vi "Omniax_mDrive_XYZR_MM_BR_RES_2_NC_GR_pxi_Acc2.vi"() -> ()   [LabVIEW 2009]
uses:
  <vilib>/Instr/_visa.llb/VISA Configure Serial Port (Instr).vi
panel:
  in  "Clear ZY":bool
  out "atan Y/Z":dbl
  out "ZY Graph":cluster{"Y":dbl[], "Y":dbl[]}[](graph)
  out "R Ready":bool
  out "Z Ready":bool
  out "Y Ready":bool
  out "X Ready":bool
  out "ZR Graph":cluster{"Y":dbl[], "Y":dbl[]}[](graph)
  out "XY Graph":cluster{"Y":dbl[], "Y":dbl[]}[](graph)
  out "X Scan Duration":dbl
  out "Y Scan Duration":dbl
  out "Z Scan Duration":dbl
  out "R Scan Duration":dbl
  out "R Backlash steps/sec":i32
  out "R Backlash":i32
  out "R Holding Current %":i32
  out "R Run Current %":i32
  out "R offset deg":dbl
  out "R deg/rev":dbl
  out "R steps/rev":u32
  out "R velocity PV step/sec":i32
  out "R MINPOS":i32=-94296
  out "R MAXPOS":i32=-34296
  out "R COM PORT":refnum<visa-resource-name>="COM5"
  in  "R Scan set":bool
  in  "R Scan Velocity SP deg/sec":dbl
  in  "R Scan Length SP deg":dbl
  in  "R Move Set":bool
  out "Reset R Motor Steps":i32
  in  "Reset R Position deg":dbl
  out "R Velocity MVdeg/sec":dbl
  in  "R Velocity SP deg/sec":dbl
  in  "R Position SP deg":dbl
  out "R Position MV deg":dbl
  out "R Scan velocity MV deg/sec":dbl format="%#_6f"
  out "R Scan length MV deg":dbl
  in  "R Scan Length SP steps":i32 min=-6144000 max=0 step=100
  in  "R Scan OK":bool
  in  "R Velocity SP step/sec":i32 min=1 max=20000
  in  "R Scan Velocity SP steps/sec":i32=1 min=1 max=102400 step=1
  in  "R Go":bool
  in  "R Step SP":i32=-20000 min=-6144000 max=0 step=500
  out "R Position deg PV":dbl
  out "R Step PV":i32 max=2000
  out "R Backlash corr":bool
  out "R in Motion":bool
  out "R Scan":bool
  out "R in Range":bool
  out "Z COM PORT":refnum<visa-resource-name>="COM5"
  out "Z Backlash steps/sec":i32
  out "Z Backlash":i32
  out "Z Holding Current %":i32
  out "Z Run Current %":i32
  out "Z offset mm":dbl
  out "Z mm/rev":dbl
  out "Z steps/rev":u32
  out "Z  velocity PV step/sec":i32
  out "Z MINPOS":i32=-94296
  out "Z MAXPOS":i32=-34296
  in  "Z Scan set":bool
  in  "Z Scan Velocity SP mm/sec":dbl
  in  "Z Scan Length SP mm":dbl
  in  "Z Move Set":bool
  out "Reset Z Motor Steps":i32
  in  "Reset Z Position mm":dbl
  out "Z Velocity MV mm/sec":dbl
  in  "Z Velocity SP mm/sec":dbl
  in  "Z Position SP mm":dbl
  out "Z Position MV mm":dbl
  out "Z Scan velocity MV mm/sec":dbl format="%#_6f"
  out "Z Scan length MV mm":dbl
  in  "Z Scan Length SP steps":i32 min=-11520000 max=90880000 step=100
  in  "Z Scan OK":bool
  in  "Z Velocity SP step/sec":i32 min=1 max=204800
  in  "Z Scan Velocity SP steps/sec":i32=1 min=1 max=102400 step=1
  in  "Z Go":bool
  in  "Z Step SP":i32=-20000 min=0 max=102400000 step=500
  out "Z Position mm PV":dbl
  out "Z Step PV":i32 max=2000
  out "Z Backlash corr":bool
  out "Z in Motion":bool
  out "Z Scan":bool
  out "Z in Range":bool
  out "Reset X Motor Steps":i32
  in  "Reset X Position mm":dbl
  out "X Backlash corr":bool
  out "X  in Motion":bool
  out "X Scan":bool
  out "X  in Range":bool
  out "X Step PV":i32 max=2000
  out "X Position mm PV":dbl
  out "X velocity PV step/sec":i32
  in  "X Scan set":bool
  in  "X Scan Velocity SP mm/sec":dbl
  in  "X Scan Length SP mm":dbl
  in  "X Move Set":bool
  out "X Velocity MV mm/sec":dbl
  in  "X Velocity SP mm/sec":dbl
  in  "X Position SP mm":dbl
  out "X Position MV mm":dbl
  out "X Scan velocity MV mm/sec":dbl format="%#_6f"
  out "X Scan length MV mm":dbl
  in  "X Scan Length SP steps":i32 min=-2304000 max=2304000 step=100
  in  "X Scan OK":bool
  in  "X Velocity SP step/sec":i32 min=1 max=128000
  in  "X Scan Velocity SP steps/sec":i32=1 min=1 max=102400 step=1
  in  "X Go":bool
  in  "X Step SP":i32=-20000 min=-2304000 max=2304000 step=500
  out "X Backlash steps/sec":i32
  out "X Backlash":i32
  out "X Holding Current %":i32
  out "X Run Current %":i32
  out "X offset mm":dbl
  out "X mm/rev":dbl
  out "X steps/rev":u32
  out "X MAXPOS":i32=-34296
  out "X MINPOS":i32=-94296
  out "X COM PORT":refnum<visa-resource-name>="COM5"
  out "Y Backlash corr":bool
  in  "Y Scan set":bool
  in  "Y Scan Velocity SP mm/sec":dbl
  in  "Y Scan Length SP mm":dbl
  in  "Y Move Set":bool
  out "Y Backlash steps/sec":i32
  out "Y Backlash":i32
  out "Y in Motion":bool
  in  "Reset":bool
  out "Reset Y Motor Steps":i32
  in  "Reset Y Position mm":dbl
  out "Y Velocity MV mm/sec":dbl
  in  "Y Velocity SP mm/sec":dbl
  in  "Y Position SP mm":dbl
  out "Y Position MV mm":dbl
  out "Y Holding Current %":i32
  out "Y Run Current %":i32
  out "Y Scan velocity MV mm/sec":dbl format="%#_6f"
  out "Y Scan length MV mm":dbl
  in  "Scan Cancel":bool
  out "Y Position mm PV":dbl
  out "Y offset mm":dbl
  out "Y mm/rev":dbl
  out "Y steps/rev":u32
  out "Y velocity PV step/sec":i32
  in  "Y Scan Length SP steps":i32 min=-1792000 max=2816000 step=100
  out "Y Scan":bool
  in  "Y Scan OK":bool
  in  "Scan Go":bool
  in  "Y Velocity SP step/sec":i32 min=1 max=128000
  in  "Y Scan Velocity SP steps/sec":i32=1 min=1 max=102400 step=1
  in  "Stop":bool
  out "Y in Range":bool
  out "Y Step PV":i32 max=2000
  in  "Y Go":bool
  in  "Y Step SP":i32=-20000 min=-2304000 max=2304000 step=500
  out "Y MINPOS":i32=-94296
  out "Y MAXPOS":i32=-34296
  out "Y COM PORT":refnum<visa-resource-name>="COM5"
  # "L"
  # "M"
  # "B"
  # "S"
  # "R"
  # "MX"
  # "MY"
  # "MZ"
  # "MR"
  # "MX"
  # "MY"
  # "MZ"
  # "MR"
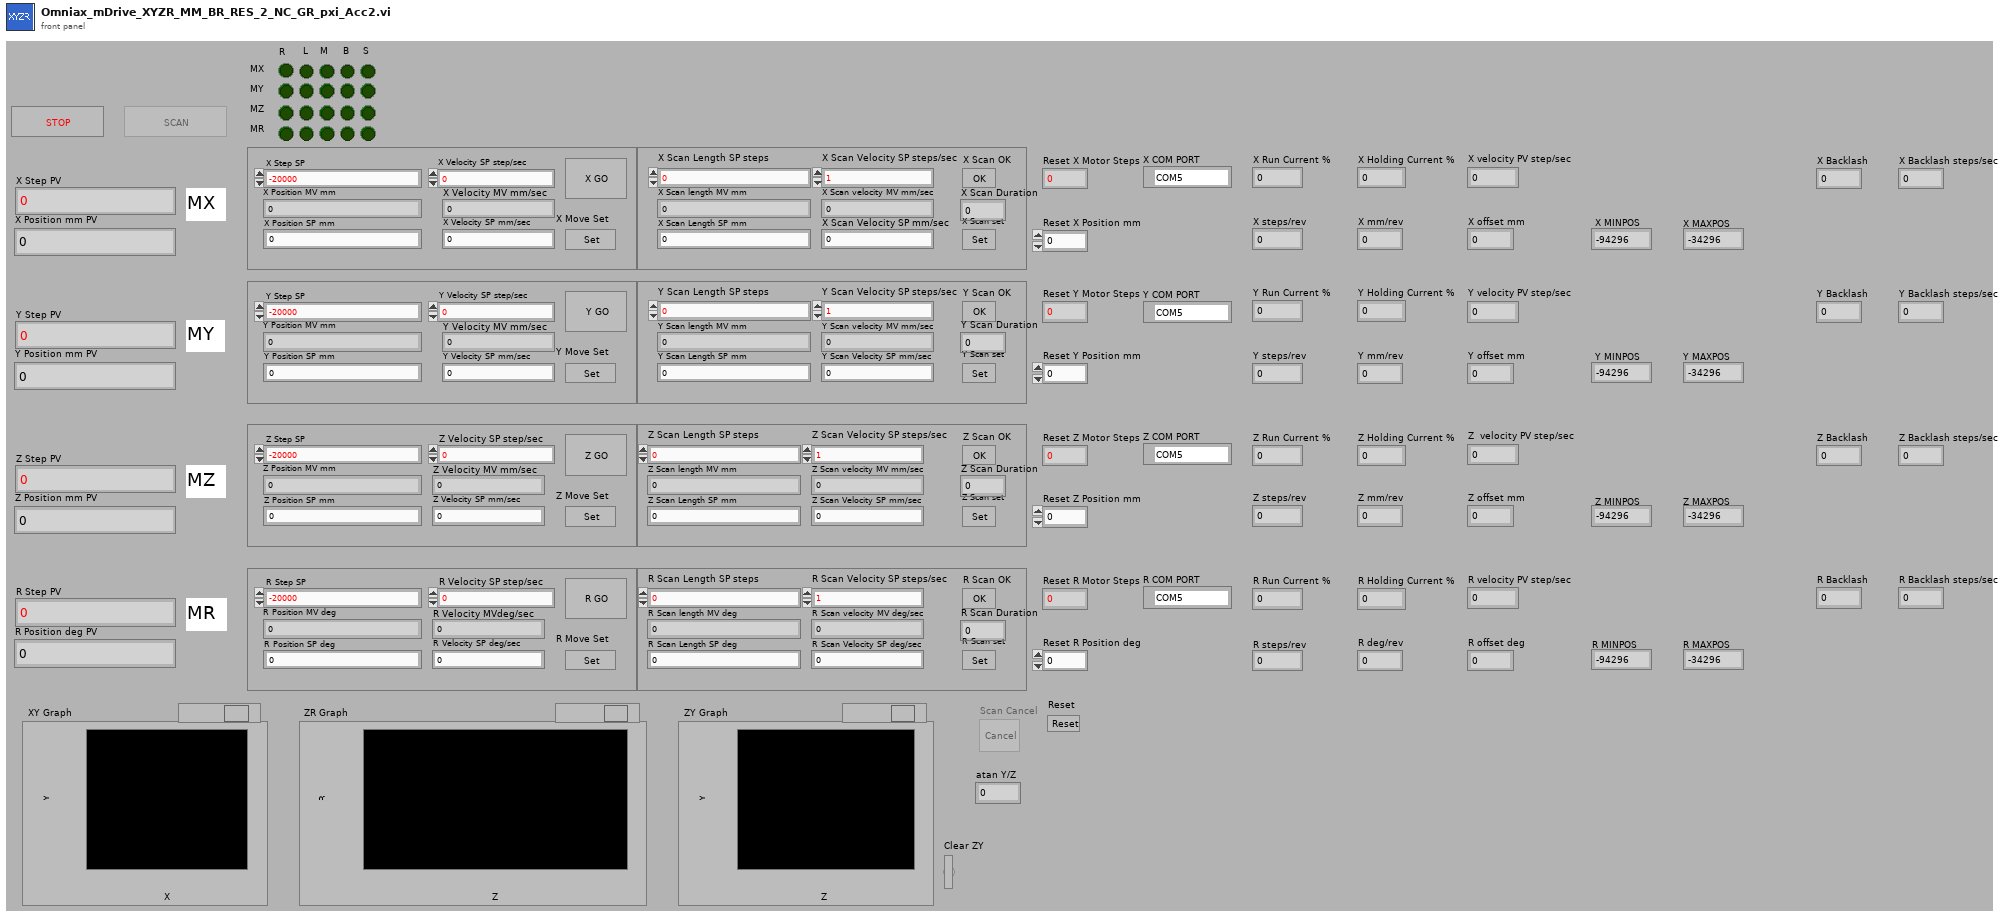
[diagram p1: front panel]
types:
  T1 = enum16{"Stop", "Reset", "Run Current", "Holding Current", "Accel Rate", "Decel Rate", "Move to Relative Position", "Move to Absolute Position", "Echo Mode", "Print Parameter", "Send String", "Microstep Resolution", "Set Current Position", "Max Velocity"}
  T2 = enum8{"Enabled", "Disabled", "Disabled and Grayed Out"}
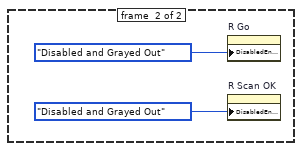
[diagram p2: hidden frame]
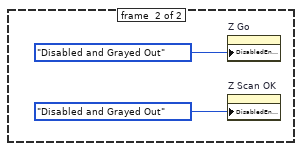
[diagram p5: hidden frame]
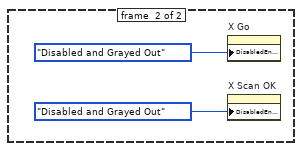
[diagram p8: hidden frame]
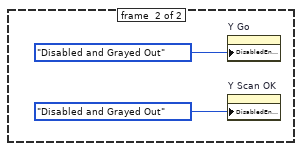
[diagram p11: hidden frame]
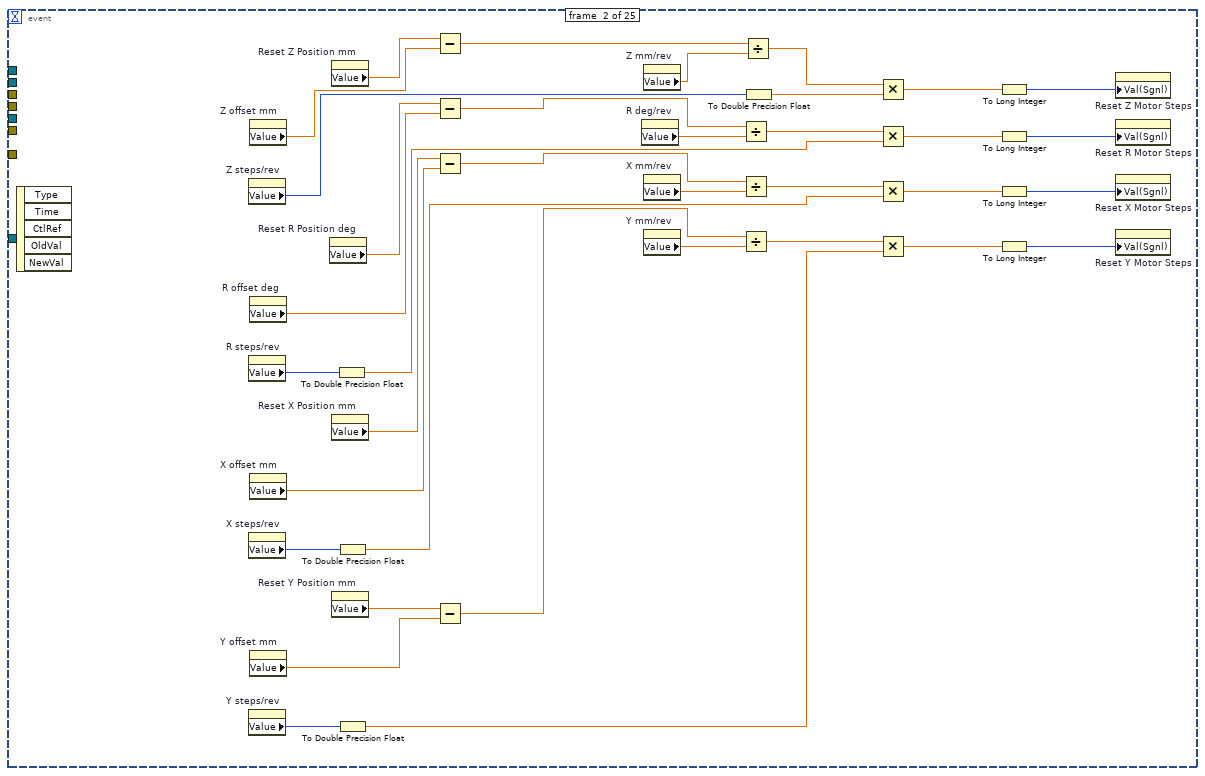
[diagram p14: hidden frame]
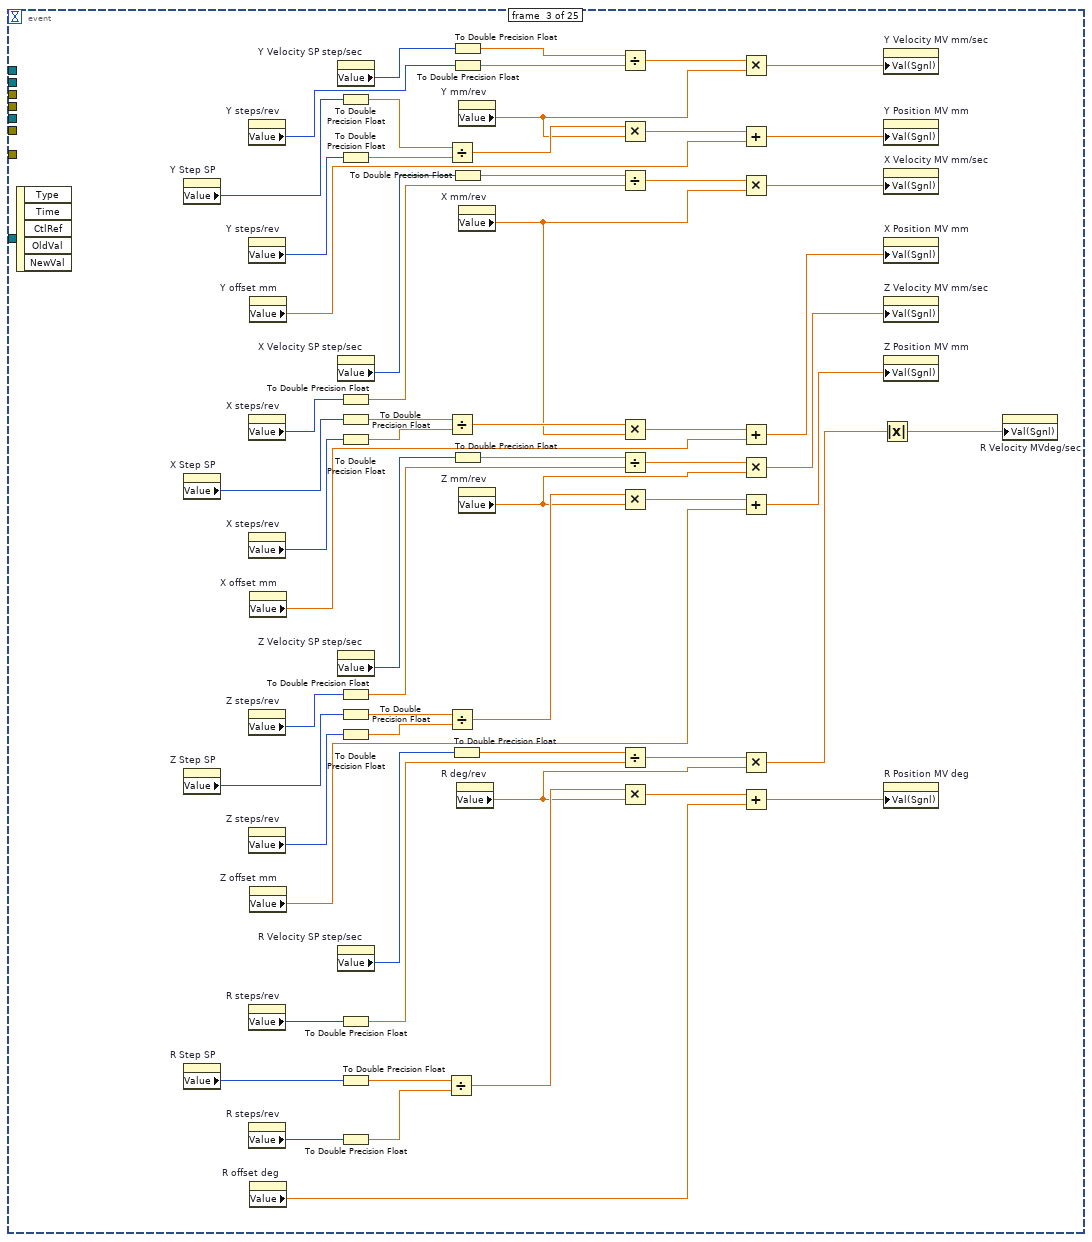
[diagram p15: hidden frame]
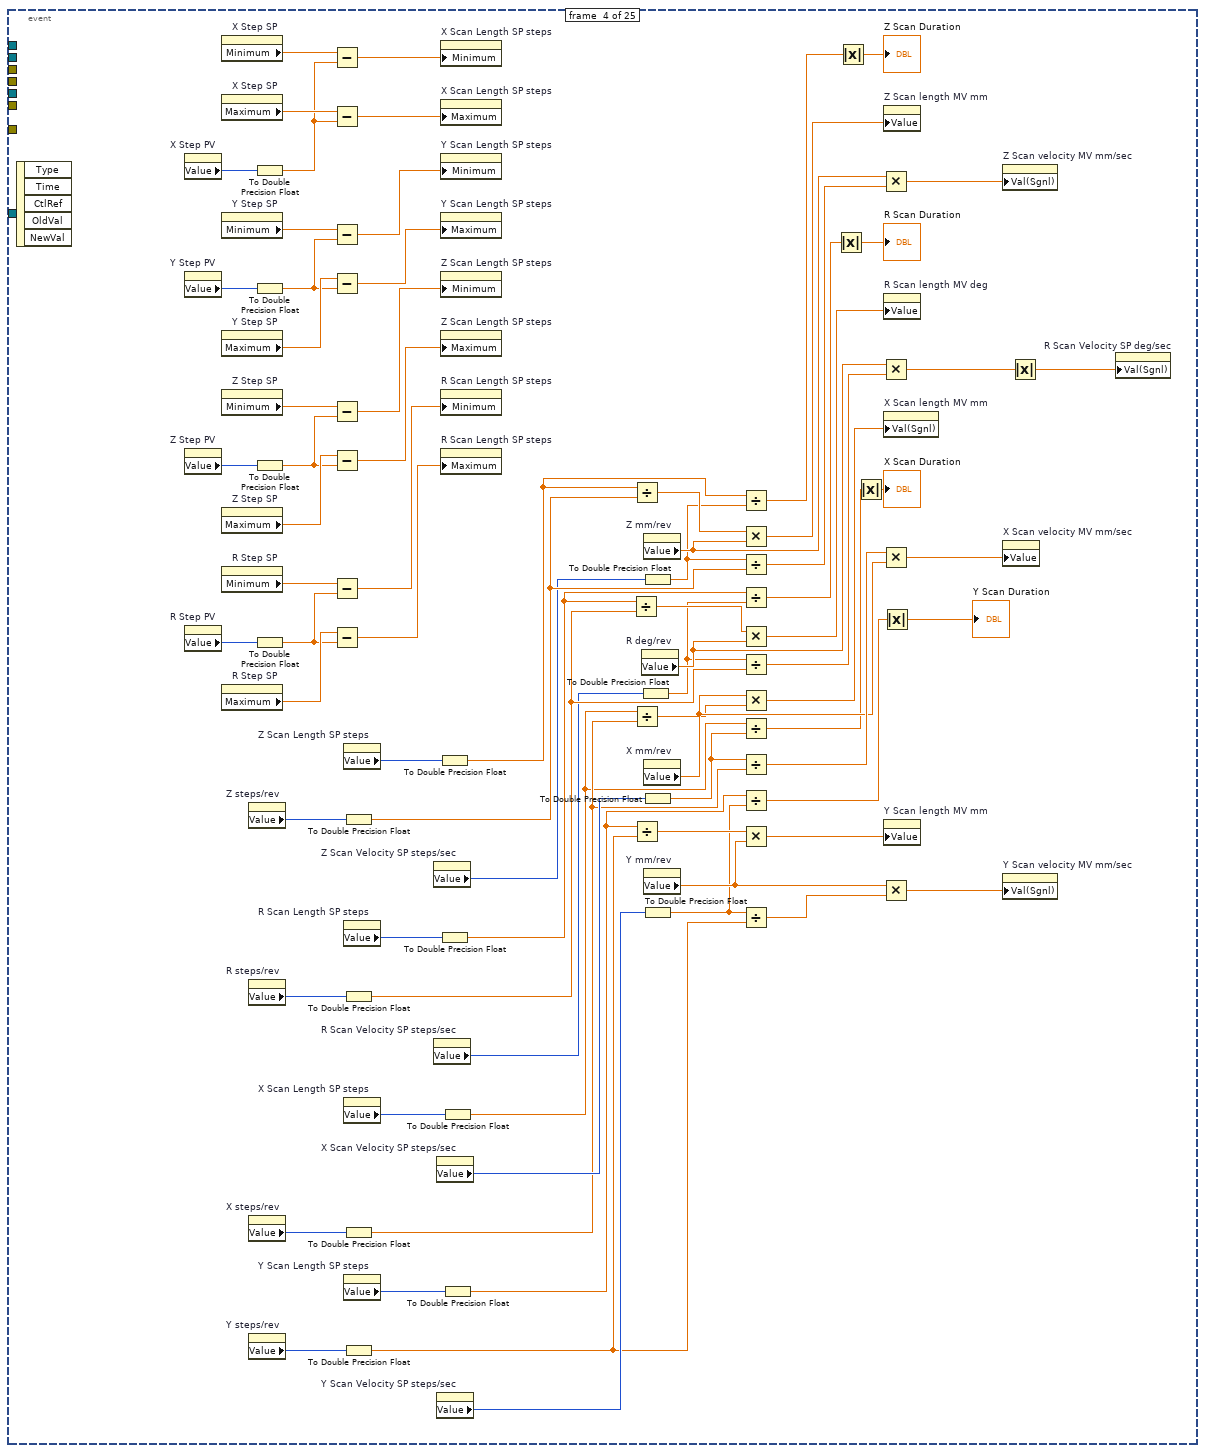
[diagram p16: hidden frame]
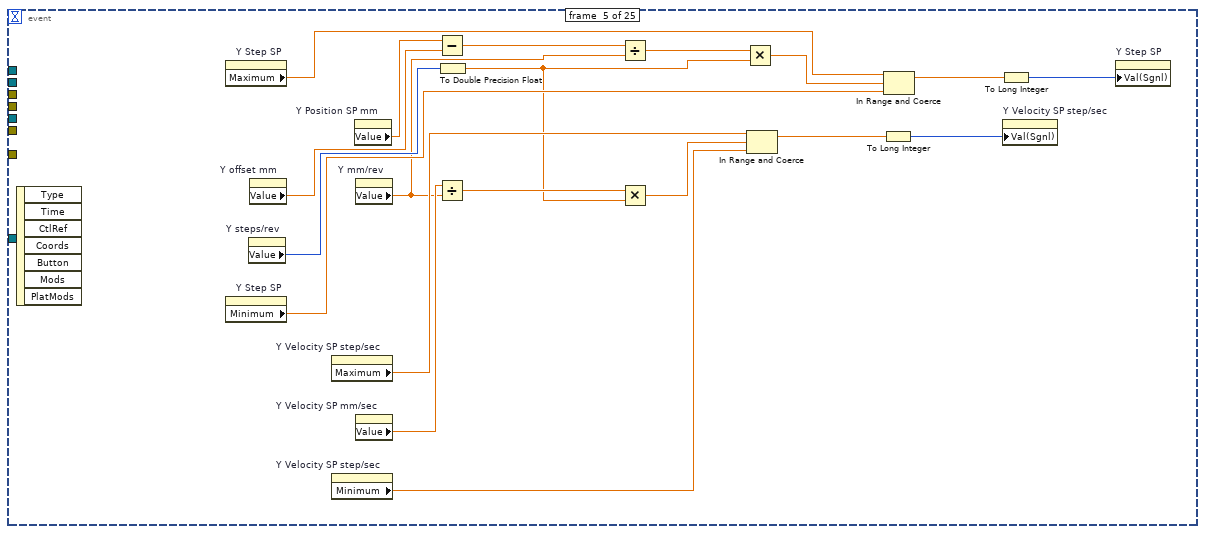
[diagram p17: hidden frame]
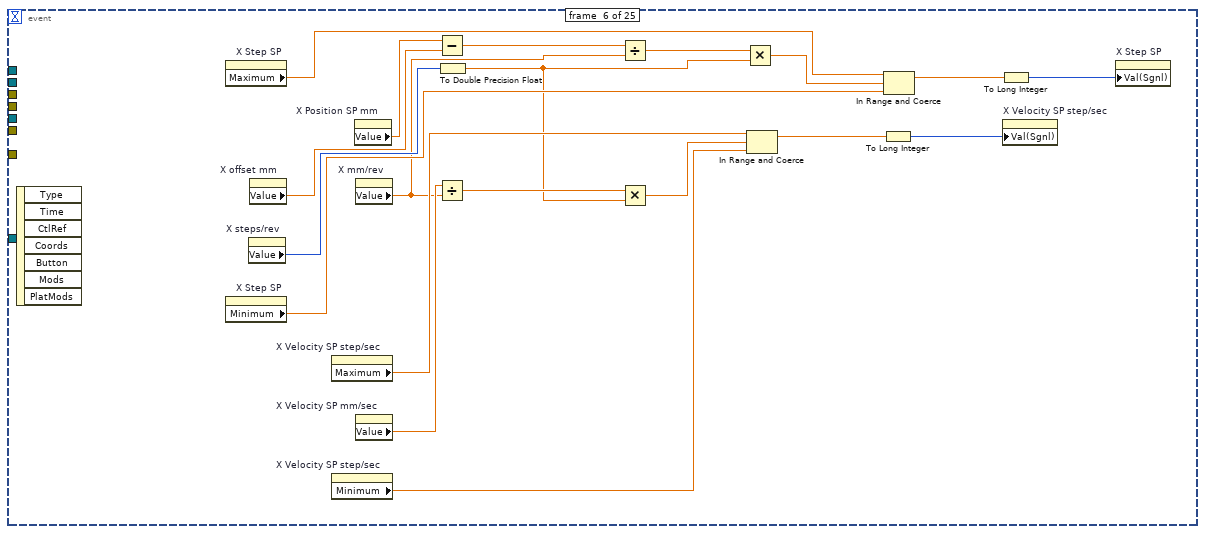
[diagram p18: hidden frame]
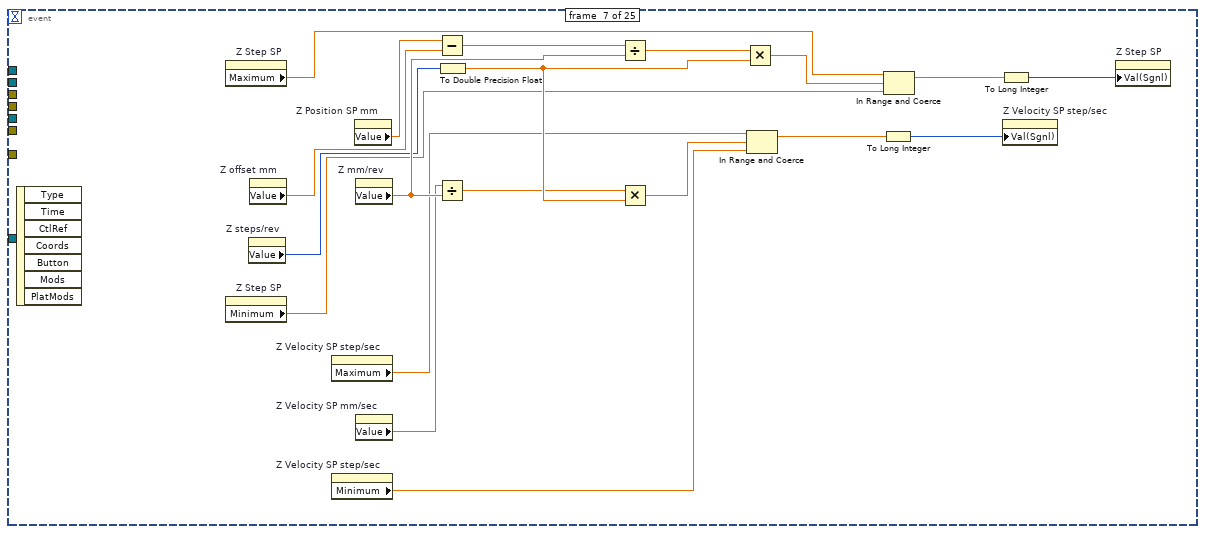
[diagram p19: hidden frame]
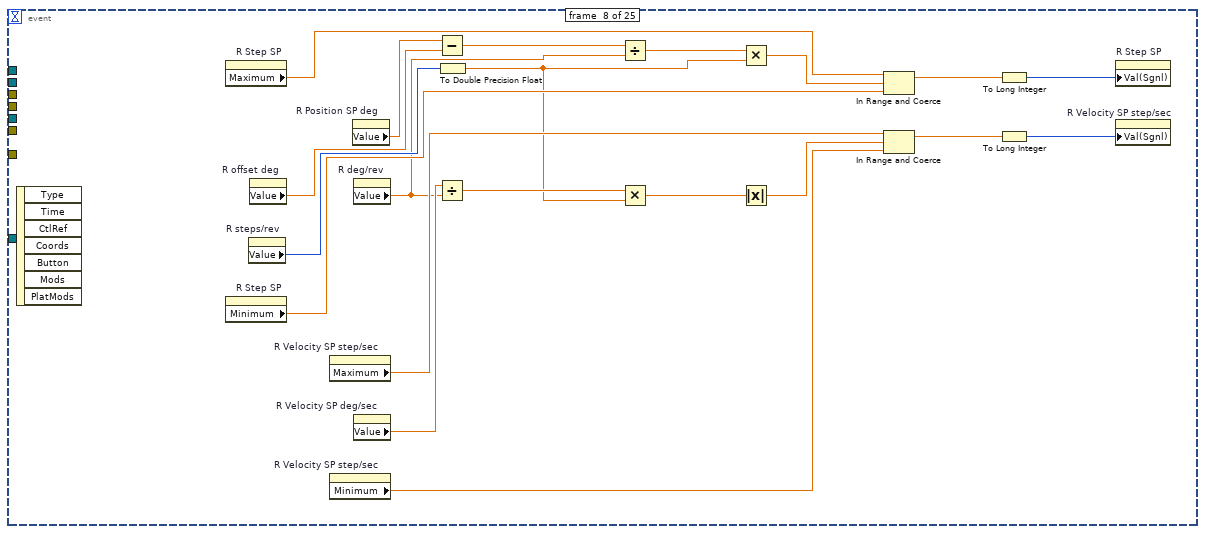
[diagram p20: hidden frame]
diagram:
  n1 = flat-sequence {
    frame #0 {
      w83 = 0.2 ("MM/rev")
      w86 = u32 51200 ("step/rev")
      w81 = 128000 ("Value (Signaling)")
      n2 = To Double Precision Float(number=w81) -> (double precision float=w87:dbl)
      n3 = To Double Precision Float(number=w86) -> (double precision float=w85:dbl)
      n4 = property on="Y Velocity SP step/sec" class="DigNum (strict)"("Minimum"=1.0 ("Data Entry Limits:Minimum")) -> ()  [unwired: 2 in, 2 out]
      n5 = property on="Y Velocity SP step/sec" class="DigNum (strict)"("Val(Sgnl)"=w81) -> ()  [unwired: 2 in, 2 out]
      n6 = Divide(x=w87, y=w85) -> (x/y=w82:dbl)
      n7 = property on="Y Velocity SP step/sec" class="DigNum (strict)"("Maximum"=w87) -> ()  [unwired: 2 in, 2 out]
      n8 = Multiply(x=w82, y=w83) -> (x*y=w84:dbl)
      n9 = property on="Y Velocity SP mm/sec" class="DigNum (strict)"("Val(Sgnl)"=w84) -> ()  [unwired: 2 in, 2 out]
      "Y offset mm" <- 0.0 ("offset")
      "Y steps/rev" <- w86
      "Y mm/rev" <- w83
    }
  }
  n10 = flat-sequence {
    tunnel: [w91] -> w6
    tunnel: [w90] -> w5
    tunnel: [w99] -> w24
    tunnel: [w101] -> w22
    tunnel: w6 -> [w100]
    tunnel: w5 -> [w102]
    tunnel: w24 -> [w106]
    tunnel: [w107] -> w23
    tunnel: w22 -> [w105]
    tunnel: [w108] -> w21
    tunnel: [w119] -> w45
    tunnel: [w121] -> w44
    tunnel: w23 -> [w120]
    tunnel: w21 -> [w115]
    tunnel: w45 -> [w128]
    tunnel: [w127] -> w43
    tunnel: w44 -> [w125]
    tunnel: [w126] -> w42
    tunnel: [w138] -> w41
    tunnel: [w139] -> w40
    tunnel: w43 -> [w137]
    tunnel: w42 -> [w136]
    tunnel: w41 -> [w149]
    tunnel: w40 -> [w148]
    tunnel: [w151] -> w39
    tunnel: [w150] -> w38
    tunnel: [w145] -> w37
    tunnel: [w158] -> w31
    tunnel: [w159] -> w32
    tunnel: w39 -> [w159]
    tunnel: w38 -> [w158]
    tunnel: w37 -> [w156]
    frame #0 {
      w98 = refnum<visa-resource-name> "COM7" ("COM PORT")
      w96 = u16 0 items=["None", "XON/XOFF", "RTS/CTS", "XON/XOFF & RTS/CTS", "DTR/DSR", "XON/XOFF & DTR/DSR"] ("flow control (0:none)")
      w95 = u16 10 items=["1.0"=10, "1.5"=15, "2.0"=20] ("stop bits (10: 1 bit)")
      # "Stop bits"
      n11 = call-poly "VISA Configure Serial Port"("VISA resource name"=w98, "timeout (10sec)"=u32 10000, "baud rate (9600)"=u32 9600, "data bits (8)"=u16 8, "parity (0:none)"=enum16{"None", "Odd", "Even", "Mark", "Space"}."None", "stop bits (10: 1 bit)"=w95, "flow control (0:none)"=w96) -> ("VISA resource name out"=w91:refnum<visa-resource-name>, "error out"=w90:errorcluster)  [unwired: 7 in]
      "R COM PORT" <- w98
    }
    frame #1 {
      n12 = call "mDrive Send Command.vi"("error in (no error)"=w102, "Extra"="EM=2", "Command"=T1."Send String", "VISA resource name"=w100) -> ("error out"=w101:errorcluster, "VISA resource name out"=w99:refnum<visa-resource-name>)  [unwired: 3 in, 1 out]
    }
    frame #2 {
      # "pr=1000000"
      n13 = Number To Decimal String(number=100000) -> (decimal integer string=w110:string)  [unwired: 1 in]
      n14 = call "mDrive Send Command.vi"("error in (no error)"=w105, "Extra"=w110, "Command"=T1."Accel Rate", "VISA resource name"=w106) -> ("error out"=w109:errorcluster, "VISA resource name out"=w114:refnum<visa-resource-name>)  [unwired: 3 in, 1 out]
      n15 = call "mDrive Send Command.vi"("error in (no error)"=w109, "Extra"=w110, "Command"=T1."Decel Rate", "VISA resource name"=w114) -> ("error out"=w108:errorcluster, "VISA resource name out"=w107:refnum<visa-resource-name>)  [unwired: 3 in, 1 out]
    }
    frame #3 {
      # "Run Current %"
      n16 = property on="R Run Current %" class="DigNum (strict)"() -> ("Value"=w117:i32)  [unwired: 2 in, 2 out]
      n17 = Number To Decimal String(number=w117) -> (decimal integer string=w118:string)  [unwired: 1 in]
      n18 = call "mDrive Send Command.vi"("error in (no error)"=w115, "Extra"=w118, "Command"=T1."Run Current", "VISA resource name"=w120) -> ("error out"=w121:errorcluster, "VISA resource name out"=w119:refnum<visa-resource-name>)  [unwired: 3 in, 1 out]
    }
    frame #4 {
      # "Holding Current %"
      n19 = property on="R Holding Current %" class="DigNum (strict)"() -> ("Value"=w123:i32)  [unwired: 2 in, 2 out]
      n20 = Number To Decimal String(number=w123) -> (decimal integer string=w124:string)  [unwired: 1 in]
      n21 = call "mDrive Send Command.vi"("error in (no error)"=w125, "Extra"=w124, "Command"=T1."Holding Current", "VISA resource name"=w128) -> ("error out"=w126:errorcluster, "VISA resource name out"=w127:refnum<visa-resource-name>)  [unwired: 3 in, 1 out]
    }
    frame #5 {
      # "Print Velocity Max"
      # "Velocity Max"
      n22 = property on="R Velocity SP step/sec" class="DigNum (strict)"() -> ("Value"=w135:i32)  [unwired: 2 in, 2 out]
      n23 = Number To Decimal String(number=w135) -> (decimal integer string=w134:string)  [unwired: 1 in]
      n24 = call "mDrive Send Command.vi"("error in (no error)"=w136, "Extra"=w134, "Command"=T1."Max Velocity", "VISA resource name"=w137) -> ("error out"=w132:errorcluster, "VISA resource name out"=w142:refnum<visa-resource-name>)  [unwired: 3 in, 1 out]
      n25 = call "mDrive Send Command.vi"("error in (no error)"=w132, "Extra"="VM", "Command"=T1."Print Parameter", "VISA resource name"=w142) -> ("error out"=w139:errorcluster, "read buffer"=w140:string, "VISA resource name out"=w138:refnum<visa-resource-name>)  [unwired: 3 in]
      n26 = Decimal String To Number(string=w140, offset=0) -> (number=w133:i32)  [unwired: 1 in, 1 out]
      n27 = property on="R velocity PV step/sec" class="DigNum (strict)"("Val(Sgnl)"=w133) -> ()  [unwired: 2 in, 2 out]
    }
    frame #6 {
      # "PRINT POSITION"
      n28 = call "mDrive Send Command.vi"("error in (no error)"=w148, "Extra"="P", "Command"=T1."Print Parameter", "VISA resource name"=w149) -> ("error out"=w150:errorcluster, "read buffer"=w147:string, "VISA resource name out"=w151:refnum<visa-resource-name>)  [unwired: 3 in]
      n29 = Decimal String To Number(string=w147, offset=0) -> (number=w145:i32)  [unwired: 1 in, 1 out]
    }
    frame #7 {
      n30 = property on="R Step SP" class="DigNum (strict)"("Val(Sgnl)"=w156) -> ()  [unwired: 2 in, 2 out]
      n31 = property on="R Step SP" class="DigNum (strict)"() -> ("Maximum"=w155:dbl)  [unwired: 2 in, 2 out]
      n32 = To Long Integer(number=w155) -> (32bit integer=w152:i32)
      "R MAXPOS" <- w152
      n33 = property on="R Step SP" class="DigNum (strict)"() -> ("Minimum"=w154:dbl)  [unwired: 2 in, 2 out]
      n34 = To Long Integer(number=w154) -> (32bit integer=w153:i32)
      "R MINPOS" <- w153
      n35 = In Range and Coerce(upper limit=w152, x=w156, lower limit=w153) -> (In Range?=w157:bool)  [unwired: 1 out]
      n36 = property on="R in Range" class="Bool (strict)"("Val(Sgnl)"=w157) -> ()  [unwired: 2 in, 2 out]
    }
  }
  n37 = flat-sequence {
    tunnel: [w160] -> w10
    tunnel: [w161] -> w9
    tunnel: [w171] -> w16
    tunnel: [w170] -> w14
    tunnel: w10 -> [w172]
    tunnel: w9 -> [w169]
    tunnel: w16 -> [w182]
    tunnel: [w177] -> w15
    tunnel: w14 -> [w181]
    tunnel: [w181] -> w13
    tunnel: [w186] -> w54
    tunnel: [w188] -> w53
    tunnel: w15 -> [w187]
    tunnel: w13 -> [w189]
    tunnel: w54 -> [w196]
    tunnel: [w195] -> w52
    tunnel: w53 -> [w193]
    tunnel: [w194] -> w51
    tunnel: [w206] -> w50
    tunnel: [w207] -> w49
    tunnel: w52 -> [w205]
    tunnel: w51 -> [w204]
    tunnel: w50 -> [w217]
    tunnel: w49 -> [w216]
    tunnel: [w219] -> w48
    tunnel: [w218] -> w47
    tunnel: [w213] -> w46
    tunnel: [w226] -> w35
    tunnel: [w227] -> w36
    tunnel: w48 -> [w227]
    tunnel: w47 -> [w226]
    tunnel: w46 -> [w224]
    frame #0 {
      w168 = refnum<visa-resource-name> "COM6" ("COM PORT")
      w166 = u16 0 items=["None", "XON/XOFF", "RTS/CTS", "XON/XOFF & RTS/CTS", "DTR/DSR", "XON/XOFF & DTR/DSR"] ("flow control (0:none)")
      w165 = u16 10 items=["1.0"=10, "1.5"=15, "2.0"=20] ("stop bits (10: 1 bit)")
      # "Stop bits"
      n38 = call-poly "VISA Configure Serial Port"("VISA resource name"=w168, "timeout (10sec)"=u32 10000, "baud rate (9600)"=u32 9600, "data bits (8)"=u16 8, "parity (0:none)"=enum16{"None", "Odd", "Even", "Mark", "Space"}."None", "stop bits (10: 1 bit)"=w165, "flow control (0:none)"=w166) -> ("VISA resource name out"=w160:refnum<visa-resource-name>, "error out"=w161:errorcluster)  [unwired: 7 in]
      "Z COM PORT" <- w168
    }
    frame #1 {
      n39 = call "mDrive Send Command.vi"("error in (no error)"=w169, "Extra"="EM=2", "Command"=T1."Send String", "VISA resource name"=w172) -> ("error out"=w170:errorcluster, "VISA resource name out"=w171:refnum<visa-resource-name>)  [unwired: 3 in, 1 out]
    }
    frame #2 {
      n40 = Number To Decimal String(number=1000000) -> (decimal integer string=w175:string)  [unwired: 1 in]
      n41 = call "mDrive Send Command.vi"("Extra"=w175, "Command"=T1."Accel Rate", "VISA resource name"=w182) -> ("VISA resource name out"=w180:refnum<visa-resource-name>)  [unwired: 4 in, 2 out]
      n42 = call "mDrive Send Command.vi"("Extra"=w175, "Command"=T1."Decel Rate", "VISA resource name"=w180) -> ("VISA resource name out"=w177:refnum<visa-resource-name>)  [unwired: 4 in, 2 out]
    }
    frame #3 {
      # "Run Current %"
      n43 = property on="Z Run Current %" class="DigNum (strict)"() -> ("Value"=w184:i32)  [unwired: 2 in, 2 out]
      n44 = Number To Decimal String(number=w184) -> (decimal integer string=w185:string)  [unwired: 1 in]
      n45 = call "mDrive Send Command.vi"("error in (no error)"=w189, "Extra"=w185, "Command"=T1."Run Current", "VISA resource name"=w187) -> ("error out"=w188:errorcluster, "VISA resource name out"=w186:refnum<visa-resource-name>)  [unwired: 3 in, 1 out]
    }
    frame #4 {
      # "Holding Current %"
      n46 = property on="Z Run Current %" class="DigNum (strict)"() -> ("Value"=w191:i32)  [unwired: 2 in, 2 out]
      n47 = Number To Decimal String(number=w191) -> (decimal integer string=w192:string)  [unwired: 1 in]
      n48 = call "mDrive Send Command.vi"("error in (no error)"=w193, "Extra"=w192, "Command"=T1."Holding Current", "VISA resource name"=w196) -> ("error out"=w194:errorcluster, "VISA resource name out"=w195:refnum<visa-resource-name>)  [unwired: 3 in, 1 out]
    }
    frame #5 {
      # "Velocity Max"
      n49 = property on="Z Velocity SP step/sec" class="DigNum (strict)"() -> ("Value"=w203:i32)  [unwired: 2 in, 2 out]
      n50 = Number To Decimal String(number=w203) -> (decimal integer string=w202:string)  [unwired: 1 in]
      n51 = call "mDrive Send Command.vi"("error in (no error)"=w204, "Extra"=w202, "Command"=T1."Max Velocity", "VISA resource name"=w205) -> ("error out"=w200:errorcluster, "VISA resource name out"=w210:refnum<visa-resource-name>)  [unwired: 3 in, 1 out]
      n52 = call "mDrive Send Command.vi"("error in (no error)"=w200, "Extra"="VM", "Command"=T1."Print Parameter", "VISA resource name"=w210) -> ("error out"=w207:errorcluster, "read buffer"=w208:string, "VISA resource name out"=w206:refnum<visa-resource-name>)  [unwired: 3 in]
      n53 = Decimal String To Number(string=w208, offset=0) -> (number=w201:i32)  [unwired: 1 in, 1 out]
      n54 = property on="Z  velocity PV step/sec" class="DigNum (strict)"("Val(Sgnl)"=w201) -> ()  [unwired: 2 in, 2 out]
    }
    frame #6 {
      # "PRINT POSITION"
      n55 = call "mDrive Send Command.vi"("error in (no error)"=w216, "Extra"="P", "Command"=T1."Print Parameter", "VISA resource name"=w217) -> ("error out"=w218:errorcluster, "read buffer"=w215:string, "VISA resource name out"=w219:refnum<visa-resource-name>)  [unwired: 3 in]
      n56 = Decimal String To Number(string=w215, offset=0) -> (number=w213:i32)  [unwired: 1 in, 1 out]
    }
    frame #7 {
      n57 = property on="Z Step SP" class="DigNum (strict)"("Val(Sgnl)"=w224) -> ()  [unwired: 2 in, 2 out]
      n58 = property on="Z Step SP" class="DigNum (strict)"() -> ("Maximum"=w221:dbl)  [unwired: 2 in, 2 out]
      n59 = property on="Z Step SP" class="DigNum (strict)"() -> ("Minimum"=w223:dbl)  [unwired: 2 in, 2 out]
      n60 = To Long Integer(number=w221) -> (32bit integer=w222:i32)
      "Z MAXPOS" <- w222
      n61 = To Long Integer(number=w223) -> (32bit integer=w220:i32)
      "Z MINPOS" <- w220
      n62 = In Range and Coerce(upper limit=w222, x=w224, lower limit=w220) -> (In Range?=w225:bool)  [unwired: 1 out]
      n63 = property on="Z in Range" class="Bool (strict)"("Val(Sgnl)"=w225) -> ()  [unwired: 2 in, 2 out]
    }
  }
  n64 = flat-sequence {
    tunnel: [w229] -> w4
    tunnel: [w228] -> w3
    tunnel: [w239] -> w20
    tunnel: [w237] -> w18
    tunnel: w4 -> [w240]
    tunnel: w3 -> [w238]
    tunnel: w20 -> [w246]
    tunnel: [w247] -> w19
    tunnel: w18 -> [w243]
    tunnel: [w245] -> w17
    tunnel: [w256] -> w74
    tunnel: [w258] -> w72
    tunnel: w19 -> [w257]
    tunnel: w17 -> [w259]
    tunnel: w74 -> [w266]
    tunnel: [w265] -> w73
    tunnel: w72 -> [w263]
    tunnel: [w264] -> w71
    tunnel: [w276] -> w76
    tunnel: [w277] -> w75
    tunnel: w73 -> [w275]
    tunnel: w71 -> [w274]
    tunnel: w76 -> [w287]
    tunnel: w75 -> [w286]
    tunnel: [w289] -> w60
    tunnel: [w288] -> w59
    tunnel: [w283] -> w58
    tunnel: [w294] -> w79
    tunnel: [w295] -> w80
    tunnel: w60 -> [w295]
    tunnel: w59 -> [w294]
    tunnel: w58 -> [w290]
    frame #0 {
      w236 = refnum<visa-resource-name> "COM5" ("COM PORT")
      w234 = u16 0 items=["None", "XON/XOFF", "RTS/CTS", "XON/XOFF & RTS/CTS", "DTR/DSR", "XON/XOFF & DTR/DSR"] ("flow control (0:none)")
      w233 = u16 10 items=["1.0"=10, "1.5"=15, "2.0"=20] ("stop bits (10: 1 bit)")
      # "Stop bits"
      n65 = call-poly "VISA Configure Serial Port"("VISA resource name"=w236, "timeout (10sec)"=u32 10000, "baud rate (9600)"=u32 9600, "data bits (8)"=u16 8, "parity (0:none)"=enum16{"None", "Odd", "Even", "Mark", "Space"}."None", "stop bits (10: 1 bit)"=w233, "flow control (0:none)"=w234) -> ("VISA resource name out"=w229:refnum<visa-resource-name>, "error out"=w228:errorcluster)  [unwired: 7 in]
      "Y COM PORT" <- w236
    }
    frame #1 {
      n66 = call "mDrive Send Command.vi"("error in (no error)"=w238, "Extra"="EM=2", "Command"=T1."Send String", "VISA resource name"=w240) -> ("error out"=w237:errorcluster, "VISA resource name out"=w239:refnum<visa-resource-name>)  [unwired: 3 in, 1 out]
    }
    frame #2 {
      n67 = Number To Decimal String(number=1000000) -> (decimal integer string=w248:string)  [unwired: 1 in]
      n68 = call "mDrive Send Command.vi"("error in (no error)"=w243, "Extra"=w248, "Command"=T1."Accel Rate", "VISA resource name"=w246) -> ("error out"=w244:errorcluster, "VISA resource name out"=w252:refnum<visa-resource-name>)  [unwired: 3 in, 1 out]
      n69 = call "mDrive Send Command.vi"("error in (no error)"=w244, "Extra"=w248, "Command"=T1."Decel Rate", "VISA resource name"=w252) -> ("error out"=w245:errorcluster, "VISA resource name out"=w247:refnum<visa-resource-name>)  [unwired: 3 in, 1 out]
    }
    frame #3 {
      # "Run Current %"
      n70 = property on="Y Run Current %" class="DigNum (strict)"() -> ("Value"=w254:i32)  [unwired: 2 in, 2 out]
      n71 = Number To Decimal String(number=w254) -> (decimal integer string=w255:string)  [unwired: 1 in]
      n72 = call "mDrive Send Command.vi"("error in (no error)"=w259, "Extra"=w255, "Command"=T1."Run Current", "VISA resource name"=w257) -> ("error out"=w258:errorcluster, "VISA resource name out"=w256:refnum<visa-resource-name>)  [unwired: 3 in, 1 out]
    }
    frame #4 {
      # "Holding Current %"
      n73 = property on="Y Holding Current %" class="DigNum (strict)"() -> ("Value"=w261:i32)  [unwired: 2 in, 2 out]
      n74 = Number To Decimal String(number=w261) -> (decimal integer string=w262:string)  [unwired: 1 in]
      n75 = call "mDrive Send Command.vi"("error in (no error)"=w263, "Extra"=w262, "Command"=T1."Holding Current", "VISA resource name"=w266) -> ("error out"=w264:errorcluster, "VISA resource name out"=w265:refnum<visa-resource-name>)  [unwired: 3 in, 1 out]
    }
    frame #5 {
      # "Velocity Max"
      n76 = property on="Y Velocity SP step/sec" class="DigNum (strict)"() -> ("Value"=w273:i32)  [unwired: 2 in, 2 out]
      n77 = Number To Decimal String(number=w273) -> (decimal integer string=w272:string)  [unwired: 1 in]
      n78 = call "mDrive Send Command.vi"("error in (no error)"=w274, "Extra"=w272, "Command"=T1."Max Velocity", "VISA resource name"=w275) -> ("error out"=w270:errorcluster, "VISA resource name out"=w280:refnum<visa-resource-name>)  [unwired: 3 in, 1 out]
      n79 = call "mDrive Send Command.vi"("error in (no error)"=w270, "Extra"="VM", "Command"=T1."Print Parameter", "VISA resource name"=w280) -> ("error out"=w277:errorcluster, "read buffer"=w278:string, "VISA resource name out"=w276:refnum<visa-resource-name>)  [unwired: 3 in]
      n80 = Decimal String To Number(string=w278, offset=0) -> (number=w271:i32)  [unwired: 1 in, 1 out]
      n81 = property on="Y scan velocity MV step/sec" class="DigNum (strict)"("Val(Sgnl)"=w271) -> ()  [unwired: 2 in, 2 out]
    }
    frame #6 {
      # "PRINT POSITION"
      n82 = call "mDrive Send Command.vi"("error in (no error)"=w286, "Extra"="P", "Command"=T1."Print Parameter", "VISA resource name"=w287) -> ("error out"=w288:errorcluster, "read buffer"=w285:string, "VISA resource name out"=w289:refnum<visa-resource-name>)  [unwired: 3 in]
      n83 = Decimal String To Number(string=w285, offset=0) -> (number=w283:i32)  [unwired: 1 in, 1 out]
    }
    frame #7 {
      w292 = -2304000 ("lower limit")
      w293 = 2304000 ("upper limit")
      n84 = property on="Y Step SP" class="DigNum (strict)"("Val(Sgnl)"=w290) -> ()  [unwired: 2 in, 2 out]
      n85 = property on="Y Step SP" class="DigNum (strict)"("Minimum"=w292) -> ()  [unwired: 2 in, 2 out]
      n86 = property on="Y Step SP" class="DigNum (strict)"("Maximum"=w293) -> ()  [unwired: 2 in, 2 out]
      n87 = In Range and Coerce(upper limit=w293, x=w290, lower limit=w292) -> (In Range?=w291:bool)  [unwired: 1 out]
      n88 = property on="Y in Range" class="Bool (strict)"("Val(Sgnl)"=w291) -> ()  [unwired: 2 in, 2 out]
      "Y MINPOS" <- w292
      "Y MAXPOS" <- w293
    }
  }
  n89 = flat-sequence {
    frame #0 {
      w301 = -3.0 ("R deg/rev")
      w299 = u32 51200 ("step/rev")
      w303 = 20000 ("Value (Signaling)")
      n90 = To Double Precision Float(number=w303) -> (double precision float=w305:dbl)
      n91 = To Double Precision Float(number=w299) -> (double precision float=w300:dbl)
      n92 = property on="R Velocity SP step/sec" class="DigNum (strict)"("Val(Sgnl)"=w303) -> ()  [unwired: 2 in, 2 out]
      n93 = property on="R Velocity SP step/sec" class="DigNum (strict)"("Minimum"=1.0 ("Data Entry Limits:Minimum")) -> ()  [unwired: 2 in, 2 out]
      n94 = Divide(x=w305, y=w300) -> (x/y=w304:dbl)
      n95 = property on="R Velocity SP step/sec" class="DigNum (strict)"("Maximum"=w305) -> ()  [unwired: 2 in, 2 out]
      n96 = Multiply(x=w304, y=w301) -> (x*y=w302:dbl)
      n97 = Absolute Value(x=w302) -> (abs(x)=w296:dbl)
      n98 = property on="R Velocity SP deg/sec" class="DigNum (strict)"("Val(Sgnl)"=w296) -> ()  [unwired: 2 in, 2 out]
      "R offset deg" <- 0.0 ("R offset deg")
      "R deg/rev" <- w301
      "R steps/rev" <- w299
    }
  }
  n99 = flat-sequence {
    frame #0 {
      w307 = 0.2 ("Z mm/rev")
      w306 = u32 51200 ("step/rev")
      w308 = 204800 ("Value (Signaling)")
      n100 = To Double Precision Float(number=w308) -> (double precision float=w312:dbl)
      n101 = To Double Precision Float(number=w306) -> (double precision float=w311:dbl)
      n102 = property on="Z Velocity SP step/sec" class="DigNum (strict)"("Val(Sgnl)"=w308) -> ()  [unwired: 2 in, 2 out]
      n103 = property on="Z Velocity SP step/sec" class="DigNum (strict)"("Minimum"=1.0 ("Data Entry Limits:Minimum")) -> ()  [unwired: 2 in, 2 out]
      n104 = Divide(x=w312, y=w311) -> (x/y=w309:dbl)
      n105 = property on="Z Velocity SP step/sec" class="DigNum (strict)"("Maximum"=w312) -> ()  [unwired: 2 in, 2 out]
      n106 = Multiply(x=w309, y=w307) -> (x*y=w310:dbl)
      n107 = property on="Z Velocity SP mm/sec" class="DigNum (strict)"("Val(Sgnl)"=w310) -> ()  [unwired: 2 in, 2 out]
      "Z offset mm" <- 0.0 ("Z offset mm")
      "Z mm/rev" <- w307
      "Z steps/rev" <- w306
    }
  }
  n108 = flat-sequence {
    frame #0 {
      n109 = property on="R Backlash corr" class="Bool (strict)"("Val(Sgnl)"=FALSE ("Value (Signaling)")) -> ()  [unwired: 2 in, 2 out]
      n110 = property on="Y Backlash corr" class="Bool (strict)"("Val(Sgnl)"=FALSE ("Value (Signaling)")) -> ()  [unwired: 2 in, 2 out]
      n111 = property on="Z Backlash corr" class="Bool (strict)"("Val(Sgnl)"=FALSE ("Value (Signaling)")) -> ()  [unwired: 2 in, 2 out]
      n112 = property on="X Backlash corr" class="Bool (strict)"("Val(Sgnl)"=FALSE ("Value (Signaling)")) -> ()  [unwired: 2 in, 2 out]
      "Z Backlash steps/sec" <- 25600 ("Z Backlash steps/sec")
      "Z Backlash" <- -12800 ("Z Backlash")
      "X Backlash steps/sec" <- 25600 ("Value (Signaling)")
      "X Backlash" <- 5120 ("Backlash2")
      "Y Backlash" <- 5120 ("Backlash2")
      "Y Backlash steps/sec" <- 25600 ("Value (Signaling)")
      "R Backlash steps/sec" <- 6400 ("R Backlash steps/sec")
      "R Backlash" <- -12800 ("R Backlash")
    }
  }
  n113 = flat-sequence {
    frame #0 {
      "Z Holding Current %" <- 20 ("Z Holding Current %")
      "Z Run Current %" <- 40 ("Z Run Current %")
      "X Run Current %" <- 40 ("Run Current %")
      "X Holding Current %" <- 20 ("Holding Current %")
      "Y Run Current %" <- 40 ("Run Current %")
      "Y Holding Current %" <- 20 ("Holding Current %")
      "R Holding Current %" <- 20 ("R Holding Current %")
      "R Run Current %" <- 100 ("R Run Current %")
    }
  }
  n114 = flat-sequence {
    frame #0 {
      n115 = property on="Z Scan" class="Bool (strict)"("Val(Sgnl)"=FALSE ("Value (Signaling)")) -> ()  [unwired: 2 in, 2 out]
      n116 = property on="R Velocity SP deg/sec" class="DigNum (strict)"("Val(Sgnl)"=0.1 ("Value (Signaling)")) -> ()  [unwired: 2 in, 2 out]
      n117 = property on="Z Scan Velocity SP mm/sec" class="DigNum (strict)"("Val(Sgnl)"=0.1 ("Value (Signaling)")) -> ()  [unwired: 2 in, 2 out]
      n118 = property on="X Scan" class="Bool (strict)"("Val(Sgnl)"=FALSE ("Value (Signaling)")) -> ()  [unwired: 2 in, 2 out]
      n119 = property on="R Scan" class="Bool (strict)"("Val(Sgnl)"=FALSE ("Value (Signaling)")) -> ()  [unwired: 2 in, 2 out]
      n120 = property on="Y Scan Velocity SP mm/sec" class="DigNum (strict)"("Val(Sgnl)"=0.1 ("Value (Signaling)")) -> ()  [unwired: 2 in, 2 out]
      n121 = property on="Y Scan" class="Bool (strict)"("Val(Sgnl)"=FALSE ("Value (Signaling)")) -> ()  [unwired: 2 in, 2 out]
      n122 = property on="X Scan Velocity SP mm/sec" class="DigNum (strict)"("Val(Sgnl)"=0.1 ("Value (Signaling)")) -> ()  [unwired: 2 in, 2 out]
      n123 = property on="Scan Go" class="Bool"("DisabledEnum"=T2."Disabled and Grayed Out" ("Disabled")) -> ()  [unwired: 2 in, 2 out]
      n124 = property on="Scan Cancel" class="Bool"("DisabledEnum"=T2."Disabled and Grayed Out" ("Disabled")) -> ()  [unwired: 2 in, 2 out]
    }
  }
  n125 = flat-sequence {
    frame #0 {
      w347 = 0.2 ("MM/rev")
      w350 = u32 51200 ("step/rev")
      w345 = 128000 ("Value (Signaling)")
      # "a=1000000"
      n126 = property on="X Velocity SP step/sec" class="DigNum (strict)"("Minimum"=1.0 ("Data Entry Limits:Minimum")) -> ()  [unwired: 2 in, 2 out]
      n127 = To Double Precision Float(number=w345) -> (double precision float=w351:dbl)
      n128 = To Double Precision Float(number=w350) -> (double precision float=w349:dbl)
      n129 = property on="X Velocity SP step/sec" class="DigNum (strict)"("Val(Sgnl)"=w345) -> ()  [unwired: 2 in, 2 out]
      n130 = Divide(x=w351, y=w349) -> (x/y=w346:dbl)
      n131 = property on="X Velocity SP step/sec" class="DigNum (strict)"("Maximum"=w351) -> ()  [unwired: 2 in, 2 out]
      n132 = Multiply(x=w346, y=w347) -> (x*y=w348:dbl)
      n133 = property on="X Velocity SP mm/sec" class="DigNum (strict)"("Val(Sgnl)"=w348) -> ()  [unwired: 2 in, 2 out]
      "X offset mm" <- 0.0 ("offset")
      "X steps/rev" <- w350
      "X mm/rev" <- w347
    }
  }
  n134 = flat-sequence {
    tunnel: [w355] -> w8
    tunnel: [w354] -> w7
    tunnel: [w365] -> w28
    tunnel: [w363] -> w26
    tunnel: w8 -> [w366]
    tunnel: w7 -> [w364]
    tunnel: w28 -> [w370]
    tunnel: [w369] -> w27
    tunnel: w26 -> [w371]
    tunnel: [w373] -> w25
    tunnel: [w382] -> w70
    tunnel: [w384] -> w69
    tunnel: w27 -> [w383]
    tunnel: w25 -> [w385]
    tunnel: w70 -> [w392]
    tunnel: [w391] -> w68
    tunnel: w69 -> [w389]
    tunnel: [w390] -> w67
    tunnel: [w402] -> w66
    tunnel: [w403] -> w65
    tunnel: w68 -> [w401]
    tunnel: w67 -> [w400]
    tunnel: w66 -> [w413]
    tunnel: w65 -> [w412]
    tunnel: [w415] -> w57
    tunnel: [w414] -> w56
    tunnel: [w409] -> w55
    tunnel: [w420] -> w63
    tunnel: [w421] -> w64
    tunnel: w57 -> [w421]
    tunnel: w56 -> [w420]
    tunnel: w55 -> [w416]
    frame #0 {
      w362 = refnum<visa-resource-name> "COM4" ("COM PORT")
      w360 = u16 0 items=["None", "XON/XOFF", "RTS/CTS", "XON/XOFF & RTS/CTS", "DTR/DSR", "XON/XOFF & DTR/DSR"] ("flow control (0:none)")
      w359 = u16 10 items=["1.0"=10, "1.5"=15, "2.0"=20] ("stop bits (10: 1 bit)")
      # "Stop bits"
      n135 = call-poly "VISA Configure Serial Port"("VISA resource name"=w362, "timeout (10sec)"=u32 10000, "baud rate (9600)"=u32 9600, "data bits (8)"=u16 8, "parity (0:none)"=enum16{"None", "Odd", "Even", "Mark", "Space"}."None", "stop bits (10: 1 bit)"=w359, "flow control (0:none)"=w360) -> ("VISA resource name out"=w355:refnum<visa-resource-name>, "error out"=w354:errorcluster)  [unwired: 7 in]
      "X COM PORT" <- w362
    }
    frame #1 {
      n136 = call "mDrive Send Command.vi"("error in (no error)"=w364, "Extra"="EM=2", "Command"=T1."Send String", "VISA resource name"=w366) -> ("error out"=w363:errorcluster, "VISA resource name out"=w365:refnum<visa-resource-name>)  [unwired: 3 in, 1 out]
    }
    frame #2 {
      n137 = Number To Decimal String(number=1000000) -> (decimal integer string=w374:string)  [unwired: 1 in]
      n138 = call "mDrive Send Command.vi"("error in (no error)"=w371, "Extra"=w374, "Command"=T1."Accel Rate", "VISA resource name"=w370) -> ("error out"=w372:errorcluster, "VISA resource name out"=w378:refnum<visa-resource-name>)  [unwired: 3 in, 1 out]
      n139 = call "mDrive Send Command.vi"("error in (no error)"=w372, "Extra"=w374, "Command"=T1."Decel Rate", "VISA resource name"=w378) -> ("error out"=w373:errorcluster, "VISA resource name out"=w369:refnum<visa-resource-name>)  [unwired: 3 in, 1 out]
    }
    frame #3 {
      # "Run Current %"
      n140 = property on="X Run Current %" class="DigNum (strict)"() -> ("Value"=w380:i32)  [unwired: 2 in, 2 out]
      n141 = Number To Decimal String(number=w380) -> (decimal integer string=w381:string)  [unwired: 1 in]
      n142 = call "mDrive Send Command.vi"("error in (no error)"=w385, "Extra"=w381, "Command"=T1."Run Current", "VISA resource name"=w383) -> ("error out"=w384:errorcluster, "VISA resource name out"=w382:refnum<visa-resource-name>)  [unwired: 3 in, 1 out]
    }
    frame #4 {
      # "Holding Current %"
      n143 = property on="X Holding Current %" class="DigNum (strict)"() -> ("Value"=w387:i32)  [unwired: 2 in, 2 out]
      n144 = Number To Decimal String(number=w387) -> (decimal integer string=w388:string)  [unwired: 1 in]
      n145 = call "mDrive Send Command.vi"("error in (no error)"=w389, "Extra"=w388, "Command"=T1."Holding Current", "VISA resource name"=w392) -> ("error out"=w390:errorcluster, "VISA resource name out"=w391:refnum<visa-resource-name>)  [unwired: 3 in, 1 out]
    }
    frame #5 {
      # "Velocity Max"
      n146 = property on="X Velocity SP step/sec" class="DigNum (strict)"() -> ("Value"=w399:i32)  [unwired: 2 in, 2 out]
      n147 = Number To Decimal String(number=w399) -> (decimal integer string=w398:string)  [unwired: 1 in]
      n148 = call "mDrive Send Command.vi"("error in (no error)"=w400, "Extra"=w398, "Command"=T1."Max Velocity", "VISA resource name"=w401) -> ("error out"=w396:errorcluster, "VISA resource name out"=w406:refnum<visa-resource-name>)  [unwired: 3 in, 1 out]
      n149 = call "mDrive Send Command.vi"("error in (no error)"=w396, "Extra"="VM", "Command"=T1."Print Parameter", "VISA resource name"=w406) -> ("error out"=w403:errorcluster, "read buffer"=w404:string, "VISA resource name out"=w402:refnum<visa-resource-name>)  [unwired: 3 in]
      n150 = Decimal String To Number(string=w404, offset=0) -> (number=w397:i32)  [unwired: 1 in, 1 out]
      n151 = property on="X velocity PV step/sec" class="DigNum (strict)"("Val(Sgnl)"=w397) -> ()  [unwired: 2 in, 2 out]
    }
    frame #6 {
      # "PRINT POSITION"
      n152 = call "mDrive Send Command.vi"("error in (no error)"=w412, "Extra"="P", "Command"=T1."Print Parameter", "VISA resource name"=w413) -> ("error out"=w414:errorcluster, "read buffer"=w411:string, "VISA resource name out"=w415:refnum<visa-resource-name>)  [unwired: 3 in]
      n153 = Decimal String To Number(string=w411, offset=0) -> (number=w409:i32)  [unwired: 1 in, 1 out]
    }
    frame #7 {
      w418 = -2304000 ("lower limit")
      w419 = 2304000 ("upper limit")
      n154 = property on="X Step SP" class="DigNum (strict)"("Val(Sgnl)"=w416) -> ()  [unwired: 2 in, 2 out]
      n155 = property on="X Step SP" class="DigNum (strict)"("Maximum"=w419) -> ()  [unwired: 2 in, 2 out]
      n156 = In Range and Coerce(upper limit=w419, x=w416, lower limit=w418) -> (In Range?=w417:bool)  [unwired: 1 out]
      n157 = property on="X Step SP" class="DigNum (strict)"("Minimum"=w418) -> ()  [unwired: 2 in, 2 out]
      n158 = property on="X  in Range" class="Bool (strict)"("Val(Sgnl)"=w417) -> ()  [unwired: 2 in, 2 out]
      "X MINPOS" <- w418
      "X MAXPOS" <- w419
    }
  }
  n159 = property on="Z Step SP" class="DigNum (strict)"("Minimum"=0 ("lower limit")) -> ()  [unwired: 2 in, 2 out]
  n160 = property on="Z Step SP" class="DigNum (strict)"("Maximum"=102400000 ("upper limit")) -> ()  [unwired: 2 in, 2 out]
  n161 = property on="R Step SP" class="DigNum (strict)"("Minimum"=-6144000 ("lower limit")) -> ()  [unwired: 2 in, 2 out]
  n162 = property on="R Step SP" class="DigNum (strict)"("Maximum"=0 ("upper limit")) -> ()  [unwired: 2 in, 2 out]
  n163 = while {
    tunnel: w80 -> [w435]
    tunnel: w79 -> [w438]
    tunnel: [w439] -> w77
    tunnel: [w437] -> w78
    tunnel: w64 -> [w433]
    tunnel: w63 -> [w432]
    tunnel: [w431] -> w62
    tunnel: [w430] -> w61
    tunnel: w36 -> [w429]
    tunnel: w35 -> [w428]
    tunnel: [w427] -> w34
    tunnel: [w426] -> w33
    tunnel: w32 -> [w425]
    tunnel: w31 -> [w424]
    tunnel: [w423] -> w30
    tunnel: [w422] -> w29
    stop <- w434 stop-if-true
    n164 = event shown="[3] \"Y Scan Length SP steps\", \"Y Scan Velocity SP steps/sec \", \"X Scan Velocity SP steps/sec \", \"X Scan Length SP steps\", \"Z Scan Velocity SP steps/sec\", \"Z Scan Length SP steps\", \"R Scan Velocity SP steps/sec\", \"R Scan Length SP steps\": Value Change" {
      selector: _ -> [_ _ _ _ _ _ _ _ _ _ _ _ _ _ _ _ _ _ _ _ _ _ _ _ _]
      dyn-events: _ -> [_ _ _ _ _ _ _ _ _ _ _ _ _ _ _ _ _ _ _ _ _ _ _ _ _]
      timeout: 100 -> [_ _ _ _ _ _ _ _ _ _ _ _ _ _ _ _ _ _ _ _ _ _ _ _ _]
      tunnel: w438 -> [w517 _ _ _ _ _ _ _ _ _ _ _ w1358 _ _ _ _ w1607 _ _ w1703 w1719 w1763 w1840 w2084]
      tunnel: [w516 _ _ _ _ _ _ _ _ _ _ _ w1364 _ _ _ _ w1605 _ _ w1703 w1717 w1765 w1829 w2082] -> w439
      tunnel: w435 -> [w455 _ _ _ _ _ _ _ _ _ _ _ w1359 _ _ _ _ w1606 _ _ w1704 w1720 w1764 w1842 w2085]
      tunnel: [w515 _ _ _ _ _ _ _ _ _ _ _ w1365 _ _ _ _ w1602 _ _ w1704 w1718 w1766 w1830 w2083] -> w437
      tunnel: [_ _ _ _ _ _ _ _ _ _ _ _ _ _ _ _ _ _ _ _ TRUE _ _ _ _] -> w434
      tunnel: w433 -> [w454 _ _ _ _ _ _ _ _ _ _ _ _ _ _ w1516 w1571 _ _ _ _ w1714 w1756 w1846 w2081]
      tunnel: w432 -> [w492 _ _ _ _ _ _ _ _ _ _ _ _ _ _ w1515 w1570 _ _ _ _ w1713 w1755 w1844 w2080]
      tunnel: [w491 _ _ _ _ _ _ _ _ _ _ _ _ _ _ w1514 w1569 _ _ _ _ w1716 w1754 w1822 w2079] -> w431
      tunnel: [w490 _ _ _ _ _ _ _ _ _ _ _ _ _ _ w1513 w1568 _ _ _ _ w1715 w1753 w1820 w2078] -> w430
      tunnel: w429 -> [w464 _ _ _ _ _ _ _ _ _ _ _ _ w1410 _ _ _ _ w1637 _ _ w1712 w1750 w1838 w2077]
      tunnel: w428 -> [w467 _ _ _ _ _ _ _ _ _ _ _ _ w1409 _ _ _ _ w1636 _ _ w1711 w1749 w1836 w2076]
      tunnel: [w466 _ _ _ _ _ _ _ _ _ _ _ _ w1407 _ _ _ _ w1634 _ _ w1710 w1748 w1828 w2073] -> w427
      tunnel: [w465 _ _ _ _ _ _ _ _ _ _ _ _ w1408 _ _ _ _ w1635 _ _ w1709 w1747 w1827 w2072] -> w426
      tunnel: w425 -> [w463 _ _ _ _ _ _ _ _ _ _ _ _ _ w1463 _ _ _ _ w1671 _ w1708 w1744 w1833 w2075]
      tunnel: w424 -> [w462 _ _ _ _ _ _ _ _ _ _ _ _ _ w1462 _ _ _ _ w1670 _ w1707 w1743 w1831 w2074]
      tunnel: [w461 _ _ _ _ _ _ _ _ _ _ _ _ _ w1460 _ _ _ _ w1669 _ w1706 w1742 w1825 w2071] -> w423
      tunnel: [w460 _ _ _ _ _ _ _ _ _ _ _ _ _ w1461 _ _ _ _ w1668 _ w1705 w1741 w1824 w2070] -> w422
      event #0 {
        n165 = event-data() -> ()  [unwired: 1 in, 2 out]
        n166 = flat-sequence {
          tunnel: [w813] -> w503
          tunnel: [w790] -> w502
          tunnel: [w802] -> w501
          tunnel: [w781] -> w500
          tunnel: w454 -> [w780]
          tunnel: w492 -> [w779]
          tunnel: w503 -> [w819]
          tunnel: [w819] -> w499
          tunnel: w502 -> [w818]
          tunnel: [w818] -> w498
          tunnel: w501 -> [w817]
          tunnel: [w817] -> w497
          tunnel: w500 -> [w814]
          tunnel: [w814] -> w496
          tunnel: w499 -> [w826]
          tunnel: [w827] -> w495
          tunnel: w498 -> [w829]
          tunnel: [w828] -> w494
          tunnel: w497 -> [w825]
          tunnel: [w824] -> w493
          tunnel: w496 -> [w824]
          tunnel: w495 -> [w839]
          tunnel: w494 -> [w840]
          tunnel: w493 -> [w842]
          tunnel: [w838] -> w490
          tunnel: [w837] -> w491
          frame #0 {
            w785 = 0.05 ("Delay Time (s)")
            n167 = property on="X Step SP" class="DigNum (strict)"() -> ("Maximum"=w804:dbl)  [unwired: 2 in, 2 out]
            n168 = property on="X Step SP" class="DigNum (strict)"() -> ("Minimum"=w806:dbl)  [unwired: 2 in, 2 out]
            n169 = property on="X steps/rev" class="DigNum (strict)"() -> ("Value"=w800:u32)  [unwired: 2 in, 2 out]
            n170 = property on="X offset mm" class="DigNum (strict)"() -> ("Value"=w796:dbl)  [unwired: 2 in, 2 out]
            n171 = To Long Integer(number=w804) -> (32bit integer=w803:i32)
            n172 = To Long Integer(number=w806) -> (32bit integer=w805:i32)
            n173 = To Double Precision Float(number=w800) -> (double precision float=w801:dbl)
            n174 = call "mDrive Send Command.vi"("error in (no error)"=w779, "Extra"="P", "Command"=T1."Print Parameter", "VISA resource name"=w780) -> ("error out"=w808:errorcluster, "read buffer"=w812:string, "VISA resource name out"=w810:refnum<visa-resource-name>)  [unwired: 3 in]
            n175 = call "Time Delay12"("error in (no error)"=w808, "Delay Time (s)"=w785) -> ("error out"=w807:errorcluster)  [unwired: 9 in]
            n176 = Decimal String To Number(string=w812, offset=0) -> (number=w792:i32)  [unwired: 1 in, 1 out]
            n177 = To Long Integer(number=w792) -> (32bit integer=w794:i32)
            n178 = property on="X Step PV" class="DigNum (strict)"("Val(Sgnl)"=w794) -> ()  [unwired: 2 in, 2 out]
            n179 = call "mDrive Send Command.vi"("error in (no error)"=w807, "Extra"="MV", "Command"=T1."Print Parameter", "VISA resource name"=w810) -> ("error out"=w809:errorcluster, "read buffer"=w778:string, "VISA resource name out"=w813:refnum<visa-resource-name>)  [unwired: 3 in]
            n180 = call "Time Delay11"("error in (no error)"=w809, "Delay Time (s)"=w785) -> ("error out"=w790:errorcluster)  [unwired: 9 in]
            n181 = In Range and Coerce(upper limit=w803, x=w794, lower limit=w805) -> (In Range?=w802:bool)  [unwired: 1 out]
            n182 = To Double Precision Float(number=w794) -> (double precision float=w795:dbl)
            n183 = Decimal String To Number(string=w778, offset=0 ("offset (0)")) -> (number=w784:i32)  [unwired: 1 in, 1 out]
            n184 = Divide(x=w795, y=w801) -> (x/y=w799:dbl)
            n185 = Number To Boolean Array(number=w784) -> (Boolean array=w783:bool[])
            n186 = property on="X  in Range" class="Bool (strict)"("Val(Sgnl)"=w802) -> ()  [unwired: 2 in, 2 out]
            n187 = Not Equal?(x=w778, y="") -> (x != y?=w776:bool)
            n188 = property on="X mm/rev" class="DigNum (strict)"() -> ("Value"=w798:dbl)  [unwired: 2 in, 2 out]
            n189 = Index Array(array=w783, index=0) -> (element=w781:bool)
            n190 = property on="X Ready" class="Bool (strict)"("Val(Sgnl)"=w776) -> ()  [unwired: 2 in, 2 out]
            n191 = Multiply(x=w799, y=w798) -> (x*y=w797:dbl)
            n192 = property on="X  in Motion" class="Bool (strict)"("Val(Sgnl)"=w781) -> ()  [unwired: 2 in, 2 out]
            n193 = Add(x=w797, y=w796) -> (x+y=w793:dbl)
            n194 = property on="X Position mm PV" class="DigNum (strict)"("Val(Sgnl)"=w793) -> ()  [unwired: 2 in, 2 out]
          }
          frame #1 {
            n195 = property on="X Scan" class="Bool (strict)"() -> ("Value"=w815:bool)  [unwired: 2 in, 2 out]
            n196 = Or(x=w814, y=w815) -> (x .or. y?=w816:bool)
            n197 = case shown="True" w816 {
              frame #0 {
                n198 = property on="X Go" class="Bool"("DisabledEnum"=T2."Enabled" ("Disabled")) -> ()  [unwired: 2 in, 2 out]
                n199 = property on="X Scan OK" class="Bool"("DisabledEnum"=T2."Enabled" ("Disabled")) -> ()  [unwired: 2 in, 2 out]
              }
              frame #1 {
                n200 = property on="X Go" class="Bool"("DisabledEnum"=T2."Disabled and Grayed Out" ("Disabled")) -> ()  [unwired: 2 in, 2 out]
                n201 = property on="X Scan OK" class="Bool"("DisabledEnum"=T2."Disabled and Grayed Out" ("Disabled")) -> ()  [unwired: 2 in, 2 out]
              }
            }
          }
          frame #2 {
            n202 = case shown="False" w825 {
              tunnel: w826 -> [w832 w836]
              tunnel: [w833 w836] -> w827
              tunnel: [w834 w835] -> w828
              tunnel: w829 -> [w831 w835]
              frame #0 {
                n203 = call "mDrive Send Command.vi"("error in (no error)"=w831, "Command"=T1."Stop", "VISA resource name"=w832) -> ("error out"=w834:errorcluster, "VISA resource name out"=w833:refnum<visa-resource-name>)  [unwired: 4 in, 1 out]
              }
              frame #1 {
              }
            }
          }
          frame #3 {
            n204 = property on="X Backlash corr" class="Bool (strict)"() -> ("Value"=w843:bool)  [unwired: 2 in, 2 out]
            n205 = Implies(1:w842, 2:w843) -> (0:w841:bool)
            n206 = case shown="False" w841 {
              tunnel: w840 -> [w850 w903]
              tunnel: w839 -> [w849 w904]
              tunnel: [w848 w903] -> w838
              tunnel: [w847 w904] -> w837
              frame #0 {
                # "Backlash"
                n207 = flat-sequence {
                  tunnel: [w865] -> w862
                  tunnel: [w867] -> w861
                  tunnel: [w866] -> w860
                  tunnel: w850 -> [w864]
                  tunnel: w849 -> [w863]
                  tunnel: w862 -> [w875]
                  tunnel: [w875] -> w859
                  tunnel: w861 -> [w874]
                  tunnel: w860 -> [w873]
                  tunnel: [w872] -> w858
                  tunnel: [w871] -> w857
                  tunnel: [w870] -> w846
                  tunnel: w859 -> [w885]
                  tunnel: w858 -> [w884]
                  tunnel: w857 -> [w882]
                  tunnel: [w883] -> w856
                  tunnel: [w882] -> w855
                  tunnel: [w881] -> w852
                  tunnel: [w880] -> w851
                  tunnel: w846 -> [w880]
                  tunnel: w856 -> [w896]
                  tunnel: w855 -> [w889]
                  tunnel: [w896] -> w854
                  tunnel: [w895] -> w853
                  tunnel: w852 -> [w895]
                  tunnel: w851 -> [w891]
                  tunnel: [w890] -> w844
                  tunnel: w854 -> [w900]
                  tunnel: w853 -> [w899]
                  tunnel: [w898] -> w848
                  tunnel: [w897] -> w845
                  tunnel: w844 -> [w897]
                  tunnel: [w902] -> w847
                  tunnel: w845 -> [w902]
                  frame #0 {
                    n208 = property on="X Backlash steps/sec" class="DigNum (strict)"() -> ("Value"=w865:i32)  [unwired: 2 in, 2 out]
                    n209 = Number To Decimal String(number=w865) -> (decimal integer string=w868:string)  [unwired: 1 in]
                    n210 = call "mDrive Send Command.vi"("error in (no error)"=w864, "Extra"=w868, "Command"=T1."Max Velocity", "VISA resource name"=w863) -> ("error out"=w866:errorcluster, "VISA resource name out"=w867:refnum<visa-resource-name>)  [unwired: 3 in, 1 out]
                  }
                  frame #1 {
                    n211 = property on="X Backlash" class="DigNum (strict)"() -> ("Value"=w870:i32)  [unwired: 2 in, 2 out]
                    n212 = Number To Decimal String(number=w870) -> (decimal integer string=w876:string)  [unwired: 1 in]
                    n213 = call "mDrive Send Command.vi"("error in (no error)"=w873, "Extra"=w876, "Command"=T1."Move to Relative Position", "VISA resource name"=w874) -> ("error out"=w872:errorcluster, "VISA resource name out"=w871:refnum<visa-resource-name>)  [unwired: 3 in, 1 out]
                  }
                  frame #2 {
                    n214 = To Double Precision Float(number=w880) -> (double precision float=w878:dbl)
                    n215 = To Double Precision Float(number=w885) -> (double precision float=w887:dbl)
                    n216 = Absolute Value(x=w878) -> (abs(x)=w879:dbl)
                    n217 = Divide(x=w879, y=w887) -> (x/y=w888:dbl)
                    n218 = Add(x=w888, y=0.3) -> (x+y=w881:dbl)
                    n219 = call "Time Delay13"("error in (no error)"=w884, "Delay Time (s)"=w881) -> ("error out"=w883:errorcluster)  [unwired: 9 in]
                  }
                  frame #3 {
                    n220 = Negate(x=w891) -> (-x=w892:i32)
                    n221 = Number To Decimal String(number=w892) -> (decimal integer string=w893:string)  [unwired: 1 in]
                    n222 = call "mDrive Send Command.vi"("Extra"=w893, "Command"=T1."Move to Relative Position", "VISA resource name"=w889) -> ("VISA resource name out"=w890:refnum<visa-resource-name>)  [unwired: 4 in, 2 out]
                  }
                  frame #4 {
                    n223 = call "Time Delay14"("error in (no error)"=w900, "Delay Time (s)"=w899) -> ("error out"=w898:errorcluster)  [unwired: 9 in]
                  }
                  frame #5 {
                    n224 = property on="X Backlash corr" class="Bool (strict)"("Val(Sgnl)"=FALSE ("Value (Signaling)")) -> ()  [unwired: 2 in, 2 out]
                  }
                }
              }
              frame #1 {
              }
            }
          }
        }
        n225 = flat-sequence {
          tunnel: [w684] -> w489
          tunnel: [w661] -> w488
          tunnel: [w673] -> w487
          tunnel: [w652] -> w486
          tunnel: w464 -> [w651]
          tunnel: w467 -> [w650]
          tunnel: w489 -> [w690]
          tunnel: [w690] -> w485
          tunnel: w488 -> [w689]
          tunnel: [w689] -> w484
          tunnel: w487 -> [w688]
          tunnel: [w688] -> w483
          tunnel: w486 -> [w685]
          tunnel: [w685] -> w482
          tunnel: w485 -> [w697]
          tunnel: [w698] -> w481
          tunnel: w484 -> [w700]
          tunnel: [w699] -> w480
          tunnel: w483 -> [w696]
          tunnel: [w695] -> w479
          tunnel: w482 -> [w695]
          tunnel: w481 -> [w710]
          tunnel: w480 -> [w711]
          tunnel: w479 -> [w713]
          tunnel: [w709] -> w465
          tunnel: [w708] -> w466
          frame #0 {
            w656 = 0.05 ("Delay Time (s)")
            n226 = property on="Z Step SP" class="DigNum (strict)"() -> ("Maximum"=w675:dbl)  [unwired: 2 in, 2 out]
            n227 = property on="Z Step SP" class="DigNum (strict)"() -> ("Minimum"=w677:dbl)  [unwired: 2 in, 2 out]
            n228 = property on="Z steps/rev" class="DigNum (strict)"() -> ("Value"=w671:u32)  [unwired: 2 in, 2 out]
            n229 = property on="Z offset mm" class="DigNum (strict)"() -> ("Value"=w667:dbl)  [unwired: 2 in, 2 out]
            n230 = To Long Integer(number=w675) -> (32bit integer=w674:i32)
            n231 = To Long Integer(number=w677) -> (32bit integer=w676:i32)
            n232 = To Double Precision Float(number=w671) -> (double precision float=w672:dbl)
            n233 = call "mDrive Send Command.vi"("error in (no error)"=w650, "Extra"="P", "Command"=T1."Print Parameter", "VISA resource name"=w651) -> ("error out"=w679:errorcluster, "read buffer"=w683:string, "VISA resource name out"=w681:refnum<visa-resource-name>)  [unwired: 3 in]
            n234 = call "Time Delay17"("error in (no error)"=w679, "Delay Time (s)"=w656) -> ("error out"=w678:errorcluster)  [unwired: 9 in]
            n235 = Decimal String To Number(string=w683, offset=0) -> (number=w663:i32)  [unwired: 1 in, 1 out]
            n236 = To Long Integer(number=w663) -> (32bit integer=w665:i32)
            n237 = property on="Z Step PV" class="DigNum (strict)"("Val(Sgnl)"=w665) -> ()  [unwired: 2 in, 2 out]
            n238 = call "mDrive Send Command.vi"("error in (no error)"=w678, "Extra"="MV", "Command"=T1."Print Parameter", "VISA resource name"=w681) -> ("error out"=w680:errorcluster, "read buffer"=w647:string, "VISA resource name out"=w684:refnum<visa-resource-name>)  [unwired: 3 in]
            n239 = call "Time Delay16"("error in (no error)"=w680, "Delay Time (s)"=w656) -> ("error out"=w661:errorcluster)  [unwired: 9 in]
            n240 = In Range and Coerce(upper limit=w674, x=w665, lower limit=w676) -> (In Range?=w673:bool)  [unwired: 1 out]
            n241 = To Double Precision Float(number=w665) -> (double precision float=w666:dbl)
            n242 = Decimal String To Number(string=w647, offset=0 ("offset (0)")) -> (number=w655:i32)  [unwired: 1 in, 1 out]
            n243 = property on="Z in Range" class="Bool (strict)"("Val(Sgnl)"=w673) -> ()  [unwired: 2 in, 2 out]
            n244 = Divide(x=w666, y=w672) -> (x/y=w670:dbl)
            n245 = Number To Boolean Array(number=w655) -> (Boolean array=w654:bool[])
            n246 = Not Equal?(x=w647, y="") -> (x != y?=w648:bool)
            n247 = property on="Z Ready" class="Bool (strict)"("Val(Sgnl)"=w648) -> ()  [unwired: 2 in, 2 out]
            n248 = property on="Z mm/rev" class="DigNum (strict)"() -> ("Value"=w669:dbl)  [unwired: 2 in, 2 out]
            n249 = Index Array(array=w654, index=0) -> (element=w652:bool)
            n250 = Multiply(x=w670, y=w669) -> (x*y=w668:dbl)
            n251 = property on="Z in Motion" class="Bool (strict)"("Val(Sgnl)"=w652) -> ()  [unwired: 2 in, 2 out]
            n252 = Add(x=w668, y=w667) -> (x+y=w664:dbl)
            n253 = property on="Z Position mm PV" class="DigNum (strict)"("Val(Sgnl)"=w664) -> ()  [unwired: 2 in, 2 out]
          }
          frame #1 {
            n254 = property on="Z Scan" class="Bool (strict)"() -> ("Value"=w686:bool)  [unwired: 2 in, 2 out]
            n255 = Or(x=w685, y=w686) -> (x .or. y?=w687:bool)
            n256 = case shown="True" w687 {
              frame #0 {
                n257 = property on="Z Go" class="Bool"("DisabledEnum"=T2."Enabled" ("Disabled")) -> ()  [unwired: 2 in, 2 out]
                n258 = property on="Z Scan OK" class="Bool"("DisabledEnum"=T2."Enabled" ("Disabled")) -> ()  [unwired: 2 in, 2 out]
              }
              frame #1 {
                n259 = property on="Z Go" class="Bool"("DisabledEnum"=T2."Disabled and Grayed Out" ("Disabled")) -> ()  [unwired: 2 in, 2 out]
                n260 = property on="Z Scan OK" class="Bool"("DisabledEnum"=T2."Disabled and Grayed Out" ("Disabled")) -> ()  [unwired: 2 in, 2 out]
              }
            }
          }
          frame #2 {
            n261 = case shown="False" w696 {
              tunnel: w697 -> [w703 w707]
              tunnel: [w704 w707] -> w698
              tunnel: [w705 w706] -> w699
              tunnel: w700 -> [w702 w706]
              frame #0 {
                n262 = call "mDrive Send Command.vi"("error in (no error)"=w702, "Command"=T1."Stop", "VISA resource name"=w703) -> ("error out"=w705:errorcluster, "VISA resource name out"=w704:refnum<visa-resource-name>)  [unwired: 4 in, 1 out]
              }
              frame #1 {
              }
            }
          }
          frame #3 {
            n263 = property on="Z Backlash corr" class="Bool (strict)"() -> ("Value"=w714:bool)  [unwired: 2 in, 2 out]
            n264 = Implies(1:w713, 2:w714) -> (0:w712:bool)
            n265 = case shown="False" w712 {
              tunnel: w711 -> [w721 w774]
              tunnel: w710 -> [w720 w775]
              tunnel: [w719 w774] -> w709
              tunnel: [w718 w775] -> w708
              frame #0 {
                # "Backlash"
                n266 = flat-sequence {
                  tunnel: [w736] -> w733
                  tunnel: [w738] -> w732
                  tunnel: [w737] -> w731
                  tunnel: w721 -> [w735]
                  tunnel: w720 -> [w734]
                  tunnel: w733 -> [w746]
                  tunnel: [w746] -> w730
                  tunnel: w732 -> [w745]
                  tunnel: w731 -> [w744]
                  tunnel: [w743] -> w729
                  tunnel: [w742] -> w728
                  tunnel: [w741] -> w717
                  tunnel: w730 -> [w756]
                  tunnel: w729 -> [w755]
                  tunnel: w728 -> [w753]
                  tunnel: [w754] -> w727
                  tunnel: [w753] -> w726
                  tunnel: [w752] -> w723
                  tunnel: [w751] -> w722
                  tunnel: w717 -> [w751]
                  tunnel: w727 -> [w767]
                  tunnel: w726 -> [w760]
                  tunnel: [w767] -> w725
                  tunnel: [w766] -> w724
                  tunnel: w723 -> [w766]
                  tunnel: w722 -> [w762]
                  tunnel: [w761] -> w715
                  tunnel: w725 -> [w771]
                  tunnel: w724 -> [w770]
                  tunnel: [w769] -> w719
                  tunnel: [w768] -> w716
                  tunnel: w715 -> [w768]
                  tunnel: [w773] -> w718
                  tunnel: w716 -> [w773]
                  frame #0 {
                    n267 = property on="Z Backlash steps/sec" class="DigNum (strict)"() -> ("Value"=w736:i32)  [unwired: 2 in, 2 out]
                    n268 = Number To Decimal String(number=w736) -> (decimal integer string=w739:string)  [unwired: 1 in]
                    n269 = call "mDrive Send Command.vi"("error in (no error)"=w735, "Extra"=w739, "Command"=T1."Max Velocity", "VISA resource name"=w734) -> ("error out"=w737:errorcluster, "VISA resource name out"=w738:refnum<visa-resource-name>)  [unwired: 3 in, 1 out]
                  }
                  frame #1 {
                    n270 = property on="Z Backlash" class="DigNum (strict)"() -> ("Value"=w741:i32)  [unwired: 2 in, 2 out]
                    n271 = Number To Decimal String(number=w741) -> (decimal integer string=w747:string)  [unwired: 1 in]
                    n272 = call "mDrive Send Command.vi"("error in (no error)"=w744, "Extra"=w747, "Command"=T1."Move to Relative Position", "VISA resource name"=w745) -> ("error out"=w743:errorcluster, "VISA resource name out"=w742:refnum<visa-resource-name>)  [unwired: 3 in, 1 out]
                  }
                  frame #2 {
                    n273 = To Double Precision Float(number=w751) -> (double precision float=w749:dbl)
                    n274 = To Double Precision Float(number=w756) -> (double precision float=w758:dbl)
                    n275 = Absolute Value(x=w749) -> (abs(x)=w750:dbl)
                    n276 = Divide(x=w750, y=w758) -> (x/y=w759:dbl)
                    n277 = Add(x=w759, y=0.5) -> (x+y=w752:dbl)
                    n278 = call "Time Delay18"("error in (no error)"=w755, "Delay Time (s)"=w752) -> ("error out"=w754:errorcluster)  [unwired: 9 in]
                  }
                  frame #3 {
                    n279 = Negate(x=w762) -> (-x=w763:i32)
                    n280 = Number To Decimal String(number=w763) -> (decimal integer string=w764:string)  [unwired: 1 in]
                    n281 = call "mDrive Send Command.vi"("Extra"=w764, "Command"=T1."Move to Relative Position", "VISA resource name"=w760) -> ("VISA resource name out"=w761:refnum<visa-resource-name>)  [unwired: 4 in, 2 out]
                  }
                  frame #4 {
                    n282 = call "Time Delay19"("error in (no error)"=w771, "Delay Time (s)"=w770) -> ("error out"=w769:errorcluster)  [unwired: 9 in]
                  }
                  frame #5 {
                    n283 = property on="Z Backlash corr" class="Bool (strict)"("Val(Sgnl)"=FALSE ("Value (Signaling)")) -> ()  [unwired: 2 in, 2 out]
                  }
                }
              }
              frame #1 {
              }
            }
          }
        }
        n284 = flat-sequence {
          tunnel: w517 -> [w937]
          tunnel: w455 -> [w936]
          tunnel: [w942] -> w514
          tunnel: [w917] -> w512
          tunnel: [w929] -> w510
          tunnel: [w908] -> w508
          tunnel: w514 -> [w948]
          tunnel: [w948] -> w513
          tunnel: w512 -> [w947]
          tunnel: [w947] -> w511
          tunnel: w510 -> [w946]
          tunnel: [w946] -> w509
          tunnel: w508 -> [w943]
          tunnel: [w943] -> w504
          tunnel: w513 -> [w955]
          tunnel: [w956] -> w507
          tunnel: w511 -> [w958]
          tunnel: [w957] -> w506
          tunnel: w509 -> [w954]
          tunnel: [w953] -> w505
          tunnel: w504 -> [w953]
          tunnel: w507 -> [w968]
          tunnel: w506 -> [w969]
          tunnel: w505 -> [w971]
          tunnel: [w967] -> w516
          tunnel: [w966] -> w515
          frame #0 {
            w912 = 0.05 ("Delay Time (s)")
            n285 = property on="Y Step SP" class="DigNum (strict)"() -> ("Maximum"=w931:dbl)  [unwired: 2 in, 2 out]
            n286 = property on="Y Step SP" class="DigNum (strict)"() -> ("Minimum"=w933:dbl)  [unwired: 2 in, 2 out]
            n287 = property on="Y steps/rev" class="DigNum (strict)"() -> ("Value"=w927:u32)  [unwired: 2 in, 2 out]
            n288 = property on="Y offset mm" class="DigNum (strict)"() -> ("Value"=w923:dbl)  [unwired: 2 in, 2 out]
            n289 = To Long Integer(number=w931) -> (32bit integer=w930:i32)
            n290 = To Long Integer(number=w933) -> (32bit integer=w932:i32)
            n291 = To Double Precision Float(number=w927) -> (double precision float=w928:dbl)
            n292 = call "mDrive Send Command.vi"("error in (no error)"=w937, "Extra"="P", "Command"=T1."Print Parameter", "VISA resource name"=w936) -> ("error out"=w935:errorcluster, "read buffer"=w941:string, "VISA resource name out"=w939:refnum<visa-resource-name>)  [unwired: 3 in]
            n293 = call "Time Delay4"("error in (no error)"=w935, "Delay Time (s)"=w912) -> ("error out"=w934:errorcluster)  [unwired: 9 in]
            n294 = Decimal String To Number(string=w941, offset=0) -> (number=w919:i32)  [unwired: 1 in, 1 out]
            n295 = To Long Integer(number=w919) -> (32bit integer=w921:i32)
            n296 = property on="Y Step PV" class="DigNum (strict)"("Val(Sgnl)"=w921) -> ()  [unwired: 2 in, 2 out]
            n297 = call "mDrive Send Command.vi"("error in (no error)"=w934, "Extra"="MV", "Command"=T1."Print Parameter", "VISA resource name"=w939) -> ("error out"=w938:errorcluster, "read buffer"=w905:string, "VISA resource name out"=w942:refnum<visa-resource-name>)  [unwired: 3 in]
            n298 = call "Time Delay3"("error in (no error)"=w938, "Delay Time (s)"=w912) -> ("error out"=w917:errorcluster)  [unwired: 9 in]
            n299 = In Range and Coerce(upper limit=w930, x=w921, lower limit=w932) -> (In Range?=w929:bool)  [unwired: 1 out]
            n300 = To Double Precision Float(number=w921) -> (double precision float=w922:dbl)
            n301 = Decimal String To Number(string=w905, offset=0 ("offset (0)")) -> (number=w911:i32)  [unwired: 1 in, 1 out]
            n302 = property on="Y in Range" class="Bool (strict)"("Val(Sgnl)"=w929) -> ()  [unwired: 2 in, 2 out]
            n303 = Divide(x=w922, y=w928) -> (x/y=w926:dbl)
            n304 = Number To Boolean Array(number=w911) -> (Boolean array=w910:bool[])
            n305 = Not Equal?(x=w905, y="") -> (x != y?=w906:bool)
            n306 = property on="Y Ready" class="Bool (strict)"("Val(Sgnl)"=w906) -> ()  [unwired: 2 in, 2 out]
            n307 = property on="Y mm/rev" class="DigNum (strict)"() -> ("Value"=w925:dbl)  [unwired: 2 in, 2 out]
            n308 = Index Array(array=w910, index=0) -> (element=w908:bool)
            n309 = Multiply(x=w926, y=w925) -> (x*y=w924:dbl)
            n310 = property on="Y in Motion" class="Bool (strict)"("Val(Sgnl)"=w908) -> ()  [unwired: 2 in, 2 out]
            n311 = Add(x=w924, y=w923) -> (x+y=w920:dbl)
            n312 = property on="Y Position mm PV" class="DigNum (strict)"("Val(Sgnl)"=w920) -> ()  [unwired: 2 in, 2 out]
          }
          frame #1 {
            n313 = property on="Y Scan" class="Bool (strict)"() -> ("Value"=w944:bool)  [unwired: 2 in, 2 out]
            n314 = Or(x=w943, y=w944) -> (x .or. y?=w945:bool)
            n315 = case shown="True" w945 {
              frame #0 {
                n316 = property on="Y Go" class="Bool"("DisabledEnum"=T2."Enabled" ("Disabled")) -> ()  [unwired: 2 in, 2 out]
                n317 = property on="Y Scan OK" class="Bool"("DisabledEnum"=T2."Enabled" ("Disabled")) -> ()  [unwired: 2 in, 2 out]
              }
              frame #1 {
                n318 = property on="Y Go" class="Bool"("DisabledEnum"=T2."Disabled and Grayed Out" ("Disabled")) -> ()  [unwired: 2 in, 2 out]
                n319 = property on="Y Scan OK" class="Bool"("DisabledEnum"=T2."Disabled and Grayed Out" ("Disabled")) -> ()  [unwired: 2 in, 2 out]
              }
            }
          }
          frame #2 {
            n320 = case shown="False" w954 {
              tunnel: w955 -> [w961 w965]
              tunnel: [w962 w965] -> w956
              tunnel: [w963 w964] -> w957
              tunnel: w958 -> [w960 w964]
              frame #0 {
                n321 = call "mDrive Send Command.vi"("error in (no error)"=w960, "Command"=T1."Stop", "VISA resource name"=w961) -> ("error out"=w963:errorcluster, "VISA resource name out"=w962:refnum<visa-resource-name>)  [unwired: 4 in, 1 out]
              }
              frame #1 {
              }
            }
          }
          frame #3 {
            n322 = property on="Y Backlash corr" class="Bool (strict)"() -> ("Value"=w972:bool)  [unwired: 2 in, 2 out]
            n323 = Implies(1:w971, 2:w972) -> (0:w970:bool)
            n324 = case shown="False" w970 {
              tunnel: w969 -> [w979 w1032]
              tunnel: w968 -> [w978 w1033]
              tunnel: [w977 w1032] -> w967
              tunnel: [w976 w1033] -> w966
              frame #0 {
                # "Backlash"
                n325 = flat-sequence {
                  tunnel: [w994] -> w991
                  tunnel: [w996] -> w990
                  tunnel: [w995] -> w989
                  tunnel: w979 -> [w993]
                  tunnel: w978 -> [w992]
                  tunnel: w991 -> [w1004]
                  tunnel: [w1004] -> w988
                  tunnel: w990 -> [w1003]
                  tunnel: w989 -> [w1002]
                  tunnel: [w1001] -> w987
                  tunnel: [w1000] -> w986
                  tunnel: [w999] -> w975
                  tunnel: w988 -> [w1014]
                  tunnel: w987 -> [w1013]
                  tunnel: w986 -> [w1011]
                  tunnel: [w1012] -> w985
                  tunnel: [w1011] -> w984
                  tunnel: [w1010] -> w981
                  tunnel: [w1009] -> w980
                  tunnel: w975 -> [w1009]
                  tunnel: w985 -> [w1025]
                  tunnel: w984 -> [w1018]
                  tunnel: [w1025] -> w983
                  tunnel: [w1024] -> w982
                  tunnel: w981 -> [w1024]
                  tunnel: w980 -> [w1020]
                  tunnel: [w1019] -> w973
                  tunnel: w983 -> [w1029]
                  tunnel: w982 -> [w1028]
                  tunnel: [w1027] -> w977
                  tunnel: [w1026] -> w974
                  tunnel: w973 -> [w1026]
                  tunnel: [w1031] -> w976
                  tunnel: w974 -> [w1031]
                  frame #0 {
                    n326 = property on="Y Backlash steps/sec" class="DigNum (strict)"() -> ("Value"=w994:i32)  [unwired: 2 in, 2 out]
                    n327 = Number To Decimal String(number=w994) -> (decimal integer string=w997:string)  [unwired: 1 in]
                    n328 = call "mDrive Send Command.vi"("error in (no error)"=w993, "Extra"=w997, "Command"=T1."Max Velocity", "VISA resource name"=w992) -> ("error out"=w995:errorcluster, "VISA resource name out"=w996:refnum<visa-resource-name>)  [unwired: 3 in, 1 out]
                  }
                  frame #1 {
                    n329 = property on="Y Backlash" class="DigNum (strict)"() -> ("Value"=w999:i32)  [unwired: 2 in, 2 out]
                    n330 = Number To Decimal String(number=w999) -> (decimal integer string=w1005:string)  [unwired: 1 in]
                    n331 = call "mDrive Send Command.vi"("error in (no error)"=w1002, "Extra"=w1005, "Command"=T1."Move to Relative Position", "VISA resource name"=w1003) -> ("error out"=w1001:errorcluster, "VISA resource name out"=w1000:refnum<visa-resource-name>)  [unwired: 3 in, 1 out]
                  }
                  frame #2 {
                    n332 = To Double Precision Float(number=w1009) -> (double precision float=w1007:dbl)
                    n333 = To Double Precision Float(number=w1014) -> (double precision float=w1016:dbl)
                    n334 = Absolute Value(x=w1007) -> (abs(x)=w1008:dbl)
                    n335 = Divide(x=w1008, y=w1016) -> (x/y=w1017:dbl)
                    n336 = Add(x=w1017, y=0.3) -> (x+y=w1010:dbl)
                    n337 = call "Time Delay8"("error in (no error)"=w1013, "Delay Time (s)"=w1010) -> ("error out"=w1012:errorcluster)  [unwired: 9 in]
                  }
                  frame #3 {
                    n338 = Negate(x=w1020) -> (-x=w1021:i32)
                    n339 = Number To Decimal String(number=w1021) -> (decimal integer string=w1022:string)  [unwired: 1 in]
                    n340 = call "mDrive Send Command.vi"("Extra"=w1022, "Command"=T1."Move to Relative Position", "VISA resource name"=w1018) -> ("VISA resource name out"=w1019:refnum<visa-resource-name>)  [unwired: 4 in, 2 out]
                  }
                  frame #4 {
                    n341 = call "Time Delay2"("error in (no error)"=w1029, "Delay Time (s)"=w1028) -> ("error out"=w1027:errorcluster)  [unwired: 9 in]
                  }
                  frame #5 {
                    n342 = property on="Y Backlash corr" class="Bool (strict)"("Val(Sgnl)"=FALSE ("Value (Signaling)")) -> ()  [unwired: 2 in, 2 out]
                  }
                }
              }
              frame #1 {
              }
            }
          }
        }
        n343 = flat-sequence {
          tunnel: [w555] -> w478
          tunnel: [w532] -> w477
          tunnel: [w544] -> w476
          tunnel: [w523] -> w475
          tunnel: w463 -> [w522]
          tunnel: w462 -> [w521]
          tunnel: w478 -> [w561]
          tunnel: [w561] -> w474
          tunnel: w477 -> [w560]
          tunnel: [w560] -> w473
          tunnel: w476 -> [w559]
          tunnel: [w559] -> w472
          tunnel: w475 -> [w556]
          tunnel: [w556] -> w471
          tunnel: w474 -> [w568]
          tunnel: [w569] -> w470
          tunnel: w473 -> [w571]
          tunnel: [w570] -> w469
          tunnel: w472 -> [w567]
          tunnel: [w566] -> w468
          tunnel: w471 -> [w566]
          tunnel: w470 -> [w581]
          tunnel: w469 -> [w582]
          tunnel: w468 -> [w584]
          tunnel: [w580] -> w460
          tunnel: [w579] -> w461
          frame #0 {
            w527 = 0.05 ("Delay Time (s)")
            n344 = property on="R Step SP" class="DigNum (strict)"() -> ("Maximum"=w546:dbl)  [unwired: 2 in, 2 out]
            n345 = property on="R Step SP" class="DigNum (strict)"() -> ("Minimum"=w548:dbl)  [unwired: 2 in, 2 out]
            n346 = property on="R steps/rev" class="DigNum (strict)"() -> ("Value"=w542:u32)  [unwired: 2 in, 2 out]
            n347 = property on="R offset deg" class="DigNum (strict)"() -> ("Value"=w538:dbl)  [unwired: 2 in, 2 out]
            n348 = To Long Integer(number=w546) -> (32bit integer=w545:i32)
            n349 = To Long Integer(number=w548) -> (32bit integer=w547:i32)
            n350 = To Double Precision Float(number=w542) -> (double precision float=w543:dbl)
            n351 = call "mDrive Send Command.vi"("error in (no error)"=w521, "Extra"="P", "Command"=T1."Print Parameter", "VISA resource name"=w522) -> ("error out"=w550:errorcluster, "read buffer"=w554:string, "VISA resource name out"=w552:refnum<visa-resource-name>)  [unwired: 3 in]
            n352 = call "Time Delay21"("error in (no error)"=w550, "Delay Time (s)"=w527) -> ("error out"=w549:errorcluster)  [unwired: 9 in]
            n353 = Decimal String To Number(string=w554, offset=0) -> (number=w534:i32)  [unwired: 1 in, 1 out]
            n354 = To Long Integer(number=w534) -> (32bit integer=w536:i32)
            n355 = property on="R Step PV" class="DigNum (strict)"("Val(Sgnl)"=w536) -> ()  [unwired: 2 in, 2 out]
            n356 = call "mDrive Send Command.vi"("error in (no error)"=w549, "Extra"="MV", "Command"=T1."Print Parameter", "VISA resource name"=w552) -> ("error out"=w551:errorcluster, "read buffer"=w518:string, "VISA resource name out"=w555:refnum<visa-resource-name>)  [unwired: 3 in]
            n357 = call "Time Delay20"("error in (no error)"=w551, "Delay Time (s)"=w527) -> ("error out"=w532:errorcluster)  [unwired: 9 in]
            n358 = In Range and Coerce(upper limit=w545, x=w536, lower limit=w547) -> (In Range?=w544:bool)  [unwired: 1 out]
            n359 = To Double Precision Float(number=w536) -> (double precision float=w537:dbl)
            n360 = Decimal String To Number(string=w518, offset=0 ("offset (0)")) -> (number=w526:i32)  [unwired: 1 in, 1 out]
            n361 = property on="R in Range" class="Bool (strict)"("Val(Sgnl)"=w544) -> ()  [unwired: 2 in, 2 out]
            n362 = Divide(x=w537, y=w543) -> (x/y=w541:dbl)
            n363 = Number To Boolean Array(number=w526) -> (Boolean array=w525:bool[])
            n364 = Not Equal?(x=w518, y="") -> (x != y?=w519:bool)
            n365 = property on="R Ready" class="Bool (strict)"("Val(Sgnl)"=w519) -> ()  [unwired: 2 in, 2 out]
            n366 = property on="R deg/rev" class="DigNum (strict)"() -> ("Value"=w540:dbl)  [unwired: 2 in, 2 out]
            n367 = Index Array(array=w525, index=0) -> (element=w523:bool)
            n368 = Multiply(x=w541, y=w540) -> (x*y=w539:dbl)
            n369 = property on="R in Motion" class="Bool (strict)"("Val(Sgnl)"=w523) -> ()  [unwired: 2 in, 2 out]
            n370 = Add(x=w539, y=w538) -> (x+y=w535:dbl)
            n371 = property on="R Position deg PV" class="DigNum (strict)"("Val(Sgnl)"=w535) -> ()  [unwired: 2 in, 2 out]
          }
          frame #1 {
            n372 = property on="R Scan" class="Bool (strict)"() -> ("Value"=w557:bool)  [unwired: 2 in, 2 out]
            n373 = Or(x=w556, y=w557) -> (x .or. y?=w558:bool)
            n374 = case shown="True" w558 {
              frame #0 {
                n375 = property on="R Go" class="Bool"("DisabledEnum"=T2."Enabled" ("Disabled")) -> ()  [unwired: 2 in, 2 out]
                n376 = property on="R Scan OK" class="Bool"("DisabledEnum"=T2."Enabled" ("Disabled")) -> ()  [unwired: 2 in, 2 out]
              }
              frame #1 {
                n377 = property on="R Go" class="Bool"("DisabledEnum"=T2."Disabled and Grayed Out" ("Disabled")) -> ()  [unwired: 2 in, 2 out]
                n378 = property on="R Scan OK" class="Bool"("DisabledEnum"=T2."Disabled and Grayed Out" ("Disabled")) -> ()  [unwired: 2 in, 2 out]
              }
            }
          }
          frame #2 {
            n379 = case shown="False" w567 {
              tunnel: w568 -> [w574 w578]
              tunnel: [w575 w578] -> w569
              tunnel: [w576 w577] -> w570
              tunnel: w571 -> [w573 w577]
              frame #0 {
                n380 = call "mDrive Send Command.vi"("error in (no error)"=w573, "Command"=T1."Stop", "VISA resource name"=w574) -> ("error out"=w576:errorcluster, "VISA resource name out"=w575:refnum<visa-resource-name>)  [unwired: 4 in, 1 out]
              }
              frame #1 {
              }
            }
          }
          frame #3 {
            n381 = property on="R Backlash corr" class="Bool (strict)"() -> ("Value"=w585:bool)  [unwired: 2 in, 2 out]
            n382 = Implies(1:w584, 2:w585) -> (0:w583:bool)
            n383 = case shown="False" w583 {
              tunnel: w582 -> [w592 w645]
              tunnel: w581 -> [w591 w646]
              tunnel: [w590 w645] -> w580
              tunnel: [w589 w646] -> w579
              frame #0 {
                # "Backlash"
                n384 = flat-sequence {
                  tunnel: [w607] -> w604
                  tunnel: [w609] -> w603
                  tunnel: [w608] -> w602
                  tunnel: w592 -> [w606]
                  tunnel: w591 -> [w605]
                  tunnel: w604 -> [w617]
                  tunnel: [w617] -> w601
                  tunnel: w603 -> [w616]
                  tunnel: w602 -> [w615]
                  tunnel: [w614] -> w600
                  tunnel: [w613] -> w599
                  tunnel: [w612] -> w588
                  tunnel: w601 -> [w627]
                  tunnel: w600 -> [w626]
                  tunnel: w599 -> [w624]
                  tunnel: [w625] -> w598
                  tunnel: [w624] -> w597
                  tunnel: [w623] -> w594
                  tunnel: [w622] -> w593
                  tunnel: w588 -> [w622]
                  tunnel: w598 -> [w638]
                  tunnel: w597 -> [w631]
                  tunnel: [w638] -> w596
                  tunnel: [w637] -> w595
                  tunnel: w594 -> [w637]
                  tunnel: w593 -> [w633]
                  tunnel: [w632] -> w586
                  tunnel: w596 -> [w642]
                  tunnel: w595 -> [w641]
                  tunnel: [w640] -> w590
                  tunnel: [w639] -> w587
                  tunnel: w586 -> [w639]
                  tunnel: [w644] -> w589
                  tunnel: w587 -> [w644]
                  frame #0 {
                    n385 = property on="R Backlash steps/sec" class="DigNum (strict)"() -> ("Value"=w607:i32)  [unwired: 2 in, 2 out]
                    n386 = Number To Decimal String(number=w607) -> (decimal integer string=w610:string)  [unwired: 1 in]
                    n387 = call "mDrive Send Command.vi"("error in (no error)"=w606, "Extra"=w610, "Command"=T1."Max Velocity", "VISA resource name"=w605) -> ("error out"=w608:errorcluster, "VISA resource name out"=w609:refnum<visa-resource-name>)  [unwired: 3 in, 1 out]
                  }
                  frame #1 {
                    n388 = property on="R Backlash" class="DigNum (strict)"() -> ("Value"=w612:i32)  [unwired: 2 in, 2 out]
                    n389 = Number To Decimal String(number=w612) -> (decimal integer string=w618:string)  [unwired: 1 in]
                    n390 = call "mDrive Send Command.vi"("error in (no error)"=w615, "Extra"=w618, "Command"=T1."Move to Relative Position", "VISA resource name"=w616) -> ("error out"=w614:errorcluster, "VISA resource name out"=w613:refnum<visa-resource-name>)  [unwired: 3 in, 1 out]
                  }
                  frame #2 {
                    n391 = To Double Precision Float(number=w622) -> (double precision float=w620:dbl)
                    n392 = To Double Precision Float(number=w627) -> (double precision float=w629:dbl)
                    n393 = Absolute Value(x=w620) -> (abs(x)=w621:dbl)
                    n394 = Divide(x=w621, y=w629) -> (x/y=w630:dbl)
                    n395 = Add(x=w630, y=0.3) -> (x+y=w623:dbl)
                    n396 = call "Time Delay22"("error in (no error)"=w626, "Delay Time (s)"=w623) -> ("error out"=w625:errorcluster)  [unwired: 9 in]
                  }
                  frame #3 {
                    n397 = Negate(x=w633) -> (-x=w634:i32)
                    n398 = Number To Decimal String(number=w634) -> (decimal integer string=w635:string)  [unwired: 1 in]
                    n399 = call "mDrive Send Command.vi"("Extra"=w635, "Command"=T1."Move to Relative Position", "VISA resource name"=w631) -> ("VISA resource name out"=w632:refnum<visa-resource-name>)  [unwired: 4 in, 2 out]
                  }
                  frame #4 {
                    n400 = call "Time Delay23"("error in (no error)"=w642, "Delay Time (s)"=w641) -> ("error out"=w640:errorcluster)  [unwired: 9 in]
                  }
                  frame #5 {
                    n401 = property on="R Backlash corr" class="Bool (strict)"("Val(Sgnl)"=FALSE ("Value (Signaling)")) -> ()  [unwired: 2 in, 2 out]
                  }
                }
              }
              frame #1 {
              }
            }
          }
        }
        n402 = property on="X Position mm PV" class="DigNum (strict)"() -> ("Value"=w456:dbl)  [unwired: 2 in, 2 out]
        n403 = property on="Y Position mm PV" class="DigNum (strict)"() -> ("Value"=w449:dbl)  [unwired: 2 in, 2 out]
        n404 = property on="Z Position mm PV" class="DigNum (strict)"() -> ("Value"=w450:dbl)  [unwired: 2 in, 2 out]
        n405 = property on="R Position deg PV" class="DigNum (strict)"() -> ("Value"=w457:dbl)  [unwired: 2 in, 2 out]
        n406 = call "Build XY Graph"("Reset"=TRUE, "Y Input"=w449, "X Input"=w456) -> ("XY Graph"=→"XY Graph":cluster{"Y":dbl[], "Y":dbl[]}[])  [unwired: 7 in, 1 out]
        n407 = call "Build XY Graph2"("Reset"=TRUE, "Y Input"=w457, "X Input"=w450) -> ("XY Graph"=→"ZR Graph":cluster{"Y":dbl[], "Y":dbl[]}[])  [unwired: 7 in, 1 out]
        n408 = property on="Clear ZY" class="Bool (strict)"() -> ("Value"=w440:bool)  [unwired: 2 in, 2 out]
        n409 = call "Build XY Graph3"("Reset"=w440, "Y Input"=w449, "X Input"=w450) -> ("XY Graph"=→"ZY Graph":cluster{"Y":dbl[], "Y":dbl[]}[])  [unwired: 7 in, 1 out]
        n410 = property on="Y Scan Length SP steps" class="DigNum (strict)"() -> ("Value"=w441:i32)  [unwired: 2 in, 2 out]
        n411 = property on="Z Scan Length SP steps" class="DigNum (strict)"() -> ("Value"=w442:i32)  [unwired: 2 in, 2 out]
        n412 = Divide(x=w441, y=w442) -> (x/y=w443:dbl)
        n413 = Inverse Tangent(1:w443) -> (0:w444:dbl)
        n414 = Divide(x=w444, y=6.283185307179586) -> (x/y=w445:dbl)
        n415 = Multiply(x=360.0, y=w445) -> (x*y=w448:dbl)
        n416 = property on="atan Y/Z" class="DigNum (strict)"("Val(Sgnl)"=w448) -> ()  [unwired: 2 in, 2 out]
      }
      event #1 {
        n417 = event-data() -> ()  [unwired: 1 in, 5 out]
        n418 = property on="Z steps/rev" class="DigNum (strict)"() -> ("Value"=w1045:u32)  [unwired: 2 in, 2 out]
        n419 = property on="R steps/rev" class="DigNum (strict)"() -> ("Value"=w1036:u32)  [unwired: 2 in, 2 out]
        n420 = property on="X steps/rev" class="DigNum (strict)"() -> ("Value"=w1054:u32)  [unwired: 2 in, 2 out]
        n421 = property on="Y steps/rev" class="DigNum (strict)"() -> ("Value"=w1063:u32)  [unwired: 2 in, 2 out]
        n422 = property on="Z offset mm" class="DigNum (strict)"() -> ("Value"=w1043:dbl)  [unwired: 2 in, 2 out]
        n423 = property on="R offset deg" class="DigNum (strict)"() -> ("Value"=w1034:dbl)  [unwired: 2 in, 2 out]
        n424 = property on="X offset mm" class="DigNum (strict)"() -> ("Value"=w1052:dbl)  [unwired: 2 in, 2 out]
        n425 = property on="Y offset mm" class="DigNum (strict)"() -> ("Value"=w1061:dbl)  [unwired: 2 in, 2 out]
        n426 = property on="Reset R Position deg" class="DigNum (strict)"() -> ("Value"=w1042:dbl)  [unwired: 2 in, 2 out]
        n427 = property on="Reset Z Position mm" class="DigNum (strict)"() -> ("Value"=w1051:dbl)  [unwired: 2 in, 2 out]
        n428 = property on="Reset X Position mm" class="DigNum (strict)"() -> ("Value"=w1060:dbl)  [unwired: 2 in, 2 out]
        n429 = property on="Reset Y Position mm" class="DigNum (strict)"() -> ("Value"=w1069:dbl)  [unwired: 2 in, 2 out]
        n430 = To Double Precision Float(number=w1036) -> (double precision float=w1039:dbl)
        n431 = To Double Precision Float(number=w1054) -> (double precision float=w1057:dbl)
        n432 = To Double Precision Float(number=w1063) -> (double precision float=w1066:dbl)
        n433 = Subtract(x=w1051, y=w1043) -> (x-y=w1050:dbl)
        n434 = Subtract(x=w1042, y=w1034) -> (x-y=w1041:dbl)
        n435 = Subtract(x=w1060, y=w1052) -> (x-y=w1059:dbl)
        n436 = Subtract(x=w1069, y=w1061) -> (x-y=w1068:dbl)
        n437 = property on="R deg/rev" class="DigNum (strict)"() -> ("Value"=w1035:dbl)  [unwired: 2 in, 2 out]
        n438 = property on="Z mm/rev" class="DigNum (strict)"() -> ("Value"=w1044:dbl)  [unwired: 2 in, 2 out]
        n439 = property on="X mm/rev" class="DigNum (strict)"() -> ("Value"=w1053:dbl)  [unwired: 2 in, 2 out]
        n440 = property on="Y mm/rev" class="DigNum (strict)"() -> ("Value"=w1062:dbl)  [unwired: 2 in, 2 out]
        n441 = Divide(x=w1041, y=w1035) -> (x/y=w1040:dbl)
        n442 = Divide(x=w1059, y=w1053) -> (x/y=w1058:dbl)
        n443 = Divide(x=w1068, y=w1062) -> (x/y=w1067:dbl)
        n444 = Divide(x=w1050, y=w1044) -> (x/y=w1049:dbl)
        n445 = To Double Precision Float(number=w1045) -> (double precision float=w1048:dbl)
        n446 = Multiply(x=w1049, y=w1048) -> (x*y=w1047:dbl)
        n447 = Multiply(x=w1040, y=w1039) -> (x*y=w1038:dbl)
        n448 = Multiply(x=w1058, y=w1057) -> (x*y=w1056:dbl)
        n449 = Multiply(x=w1067, y=w1066) -> (x*y=w1065:dbl)
        n450 = To Long Integer(number=w1047) -> (32bit integer=w1046:i32)
        n451 = To Long Integer(number=w1038) -> (32bit integer=w1037:i32)
        n452 = To Long Integer(number=w1056) -> (32bit integer=w1055:i32)
        n453 = To Long Integer(number=w1065) -> (32bit integer=w1064:i32)
        n454 = property on="Reset Z Motor Steps" class="DigNum (strict)"("Val(Sgnl)"=w1046) -> ()  [unwired: 2 in, 2 out]
        n455 = property on="Reset R Motor Steps" class="DigNum (strict)"("Val(Sgnl)"=w1037) -> ()  [unwired: 2 in, 2 out]
        n456 = property on="Reset X Motor Steps" class="DigNum (strict)"("Val(Sgnl)"=w1055) -> ()  [unwired: 2 in, 2 out]
        n457 = property on="Reset Y Motor Steps" class="DigNum (strict)"("Val(Sgnl)"=w1064) -> ()  [unwired: 2 in, 2 out]
      }
      event #2 {
        n458 = event-data() -> ()  [unwired: 1 in, 5 out]
        n459 = property on="Y Step SP" class="DigNum (strict)"() -> ("Value"=w1102:i32)  [unwired: 2 in, 2 out]
        n460 = property on="X Step SP" class="DigNum (strict)"() -> ("Value"=w1094:i32)  [unwired: 2 in, 2 out]
        n461 = property on="Z Step SP" class="DigNum (strict)"() -> ("Value"=w1086:i32)  [unwired: 2 in, 2 out]
        n462 = property on="R Step SP" class="DigNum (strict)"() -> ("Value"=w1078:i32)  [unwired: 2 in, 2 out]
        n463 = property on="Y steps/rev" class="DigNum (strict)"() -> ("Value"=w1125:u32)  [unwired: 2 in, 2 out]
        n464 = property on="Y steps/rev" class="DigNum (strict)"() -> ("Value"=w1100:u32)  [unwired: 2 in, 2 out]
        n465 = property on="X steps/rev" class="DigNum (strict)"() -> ("Value"=w1119:u32)  [unwired: 2 in, 2 out]
        n466 = property on="X steps/rev" class="DigNum (strict)"() -> ("Value"=w1092:u32)  [unwired: 2 in, 2 out]
        n467 = property on="Z steps/rev" class="DigNum (strict)"() -> ("Value"=w1113:u32)  [unwired: 2 in, 2 out]
        n468 = property on="Z steps/rev" class="DigNum (strict)"() -> ("Value"=w1084:u32)  [unwired: 2 in, 2 out]
        n469 = property on="R steps/rev" class="DigNum (strict)"() -> ("Value"=w1107:u32)  [unwired: 2 in, 2 out]
        n470 = property on="R steps/rev" class="DigNum (strict)"() -> ("Value"=w1076:u32)  [unwired: 2 in, 2 out]
        n471 = property on="Y offset mm" class="DigNum (strict)"() -> ("Value"=w1099:dbl)  [unwired: 2 in, 2 out]
        n472 = property on="X offset mm" class="DigNum (strict)"() -> ("Value"=w1091:dbl)  [unwired: 2 in, 2 out]
        n473 = property on="Z offset mm" class="DigNum (strict)"() -> ("Value"=w1083:dbl)  [unwired: 2 in, 2 out]
        n474 = property on="R offset deg" class="DigNum (strict)"() -> ("Value"=w1075:dbl)  [unwired: 2 in, 2 out]
        n475 = property on="Y Velocity SP step/sec" class="DigNum (strict)"() -> ("Value"=w1127:i32)  [unwired: 2 in, 2 out]
        n476 = property on="X Velocity SP step/sec" class="DigNum (strict)"() -> ("Value"=w1121:i32)  [unwired: 2 in, 2 out]
        n477 = property on="Z Velocity SP step/sec" class="DigNum (strict)"() -> ("Value"=w1115:i32)  [unwired: 2 in, 2 out]
        n478 = property on="R Velocity SP step/sec" class="DigNum (strict)"() -> ("Value"=w1109:i32)  [unwired: 2 in, 2 out]
        n479 = To Double Precision Float(number=w1102) -> (double precision float=w1103:dbl)
        n480 = To Double Precision Float(number=w1100) -> (double precision float=w1106:dbl)
        n481 = To Double Precision Float(number=w1119) -> (double precision float=w1124:dbl)
        n482 = To Double Precision Float(number=w1094) -> (double precision float=w1095:dbl)
        n483 = To Double Precision Float(number=w1092) -> (double precision float=w1098:dbl)
        n484 = To Double Precision Float(number=w1113) -> (double precision float=w1118:dbl)
        n485 = To Double Precision Float(number=w1086) -> (double precision float=w1087:dbl)
        n486 = To Double Precision Float(number=w1084) -> (double precision float=w1090:dbl)
        n487 = To Double Precision Float(number=w1107) -> (double precision float=w1112:dbl)
        n488 = To Double Precision Float(number=w1078) -> (double precision float=w1079:dbl)
        n489 = To Double Precision Float(number=w1076) -> (double precision float=w1082:dbl)
        n490 = Divide(x=w1079, y=w1082) -> (x/y=w1081:dbl)
        n491 = Divide(x=w1103, y=w1106) -> (x/y=w1105:dbl)
        n492 = Divide(x=w1095, y=w1098) -> (x/y=w1097:dbl)
        n493 = Divide(x=w1087, y=w1090) -> (x/y=w1089:dbl)
        n494 = To Double Precision Float(number=w1109) -> (double precision float=w1110:dbl)
        n495 = To Double Precision Float(number=w1127) -> (double precision float=w1128:dbl)
        n496 = To Double Precision Float(number=w1125) -> (double precision float=w1130:dbl)
        n497 = To Double Precision Float(number=w1121) -> (double precision float=w1122:dbl)
        n498 = To Double Precision Float(number=w1115) -> (double precision float=w1116:dbl)
        n499 = property on="R deg/rev" class="DigNum (strict)"() -> ("Value"=w1074:dbl)  [unwired: 2 in, 2 out]
        n500 = property on="Y mm/rev" class="DigNum (strict)"() -> ("Value"=w1071:dbl)  [unwired: 2 in, 2 out]
        n501 = property on="X mm/rev" class="DigNum (strict)"() -> ("Value"=w1072:dbl)  [unwired: 2 in, 2 out]
        n502 = property on="Z mm/rev" class="DigNum (strict)"() -> ("Value"=w1073:dbl)  [unwired: 2 in, 2 out]
        n503 = Divide(x=w1128, y=w1130) -> (x/y=w1129:dbl)
        n504 = Multiply(x=w1105, y=w1071) -> (x*y=w1104:dbl)
        n505 = Divide(x=w1122, y=w1124) -> (x/y=w1123:dbl)
        n506 = Multiply(x=w1097, y=w1072) -> (x*y=w1096:dbl)
        n507 = Divide(x=w1116, y=w1118) -> (x/y=w1117:dbl)
        n508 = Multiply(x=w1089, y=w1073) -> (x*y=w1088:dbl)
        n509 = Divide(x=w1110, y=w1112) -> (x/y=w1111:dbl)
        n510 = Multiply(x=w1081, y=w1074) -> (x*y=w1080:dbl)
        n511 = Multiply(x=w1129, y=w1071) -> (x*y=w1126:dbl)
        n512 = Add(x=w1104, y=w1099) -> (x+y=w1101:dbl)
        n513 = Multiply(x=w1123, y=w1072) -> (x*y=w1120:dbl)
        n514 = Add(x=w1096, y=w1091) -> (x+y=w1093:dbl)
        n515 = Multiply(x=w1117, y=w1073) -> (x*y=w1114:dbl)
        n516 = Add(x=w1088, y=w1083) -> (x+y=w1085:dbl)
        n517 = Multiply(x=w1111, y=w1074) -> (x*y=w1108:dbl)
        n518 = Add(x=w1080, y=w1075) -> (x+y=w1077:dbl)
        n519 = Absolute Value(x=w1108) -> (abs(x)=w1070:dbl)
        n520 = property on="Y Velocity MV mm/sec" class="DigNum (strict)"("Val(Sgnl)"=w1126) -> ()  [unwired: 2 in, 2 out]
        n521 = property on="Y Position MV mm" class="DigNum (strict)"("Val(Sgnl)"=w1101) -> ()  [unwired: 2 in, 2 out]
        n522 = property on="X Velocity MV mm/sec" class="DigNum (strict)"("Val(Sgnl)"=w1120) -> ()  [unwired: 2 in, 2 out]
        n523 = property on="X Position MV mm" class="DigNum (strict)"("Val(Sgnl)"=w1093) -> ()  [unwired: 2 in, 2 out]
        n524 = property on="Z Velocity MV mm/sec" class="DigNum (strict)"("Val(Sgnl)"=w1114) -> ()  [unwired: 2 in, 2 out]
        n525 = property on="Z Position MV mm" class="DigNum (strict)"("Val(Sgnl)"=w1085) -> ()  [unwired: 2 in, 2 out]
        n526 = property on="R Position MV deg" class="DigNum (strict)"("Val(Sgnl)"=w1077) -> ()  [unwired: 2 in, 2 out]
        n527 = property on="R Velocity MVdeg/sec" class="DigNum (strict)"("Val(Sgnl)"=w1070) -> ()  [unwired: 2 in, 2 out]
      }
      event #3 {
        n528 = event-data() -> ()  [unwired: 1 in, 5 out]
        n529 = property on="X Step PV" class="DigNum (strict)"() -> ("Value"=w1199:i32)  [unwired: 2 in, 2 out]
        n530 = property on="Y Step PV" class="DigNum (strict)"() -> ("Value"=w1185:i32)  [unwired: 2 in, 2 out]
        n531 = property on="Z Step PV" class="DigNum (strict)"() -> ("Value"=w1172:i32)  [unwired: 2 in, 2 out]
        n532 = property on="R Step PV" class="DigNum (strict)"() -> ("Value"=w1158:i32)  [unwired: 2 in, 2 out]
        n533 = property on="X Step SP" class="DigNum (strict)"() -> ("Minimum"=w1206:dbl)  [unwired: 2 in, 2 out]
        n534 = property on="X Step SP" class="DigNum (strict)"() -> ("Maximum"=w1205:dbl)  [unwired: 2 in, 2 out]
        n535 = property on="Y Step SP" class="DigNum (strict)"() -> ("Minimum"=w1192:dbl)  [unwired: 2 in, 2 out]
        n536 = property on="Y Step SP" class="DigNum (strict)"() -> ("Maximum"=w1191:dbl)  [unwired: 2 in, 2 out]
        n537 = property on="Z Step SP" class="DigNum (strict)"() -> ("Minimum"=w1179:dbl)  [unwired: 2 in, 2 out]
        n538 = property on="Z Step SP" class="DigNum (strict)"() -> ("Maximum"=w1178:dbl)  [unwired: 2 in, 2 out]
        n539 = property on="R Step SP" class="DigNum (strict)"() -> ("Minimum"=w1163:dbl)  [unwired: 2 in, 2 out]
        n540 = property on="R Step SP" class="DigNum (strict)"() -> ("Maximum"=w1166:dbl)  [unwired: 2 in, 2 out]
        n541 = property on="Z steps/rev" class="DigNum (strict)"() -> ("Value"=w1174:u32)  [unwired: 2 in, 2 out]
        n542 = property on="R steps/rev" class="DigNum (strict)"() -> ("Value"=w1160:u32)  [unwired: 2 in, 2 out]
        n543 = property on="X steps/rev" class="DigNum (strict)"() -> ("Value"=w1201:u32)  [unwired: 2 in, 2 out]
        n544 = property on="Y steps/rev" class="DigNum (strict)"() -> ("Value"=w1187:u32)  [unwired: 2 in, 2 out]
        n545 = To Double Precision Float(number=w1199) -> (double precision float=w1152:dbl)
        n546 = To Double Precision Float(number=w1185) -> (double precision float=w1151:dbl)
        n547 = To Double Precision Float(number=w1172) -> (double precision float=w1150:dbl)
        n548 = To Double Precision Float(number=w1158) -> (double precision float=w1149:dbl)
        n549 = Subtract(x=w1206, y=w1152) -> (x-y=w1207:dbl)
        n550 = Subtract(x=w1205, y=w1152) -> (x-y=w1204:dbl)
        n551 = Subtract(x=w1192, y=w1151) -> (x-y=w1193:dbl)
        n552 = Subtract(x=w1191, y=w1151) -> (x-y=w1190:dbl)
        n553 = Subtract(x=w1179, y=w1150) -> (x-y=w1180:dbl)
        n554 = Subtract(x=w1178, y=w1150) -> (x-y=w1177:dbl)
        n555 = Subtract(x=w1163, y=w1149) -> (x-y=w1164:dbl)
        n556 = Subtract(x=w1166, y=w1149) -> (x-y=w1165:dbl)
        n557 = property on="Z Scan Length SP steps" class="DigNum (strict)"() -> ("Value"=w1175:i32)  [unwired: 2 in, 2 out]
        n558 = To Double Precision Float(number=w1174) -> (double precision float=w1171:dbl)
        n559 = property on="R Scan Length SP steps" class="DigNum (strict)"() -> ("Value"=w1161:i32)  [unwired: 2 in, 2 out]
        n560 = To Double Precision Float(number=w1160) -> (double precision float=w1157:dbl)
        n561 = property on="X Scan Length SP steps" class="DigNum (strict)"() -> ("Value"=w1197:i32)  [unwired: 2 in, 2 out]
        n562 = To Double Precision Float(number=w1201) -> (double precision float=w1198:dbl)
        n563 = property on="Y Scan Length SP steps" class="DigNum (strict)"() -> ("Value"=w1188:i32)  [unwired: 2 in, 2 out]
        n564 = To Double Precision Float(number=w1187) -> (double precision float=w1142:dbl)
        n565 = property on="Z Scan Velocity SP steps/sec" class="DigNum (strict)"() -> ("Value"=w1170:i32)  [unwired: 2 in, 2 out]
        n566 = property on="R Scan Velocity SP steps/sec" class="DigNum (strict)"() -> ("Value"=w1156:i32)  [unwired: 2 in, 2 out]
        n567 = property on="X Scan Velocity SP steps/sec" class="DigNum (strict)"() -> ("Value"=w1202:i32)  [unwired: 2 in, 2 out]
        n568 = property on="Y Scan Velocity SP steps/sec" class="DigNum (strict)"() -> ("Value"=w1184:i32)  [unwired: 2 in, 2 out]
        n569 = To Double Precision Float(number=w1175) -> (double precision float=w1148:dbl)
        n570 = To Double Precision Float(number=w1161) -> (double precision float=w1146:dbl)
        n571 = property on="X Scan Length SP steps" class="DigNum (strict)"("Minimum"=w1207) -> ()  [unwired: 2 in, 2 out]
        n572 = property on="X Scan Length SP steps" class="DigNum (strict)"("Maximum"=w1204) -> ()  [unwired: 2 in, 2 out]
        n573 = property on="Y Scan Length SP steps" class="DigNum (strict)"("Minimum"=w1193) -> ()  [unwired: 2 in, 2 out]
        n574 = property on="Y Scan Length SP steps" class="DigNum (strict)"("Maximum"=w1190) -> ()  [unwired: 2 in, 2 out]
        n575 = property on="Z Scan Length SP steps" class="DigNum (strict)"("Minimum"=w1180) -> ()  [unwired: 2 in, 2 out]
        n576 = property on="Z Scan Length SP steps" class="DigNum (strict)"("Maximum"=w1177) -> ()  [unwired: 2 in, 2 out]
        n577 = property on="R Scan Length SP steps" class="DigNum (strict)"("Minimum"=w1164) -> ()  [unwired: 2 in, 2 out]
        n578 = property on="R Scan Length SP steps" class="DigNum (strict)"("Maximum"=w1165) -> ()  [unwired: 2 in, 2 out]
        n579 = To Double Precision Float(number=w1197) -> (double precision float=w1137:dbl)
        n580 = To Double Precision Float(number=w1188) -> (double precision float=w1141:dbl)
        n581 = Divide(x=w1146, y=w1157) -> (x/y=w1162:dbl)
        n582 = Divide(x=w1148, y=w1171) -> (x/y=w1176:dbl)
        n583 = Divide(x=w1137, y=w1198) -> (x/y=w1196:dbl)
        n584 = Divide(x=w1141, y=w1142) -> (x/y=w1189:dbl)
        n585 = To Double Precision Float(number=w1156) -> (double precision float=w1145:dbl)
        n586 = property on="R deg/rev" class="DigNum (strict)"() -> ("Value"=w1159:dbl)  [unwired: 2 in, 2 out]
        n587 = To Double Precision Float(number=w1170) -> (double precision float=w1147:dbl)
        n588 = To Double Precision Float(number=w1202) -> (double precision float=w1136:dbl)
        n589 = To Double Precision Float(number=w1184) -> (double precision float=w1140:dbl)
        n590 = property on="Z mm/rev" class="DigNum (strict)"() -> ("Value"=w1173:dbl)  [unwired: 2 in, 2 out]
        n591 = property on="X mm/rev" class="DigNum (strict)"() -> ("Value"=w1200:dbl)  [unwired: 2 in, 2 out]
        n592 = property on="Y mm/rev" class="DigNum (strict)"() -> ("Value"=w1186:dbl)  [unwired: 2 in, 2 out]
        n593 = Divide(x=w1148, y=w1147) -> (x/y=w1143:dbl)
        n594 = Multiply(x=w1176, y=w1173) -> (x*y=w1168:dbl)
        n595 = Divide(x=w1147, y=w1171) -> (x/y=w1169:dbl)
        n596 = Divide(x=w1146, y=w1145) -> (x/y=w1144:dbl)
        n597 = Multiply(x=w1162, y=w1159) -> (x*y=w1154:dbl)
        n598 = Divide(x=w1145, y=w1157) -> (x/y=w1155:dbl)
        n599 = Multiply(x=w1200, y=w1196) -> (x*y=w1194:dbl)
        n600 = Divide(x=w1137, y=w1136) -> (x/y=w1138:dbl)
        n601 = Divide(x=w1136, y=w1198) -> (x/y=w1203:dbl)
        n602 = Divide(x=w1141, y=w1140) -> (x/y=w1139:dbl)
        n603 = Multiply(x=w1189, y=w1186) -> (x*y=w1182:dbl)
        n604 = Divide(x=w1140, y=w1142) -> (x/y=w1183:dbl)
        n605 = Absolute Value(x=w1144) -> (abs(x)=→"R Scan Duration":dbl)
        n606 = Absolute Value(x=w1143) -> (abs(x)=→"Z Scan Duration":dbl)
        n607 = Absolute Value(x=w1138) -> (abs(x)=→"X Scan Duration":dbl)
        n608 = Multiply(x=w1173, y=w1169) -> (x*y=w1167:dbl)
        n609 = Multiply(x=w1159, y=w1155) -> (x*y=w1153:dbl)
        n610 = Multiply(x=w1203, y=w1200) -> (x*y=w1195:dbl)
        n611 = Multiply(x=w1186, y=w1183) -> (x*y=w1181:dbl)
        n612 = Absolute Value(x=w1139) -> (abs(x)=→"Y Scan Duration":dbl)
        n613 = property on="Z Scan length MV mm" class="DigNum (strict)"("Value"=w1168) -> ()  [unwired: 2 in, 2 out]
        n614 = property on="R Scan length MV deg" class="DigNum (strict)"("Value"=w1154) -> ()  [unwired: 2 in, 2 out]
        n615 = property on="X Scan length MV mm" class="DigNum (strict)"("Val(Sgnl)"=w1194) -> ()  [unwired: 2 in, 2 out]
        n616 = property on="Y Scan length MV mm" class="DigNum (strict)"("Value"=w1182) -> ()  [unwired: 2 in, 2 out]
        n617 = property on="Z Scan velocity MV mm/sec" class="DigNum (strict)"("Val(Sgnl)"=w1167) -> ()  [unwired: 2 in, 2 out]
        n618 = property on="X Scan velocity MV mm/sec" class="DigNum (strict)"("Value"=w1195) -> ()  [unwired: 2 in, 2 out]
        n619 = property on="Y Scan velocity MV mm/sec" class="DigNum (strict)"("Val(Sgnl)"=w1181) -> ()  [unwired: 2 in, 2 out]
        n620 = Absolute Value(x=w1153) -> (abs(x)=w1135:dbl)
        n621 = property on="R Scan Velocity SP deg/sec" class="DigNum (strict)"("Val(Sgnl)"=w1135) -> ()  [unwired: 2 in, 2 out]
      }
      event #4 {
        n622 = event-data() -> ()  [unwired: 1 in, 7 out]
        n623 = property on="Y Step SP" class="DigNum (strict)"() -> ("Maximum"=w1218:dbl)  [unwired: 2 in, 2 out]
        n624 = property on="Y Step SP" class="DigNum (strict)"() -> ("Minimum"=w1217:dbl)  [unwired: 2 in, 2 out]
        n625 = property on="Y steps/rev" class="DigNum (strict)"() -> ("Value"=w1224:u32)  [unwired: 2 in, 2 out]
        n626 = property on="Y offset mm" class="DigNum (strict)"() -> ("Value"=w1222:dbl)  [unwired: 2 in, 2 out]
        n627 = property on="Y Velocity SP step/sec" class="DigNum (strict)"() -> ("Maximum"=w1211:dbl)  [unwired: 2 in, 2 out]
        n628 = property on="Y Velocity SP step/sec" class="DigNum (strict)"() -> ("Minimum"=w1210:dbl)  [unwired: 2 in, 2 out]
        n629 = property on="Y Position SP mm" class="DigNum (strict)"() -> ("Value"=w1221:dbl)  [unwired: 2 in, 2 out]
        n630 = property on="Y mm/rev" class="DigNum (strict)"() -> ("Value"=w1208:dbl)  [unwired: 2 in, 2 out]
        n631 = property on="Y Velocity SP mm/sec" class="DigNum (strict)"() -> ("Value"=w1215:dbl)  [unwired: 2 in, 2 out]
        n632 = Subtract(x=w1221, y=w1222) -> (x-y=w1225:dbl)
        n633 = Divide(x=w1215, y=w1208) -> (x/y=w1216:dbl)
        n634 = To Double Precision Float(number=w1224) -> (double precision float=w1209:dbl)
        n635 = Divide(x=w1225, y=w1208) -> (x/y=w1226:dbl)
        n636 = Multiply(x=w1216, y=w1209) -> (x*y=w1213:dbl)
        n637 = Multiply(x=w1226, y=w1209) -> (x*y=w1220:dbl)
        n638 = In Range and Coerce(upper limit=w1211, x=w1213, lower limit=w1210) -> (coerced(x)=w1212:dbl)  [unwired: 1 out]
        n639 = To Long Integer(number=w1212) -> (32bit integer=w1214:i32)
        n640 = In Range and Coerce(upper limit=w1218, x=w1220, lower limit=w1217) -> (coerced(x)=w1219:dbl)  [unwired: 1 out]
        n641 = To Long Integer(number=w1219) -> (32bit integer=w1223:i32)
        n642 = property on="Y Velocity SP step/sec" class="DigNum (strict)"("Val(Sgnl)"=w1214) -> ()  [unwired: 2 in, 2 out]
        n643 = property on="Y Step SP" class="DigNum (strict)"("Val(Sgnl)"=w1223) -> ()  [unwired: 2 in, 2 out]
      }
      event #5 {
        n644 = event-data() -> ()  [unwired: 1 in, 7 out]
        n645 = property on="X Step SP" class="DigNum (strict)"() -> ("Maximum"=w1237:dbl)  [unwired: 2 in, 2 out]
        n646 = property on="X Step SP" class="DigNum (strict)"() -> ("Minimum"=w1236:dbl)  [unwired: 2 in, 2 out]
        n647 = property on="X steps/rev" class="DigNum (strict)"() -> ("Value"=w1243:u32)  [unwired: 2 in, 2 out]
        n648 = property on="X offset mm" class="DigNum (strict)"() -> ("Value"=w1241:dbl)  [unwired: 2 in, 2 out]
        n649 = property on="X Velocity SP step/sec" class="DigNum (strict)"() -> ("Maximum"=w1230:dbl)  [unwired: 2 in, 2 out]
        n650 = property on="X Velocity SP step/sec" class="DigNum (strict)"() -> ("Minimum"=w1229:dbl)  [unwired: 2 in, 2 out]
        n651 = property on="X Position SP mm" class="DigNum (strict)"() -> ("Value"=w1240:dbl)  [unwired: 2 in, 2 out]
        n652 = property on="X mm/rev" class="DigNum (strict)"() -> ("Value"=w1227:dbl)  [unwired: 2 in, 2 out]
        n653 = property on="X Velocity SP mm/sec" class="DigNum (strict)"() -> ("Value"=w1234:dbl)  [unwired: 2 in, 2 out]
        n654 = Subtract(x=w1240, y=w1241) -> (x-y=w1244:dbl)
        n655 = Divide(x=w1234, y=w1227) -> (x/y=w1235:dbl)
        n656 = To Double Precision Float(number=w1243) -> (double precision float=w1228:dbl)
        n657 = Divide(x=w1244, y=w1227) -> (x/y=w1245:dbl)
        n658 = Multiply(x=w1235, y=w1228) -> (x*y=w1232:dbl)
        n659 = Multiply(x=w1245, y=w1228) -> (x*y=w1239:dbl)
        n660 = In Range and Coerce(upper limit=w1230, x=w1232, lower limit=w1229) -> (coerced(x)=w1231:dbl)  [unwired: 1 out]
        n661 = To Long Integer(number=w1231) -> (32bit integer=w1233:i32)
        n662 = In Range and Coerce(upper limit=w1237, x=w1239, lower limit=w1236) -> (coerced(x)=w1238:dbl)  [unwired: 1 out]
        n663 = To Long Integer(number=w1238) -> (32bit integer=w1242:i32)
        n664 = property on="X Velocity SP step/sec" class="DigNum (strict)"("Val(Sgnl)"=w1233) -> ()  [unwired: 2 in, 2 out]
        n665 = property on="X Step SP" class="DigNum (strict)"("Val(Sgnl)"=w1242) -> ()  [unwired: 2 in, 2 out]
      }
      event #6 {
        n666 = event-data() -> ()  [unwired: 1 in, 7 out]
        n667 = property on="Z Step SP" class="DigNum (strict)"() -> ("Maximum"=w1254:dbl)  [unwired: 2 in, 2 out]
        n668 = property on="Z Step SP" class="DigNum (strict)"() -> ("Minimum"=w1253:dbl)  [unwired: 2 in, 2 out]
        n669 = property on="Z steps/rev" class="DigNum (strict)"() -> ("Value"=w1260:u32)  [unwired: 2 in, 2 out]
        n670 = property on="Z offset mm" class="DigNum (strict)"() -> ("Value"=w1258:dbl)  [unwired: 2 in, 2 out]
        n671 = property on="Z Velocity SP step/sec" class="DigNum (strict)"() -> ("Maximum"=w1247:dbl)  [unwired: 2 in, 2 out]
        n672 = property on="Z Velocity SP step/sec" class="DigNum (strict)"() -> ("Minimum"=w1246:dbl)  [unwired: 2 in, 2 out]
        n673 = property on="Z Position SP mm" class="DigNum (strict)"() -> ("Value"=w1257:dbl)  [unwired: 2 in, 2 out]
        n674 = property on="Z mm/rev" class="DigNum (strict)"() -> ("Value"=w1263:dbl)  [unwired: 2 in, 2 out]
        n675 = property on="Z Velocity SP mm/sec" class="DigNum (strict)"() -> ("Value"=w1251:dbl)  [unwired: 2 in, 2 out]
        n676 = Subtract(x=w1257, y=w1258) -> (x-y=w1261:dbl)
        n677 = Divide(x=w1251, y=w1263) -> (x/y=w1252:dbl)
        n678 = To Double Precision Float(number=w1260) -> (double precision float=w1264:dbl)
        n679 = Divide(x=w1261, y=w1263) -> (x/y=w1262:dbl)
        n680 = Multiply(x=w1252, y=w1264) -> (x*y=w1249:dbl)
        n681 = Multiply(x=w1262, y=w1264) -> (x*y=w1256:dbl)
        n682 = In Range and Coerce(upper limit=w1247, x=w1249, lower limit=w1246) -> (coerced(x)=w1248:dbl)  [unwired: 1 out]
        n683 = To Long Integer(number=w1248) -> (32bit integer=w1250:i32)
        n684 = In Range and Coerce(upper limit=w1254, x=w1256, lower limit=w1253) -> (coerced(x)=w1255:dbl)  [unwired: 1 out]
        n685 = To Long Integer(number=w1255) -> (32bit integer=w1259:i32)
        n686 = property on="Z Velocity SP step/sec" class="DigNum (strict)"("Val(Sgnl)"=w1250) -> ()  [unwired: 2 in, 2 out]
        n687 = property on="Z Step SP" class="DigNum (strict)"("Val(Sgnl)"=w1259) -> ()  [unwired: 2 in, 2 out]
      }
      event #7 {
        n688 = event-data() -> ()  [unwired: 1 in, 7 out]
        n689 = property on="R Step SP" class="DigNum (strict)"() -> ("Maximum"=w1276:dbl)  [unwired: 2 in, 2 out]
        n690 = property on="R Step SP" class="DigNum (strict)"() -> ("Minimum"=w1275:dbl)  [unwired: 2 in, 2 out]
        n691 = property on="R steps/rev" class="DigNum (strict)"() -> ("Value"=w1282:u32)  [unwired: 2 in, 2 out]
        n692 = property on="R offset deg" class="DigNum (strict)"() -> ("Value"=w1280:dbl)  [unwired: 2 in, 2 out]
        n693 = property on="R Velocity SP step/sec" class="DigNum (strict)"() -> ("Maximum"=w1269:dbl)  [unwired: 2 in, 2 out]
        n694 = property on="R Velocity SP step/sec" class="DigNum (strict)"() -> ("Minimum"=w1268:dbl)  [unwired: 2 in, 2 out]
        n695 = property on="R Position SP deg" class="DigNum (strict)"() -> ("Value"=w1279:dbl)  [unwired: 2 in, 2 out]
        n696 = property on="R deg/rev" class="DigNum (strict)"() -> ("Value"=w1266:dbl)  [unwired: 2 in, 2 out]
        n697 = property on="R Velocity SP deg/sec" class="DigNum (strict)"() -> ("Value"=w1273:dbl)  [unwired: 2 in, 2 out]
        n698 = Subtract(x=w1279, y=w1280) -> (x-y=w1283:dbl)
        n699 = Divide(x=w1273, y=w1266) -> (x/y=w1274:dbl)
        n700 = To Double Precision Float(number=w1282) -> (double precision float=w1267:dbl)
        n701 = Divide(x=w1283, y=w1266) -> (x/y=w1284:dbl)
        n702 = Multiply(x=w1274, y=w1267) -> (x*y=w1271:dbl)
        n703 = Multiply(x=w1284, y=w1267) -> (x*y=w1278:dbl)
        n704 = Absolute Value(x=w1271) -> (abs(x)=w1265:dbl)
        n705 = In Range and Coerce(upper limit=w1276, x=w1278, lower limit=w1275) -> (coerced(x)=w1277:dbl)  [unwired: 1 out]
        n706 = In Range and Coerce(upper limit=w1269, x=w1265, lower limit=w1268) -> (coerced(x)=w1270:dbl)  [unwired: 1 out]
        n707 = To Long Integer(number=w1277) -> (32bit integer=w1281:i32)
        n708 = To Long Integer(number=w1270) -> (32bit integer=w1272:i32)
        n709 = property on="R Step SP" class="DigNum (strict)"("Val(Sgnl)"=w1281) -> ()  [unwired: 2 in, 2 out]
        n710 = property on="R Velocity SP step/sec" class="DigNum (strict)"("Val(Sgnl)"=w1272) -> ()  [unwired: 2 in, 2 out]
      }
      event #8 {
        n711 = event-data() -> ()  [unwired: 1 in, 7 out]
        n712 = property on="Y Step SP" class="DigNum (strict)"() -> ("Maximum"=w1294:dbl)  [unwired: 2 in, 2 out]
        n713 = property on="Y Step SP" class="DigNum (strict)"() -> ("Minimum"=w1295:dbl)  [unwired: 2 in, 2 out]
        n714 = property on="Y steps/rev" class="DigNum (strict)"() -> ("Value"=w1300:u32)  [unwired: 2 in, 2 out]
        n715 = To Double Precision Float(number=w1300) -> (double precision float=w1286:dbl)
        n716 = property on="Y Scan Length SP mm" class="DigNum (strict)"() -> ("Value"=w1298:dbl)  [unwired: 2 in, 2 out]
        n717 = property on="Y mm/rev" class="DigNum (strict)"() -> ("Value"=w1285:dbl)  [unwired: 2 in, 2 out]
        n718 = property on="Y Scan Velocity SP steps/sec" class="DigNum (strict)"() -> ("Maximum"=w1288:dbl)  [unwired: 2 in, 2 out]
        n719 = property on="Y Scan Velocity SP steps/sec" class="DigNum (strict)"() -> ("Minimum"=w1287:dbl)  [unwired: 2 in, 2 out]
        n720 = property on="Y Scan Velocity SP mm/sec" class="DigNum (strict)"() -> ("Value"=w1292:dbl)  [unwired: 2 in, 2 out]
        n721 = Divide(x=w1298, y=w1285) -> (x/y=w1301:dbl)
        n722 = Multiply(x=w1301, y=w1286) -> (x*y=w1297:dbl)
        n723 = Divide(x=w1292, y=w1285) -> (x/y=w1293:dbl)
        n724 = Multiply(x=w1293, y=w1286) -> (x*y=w1290:dbl)
        n725 = In Range and Coerce(upper limit=w1294, x=w1297, lower limit=w1295) -> (coerced(x)=w1296:dbl)  [unwired: 1 out]
        n726 = To Long Integer(number=w1296) -> (32bit integer=w1299:i32)
        n727 = In Range and Coerce(upper limit=w1288, x=w1290, lower limit=w1287) -> (coerced(x)=w1289:dbl)  [unwired: 1 out]
        n728 = To Long Integer(number=w1289) -> (32bit integer=w1291:i32)
        n729 = property on="Y Scan Length SP steps" class="DigNum (strict)"("Val(Sgnl)"=w1299) -> ()  [unwired: 2 in, 2 out]
        n730 = property on="Y Scan Velocity SP steps/sec" class="DigNum (strict)"("Val(Sgnl)"=w1291) -> ()  [unwired: 2 in, 2 out]
      }
      event #9 {
        n731 = event-data() -> ()  [unwired: 1 in, 7 out]
        n732 = property on="X Step SP" class="DigNum (strict)"() -> ("Maximum"=w1311:dbl)  [unwired: 2 in, 2 out]
        n733 = property on="X Step SP" class="DigNum (strict)"() -> ("Minimum"=w1312:dbl)  [unwired: 2 in, 2 out]
        n734 = property on="X steps/rev" class="DigNum (strict)"() -> ("Value"=w1317:u32)  [unwired: 2 in, 2 out]
        n735 = To Double Precision Float(number=w1317) -> (double precision float=w1303:dbl)
        n736 = property on="X Scan Length SP mm" class="DigNum (strict)"() -> ("Value"=w1315:dbl)  [unwired: 2 in, 2 out]
        n737 = property on="X mm/rev" class="DigNum (strict)"() -> ("Value"=w1302:dbl)  [unwired: 2 in, 2 out]
        n738 = property on="X Scan Velocity SP steps/sec" class="DigNum (strict)"() -> ("Maximum"=w1305:dbl)  [unwired: 2 in, 2 out]
        n739 = property on="X Scan Velocity SP steps/sec" class="DigNum (strict)"() -> ("Minimum"=w1304:dbl)  [unwired: 2 in, 2 out]
        n740 = property on="X Scan Velocity SP mm/sec" class="DigNum (strict)"() -> ("Value"=w1309:dbl)  [unwired: 2 in, 2 out]
        n741 = Divide(x=w1315, y=w1302) -> (x/y=w1318:dbl)
        n742 = Multiply(x=w1318, y=w1303) -> (x*y=w1314:dbl)
        n743 = Divide(x=w1309, y=w1302) -> (x/y=w1310:dbl)
        n744 = Multiply(x=w1310, y=w1303) -> (x*y=w1307:dbl)
        n745 = In Range and Coerce(upper limit=w1311, x=w1314, lower limit=w1312) -> (coerced(x)=w1313:dbl)  [unwired: 1 out]
        n746 = To Long Integer(number=w1313) -> (32bit integer=w1316:i32)
        n747 = In Range and Coerce(upper limit=w1305, x=w1307, lower limit=w1304) -> (coerced(x)=w1306:dbl)  [unwired: 1 out]
        n748 = To Long Integer(number=w1306) -> (32bit integer=w1308:i32)
        n749 = property on="X Scan Length SP steps" class="DigNum (strict)"("Val(Sgnl)"=w1316) -> ()  [unwired: 2 in, 2 out]
        n750 = property on="X Scan Velocity SP steps/sec" class="DigNum (strict)"("Val(Sgnl)"=w1308) -> ()  [unwired: 2 in, 2 out]
      }
      event #10 {
        n751 = event-data() -> ()  [unwired: 1 in, 7 out]
        n752 = property on="Z Step SP" class="DigNum (strict)"() -> ("Maximum"=w1328:dbl)  [unwired: 2 in, 2 out]
        n753 = property on="Z Step SP" class="DigNum (strict)"() -> ("Minimum"=w1329:dbl)  [unwired: 2 in, 2 out]
        n754 = property on="Z steps/rev" class="DigNum (strict)"() -> ("Value"=w1334:u32)  [unwired: 2 in, 2 out]
        n755 = property on="Z Scan Length SP mm" class="DigNum (strict)"() -> ("Value"=w1332:dbl)  [unwired: 2 in, 2 out]
        n756 = property on="Z mm/rev" class="DigNum (strict)"() -> ("Value"=w1319:dbl)  [unwired: 2 in, 2 out]
        n757 = property on="Z Scan Velocity SP steps/sec" class="DigNum (strict)"() -> ("Maximum"=w1322:dbl)  [unwired: 2 in, 2 out]
        n758 = property on="Z Scan Velocity SP steps/sec" class="DigNum (strict)"() -> ("Minimum"=w1321:dbl)  [unwired: 2 in, 2 out]
        n759 = property on="Z Scan Velocity SP mm/sec" class="DigNum (strict)"() -> ("Value"=w1326:dbl)  [unwired: 2 in, 2 out]
        n760 = Divide(x=w1332, y=w1319) -> (x/y=w1335:dbl)
        n761 = To Double Precision Float(number=w1334) -> (double precision float=w1320:dbl)
        n762 = Multiply(x=w1335, y=w1320) -> (x*y=w1331:dbl)
        n763 = Divide(x=w1326, y=w1319) -> (x/y=w1327:dbl)
        n764 = Multiply(x=w1327, y=w1320) -> (x*y=w1324:dbl)
        n765 = In Range and Coerce(upper limit=w1328, x=w1331, lower limit=w1329) -> (coerced(x)=w1330:dbl)  [unwired: 1 out]
        n766 = To Long Integer(number=w1330) -> (32bit integer=w1333:i32)
        n767 = In Range and Coerce(upper limit=w1322, x=w1324, lower limit=w1321) -> (coerced(x)=w1323:dbl)  [unwired: 1 out]
        n768 = To Long Integer(number=w1323) -> (32bit integer=w1325:i32)
        n769 = property on="Z Scan Length SP steps" class="DigNum (strict)"("Val(Sgnl)"=w1333) -> ()  [unwired: 2 in, 2 out]
        n770 = property on="Z Scan Velocity SP steps/sec" class="DigNum (strict)"("Val(Sgnl)"=w1325) -> ()  [unwired: 2 in, 2 out]
      }
      event #11 {
        n771 = event-data() -> ()  [unwired: 1 in, 7 out]
        n772 = property on="R Step SP" class="DigNum (strict)"() -> ("Maximum"=w1346:dbl)  [unwired: 2 in, 2 out]
        n773 = property on="R Step SP" class="DigNum (strict)"() -> ("Minimum"=w1347:dbl)  [unwired: 2 in, 2 out]
        n774 = property on="R steps/rev" class="DigNum (strict)"() -> ("Value"=w1352:u32)  [unwired: 2 in, 2 out]
        n775 = property on="R Velocity SP step/sec" class="DigNum (strict)"() -> ("Maximum"=w1340:dbl)  [unwired: 2 in, 2 out]
        n776 = property on="R Scan Length SP deg" class="DigNum (strict)"() -> ("Value"=w1350:dbl)  [unwired: 2 in, 2 out]
        n777 = property on="R deg/rev" class="DigNum (strict)"() -> ("Value"=w1337:dbl)  [unwired: 2 in, 2 out]
        n778 = property on="R Scan Velocity SP steps/sec" class="DigNum (strict)"() -> ("Minimum"=w1339:dbl)  [unwired: 2 in, 2 out]
        n779 = property on="R Scan Velocity SP deg/sec" class="DigNum (strict)"() -> ("Value"=w1344:dbl)  [unwired: 2 in, 2 out]
        n780 = Divide(x=w1350, y=w1337) -> (x/y=w1353:dbl)
        n781 = To Double Precision Float(number=w1352) -> (double precision float=w1338:dbl)
        n782 = Multiply(x=w1353, y=w1338) -> (x*y=w1349:dbl)
        n783 = Divide(x=w1344, y=w1337) -> (x/y=w1345:dbl)
        n784 = Multiply(x=w1345, y=w1338) -> (x*y=w1342:dbl)
        n785 = In Range and Coerce(upper limit=w1346, x=w1349, lower limit=w1347) -> (coerced(x)=w1348:dbl)  [unwired: 1 out]
        n786 = To Long Integer(number=w1348) -> (32bit integer=w1351:i32)
        n787 = Absolute Value(x=w1342) -> (abs(x)=w1336:dbl)
        n788 = property on="R Scan Length SP steps" class="DigNum (strict)"("Val(Sgnl)"=w1351) -> ()  [unwired: 2 in, 2 out]
        n789 = In Range and Coerce(upper limit=w1340, x=w1336, lower limit=w1339) -> (coerced(x)=w1341:dbl)  [unwired: 1 out]
        n790 = To Long Integer(number=w1341) -> (32bit integer=w1343:i32)
        n791 = property on="R Scan Velocity SP steps/sec" class="DigNum (strict)"("Val(Sgnl)"=w1343) -> ()  [unwired: 2 in, 2 out]
      }
      event #12 {
        n792 = event-data() -> ()  [unwired: 1 in, 7 out]
        n793 = flat-sequence {
          tunnel: w1358 -> [w1368]
          tunnel: w1359 -> [w1369]
          tunnel: [w1369] -> w1355
          tunnel: [w1368] -> w1354
          tunnel: [w1372] -> w1357
          tunnel: [w1371] -> w1356
          tunnel: w1355 -> [w1374]
          tunnel: w1354 -> [w1373]
          tunnel: [w1392] -> w1361
          tunnel: [w1391] -> w1360
          tunnel: w1357 -> [w1390]
          tunnel: w1356 -> [w1389]
          tunnel: [w1399] -> w1363
          tunnel: [w1398] -> w1362
          tunnel: w1361 -> [w1397]
          tunnel: w1360 -> [w1396]
          tunnel: [w1405] -> w1364
          tunnel: [w1406] -> w1365
          tunnel: w1363 -> [w1406]
          tunnel: w1362 -> [w1404]
          frame #0 {
            n794 = property on="Y Go" class="Bool"("DisabledEnum"=T2."Disabled and Grayed Out" ("Disabled")) -> ()  [unwired: 2 in, 2 out]
            n795 = property on="Scan Go" class="Bool"("DisabledEnum"=T2."Disabled and Grayed Out" ("Disabled")) -> ()  [unwired: 2 in, 2 out]
          }
          frame #1 {
            n796 = property on="Y Step SP" class="DigNum (strict)"() -> ("Value"=w1382:i32)  [unwired: 2 in, 2 out]
            n797 = property on="Y Step PV" class="DigNum (strict)"() -> ("Value"=w1381:i32)  [unwired: 2 in, 2 out]
            n798 = property on="Y Backlash" class="DigNum (strict)"() -> ("Value"=w1370:i32)  [unwired: 2 in, 2 out]
            n799 = Subtract(x=w1382, y=w1381) -> (x-y=w1380:i32)
            n800 = Sign(1:w1370) -> (0:w1378:i32)
            n801 = Sign(1:w1380) -> (0:w1379:i32)
            n802 = Multiply(x=w1379, y=w1378) -> (x*y=w1377:i32)
            n803 = Equal?(x=w1377, y=1) -> (x = y?=w1375:bool)
            n804 = case shown="False" w1375 {
              tunnel: w1374 -> [w1385 w1387]
              tunnel: w1373 -> [w1384 w1386]
              tunnel: [w1384 w1386] -> w1372
              tunnel: [w1385 w1387] -> w1371
              frame #0 {
                n805 = property on="Y Backlash corr" class="Bool (strict)"("Val(Sgnl)"=FALSE ("Value (Signaling)")) -> ()  [unwired: 2 in, 2 out]
              }
              frame #1 {
                n806 = property on="Y Backlash corr" class="Bool (strict)"("Val(Sgnl)"=TRUE ("Value (Signaling)")) -> ()  [unwired: 2 in, 2 out]
              }
            }
          }
          frame #2 {
            # "Velocity Setting"
            n807 = property on="Y Velocity SP step/sec" class="DigNum (strict)"() -> ("Value"=w1393:i32)  [unwired: 2 in, 2 out]
            n808 = Number To Decimal String(number=w1393) -> (decimal integer string=w1394:string)  [unwired: 1 in]
            n809 = call "mDrive Send Command.vi"("error in (no error)"=w1390, "Extra"=w1394, "Command"=T1."Max Velocity", "VISA resource name"=w1389) -> ("error out"=w1391:errorcluster, "VISA resource name out"=w1392:refnum<visa-resource-name>)  [unwired: 3 in, 1 out]
          }
          frame #3 {
            # "Move to Abs Position"
            n810 = property on="Y Step SP" class="DigNum (strict)"() -> ("Value"=w1402:i32)  [unwired: 2 in, 2 out]
            n811 = Number To Decimal String(number=w1402) -> (decimal integer string=w1401:string)  [unwired: 1 in]
            n812 = call "mDrive Send Command.vi"("error in (no error)"=w1396, "Extra"=w1401, "Command"=T1."Move to Absolute Position", "VISA resource name"=w1397) -> ("error out"=w1398:errorcluster, "VISA resource name out"=w1399:refnum<visa-resource-name>)  [unwired: 3 in, 1 out]
          }
          frame #4 {
            n813 = call "Time Delay"("error in (no error)"=w1404, "Delay Time (s)"=0.1) -> ("error out"=w1405:errorcluster)  [unwired: 9 in]
          }
        }
      }
      event #13 {
        n814 = event-data() -> ()  [unwired: 1 in, 7 out]
        n815 = flat-sequence {
          tunnel: w1409 -> [w1421]
          tunnel: w1410 -> [w1422]
          tunnel: [w1422] -> w1412
          tunnel: [w1421] -> w1411
          tunnel: [w1425] -> w1414
          tunnel: [w1424] -> w1413
          tunnel: w1412 -> [w1427]
          tunnel: w1411 -> [w1426]
          tunnel: [w1445] -> w1416
          tunnel: [w1444] -> w1415
          tunnel: w1414 -> [w1443]
          tunnel: w1413 -> [w1442]
          tunnel: [w1452] -> w1418
          tunnel: [w1451] -> w1417
          tunnel: w1416 -> [w1450]
          tunnel: w1415 -> [w1449]
          tunnel: [w1458] -> w1408
          tunnel: [w1459] -> w1407
          tunnel: w1418 -> [w1459]
          tunnel: w1417 -> [w1457]
          frame #0 {
            n816 = property on="Z Go" class="Bool"("DisabledEnum"=T2."Disabled and Grayed Out" ("Disabled")) -> ()  [unwired: 2 in, 2 out]
            n817 = property on="Scan Go" class="Bool"("DisabledEnum"=T2."Disabled and Grayed Out" ("Disabled")) -> ()  [unwired: 2 in, 2 out]
          }
          frame #1 {
            n818 = property on="Z Step SP" class="DigNum (strict)"() -> ("Value"=w1435:i32)  [unwired: 2 in, 2 out]
            n819 = property on="Z Step PV" class="DigNum (strict)"() -> ("Value"=w1434:i32)  [unwired: 2 in, 2 out]
            n820 = property on="Z Backlash" class="DigNum (strict)"() -> ("Value"=w1423:i32)  [unwired: 2 in, 2 out]
            n821 = Subtract(x=w1435, y=w1434) -> (x-y=w1433:i32)
            n822 = Sign(1:w1423) -> (0:w1431:i32)
            n823 = Sign(1:w1433) -> (0:w1432:i32)
            n824 = Multiply(x=w1432, y=w1431) -> (x*y=w1430:i32)
            n825 = Equal?(x=w1430, y=1) -> (x = y?=w1428:bool)
            n826 = case shown="True" w1428 {
              tunnel: w1427 -> [w1438 w1440]
              tunnel: w1426 -> [w1437 w1439]
              tunnel: [w1437 w1439] -> w1425
              tunnel: [w1438 w1440] -> w1424
              frame #0 {
                n827 = property on="Z Backlash corr" class="Bool (strict)"("Val(Sgnl)"=FALSE ("Value (Signaling)")) -> ()  [unwired: 2 in, 2 out]
              }
              frame #1 {
                n828 = property on="Z Backlash corr" class="Bool (strict)"("Val(Sgnl)"=TRUE ("Value (Signaling)")) -> ()  [unwired: 2 in, 2 out]
              }
            }
          }
          frame #2 {
            # "Velocity Setting"
            n829 = property on="Z Velocity SP step/sec" class="DigNum (strict)"() -> ("Value"=w1446:i32)  [unwired: 2 in, 2 out]
            n830 = Number To Decimal String(number=w1446) -> (decimal integer string=w1447:string)  [unwired: 1 in]
            n831 = call "mDrive Send Command.vi"("error in (no error)"=w1443, "Extra"=w1447, "Command"=T1."Max Velocity", "VISA resource name"=w1442) -> ("error out"=w1444:errorcluster, "VISA resource name out"=w1445:refnum<visa-resource-name>)  [unwired: 3 in, 1 out]
          }
          frame #3 {
            # "Move to Abs Position"
            n832 = property on="Z Step SP" class="DigNum (strict)"() -> ("Value"=w1455:i32)  [unwired: 2 in, 2 out]
            n833 = Number To Decimal String(number=w1455) -> (decimal integer string=w1454:string)  [unwired: 1 in]
            n834 = call "mDrive Send Command.vi"("error in (no error)"=w1449, "Extra"=w1454, "Command"=T1."Move to Absolute Position", "VISA resource name"=w1450) -> ("error out"=w1451:errorcluster, "VISA resource name out"=w1452:refnum<visa-resource-name>)  [unwired: 3 in, 1 out]
          }
          frame #4 {
            n835 = call "Time Delay28"("error in (no error)"=w1457, "Delay Time (s)"=0.1) -> ("error out"=w1458:errorcluster)  [unwired: 9 in]
          }
        }
      }
      event #14 {
        n836 = event-data() -> ()  [unwired: 1 in, 7 out]
        n837 = flat-sequence {
          tunnel: w1462 -> [w1474]
          tunnel: w1463 -> [w1475]
          tunnel: [w1475] -> w1465
          tunnel: [w1474] -> w1464
          tunnel: [w1478] -> w1467
          tunnel: [w1477] -> w1466
          tunnel: w1465 -> [w1480]
          tunnel: w1464 -> [w1479]
          tunnel: [w1498] -> w1469
          tunnel: [w1497] -> w1468
          tunnel: w1467 -> [w1496]
          tunnel: w1466 -> [w1495]
          tunnel: [w1505] -> w1471
          tunnel: [w1504] -> w1470
          tunnel: w1469 -> [w1503]
          tunnel: w1468 -> [w1502]
          tunnel: [w1511] -> w1461
          tunnel: [w1512] -> w1460
          tunnel: w1471 -> [w1512]
          tunnel: w1470 -> [w1510]
          frame #0 {
            n838 = property on="R Go" class="Bool"("DisabledEnum"=T2."Disabled and Grayed Out" ("Disabled")) -> ()  [unwired: 2 in, 2 out]
            n839 = property on="Scan Go" class="Bool"("DisabledEnum"=T2."Disabled and Grayed Out" ("Disabled")) -> ()  [unwired: 2 in, 2 out]
          }
          frame #1 {
            n840 = property on="R Step SP" class="DigNum (strict)"() -> ("Value"=w1488:i32)  [unwired: 2 in, 2 out]
            n841 = property on="R Step PV" class="DigNum (strict)"() -> ("Value"=w1487:i32)  [unwired: 2 in, 2 out]
            n842 = property on="R Backlash" class="DigNum (strict)"() -> ("Value"=w1476:i32)  [unwired: 2 in, 2 out]
            n843 = Subtract(x=w1488, y=w1487) -> (x-y=w1486:i32)
            n844 = Sign(1:w1476) -> (0:w1484:i32)
            n845 = Sign(1:w1486) -> (0:w1485:i32)
            n846 = Multiply(x=w1485, y=w1484) -> (x*y=w1483:i32)
            n847 = Equal?(x=w1483, y=1) -> (x = y?=w1481:bool)
            n848 = case shown="True" w1481 {
              tunnel: w1480 -> [w1491 w1493]
              tunnel: w1479 -> [w1490 w1492]
              tunnel: [w1490 w1492] -> w1478
              tunnel: [w1491 w1493] -> w1477
              frame #0 {
                n849 = property on="R Backlash corr" class="Bool (strict)"("Val(Sgnl)"=FALSE ("Value (Signaling)")) -> ()  [unwired: 2 in, 2 out]
              }
              frame #1 {
                n850 = property on="R Backlash corr" class="Bool (strict)"("Val(Sgnl)"=TRUE ("Value (Signaling)")) -> ()  [unwired: 2 in, 2 out]
              }
            }
          }
          frame #2 {
            # "Velocity Setting"
            n851 = property on="R Velocity SP step/sec" class="DigNum (strict)"() -> ("Value"=w1499:i32)  [unwired: 2 in, 2 out]
            n852 = Number To Decimal String(number=w1499) -> (decimal integer string=w1500:string)  [unwired: 1 in]
            n853 = call "mDrive Send Command.vi"("error in (no error)"=w1496, "Extra"=w1500, "Command"=T1."Max Velocity", "VISA resource name"=w1495) -> ("error out"=w1497:errorcluster, "VISA resource name out"=w1498:refnum<visa-resource-name>)  [unwired: 3 in, 1 out]
          }
          frame #3 {
            # "Move to Abs Position"
            n854 = property on="R Step SP" class="DigNum (strict)"() -> ("Value"=w1508:i32)  [unwired: 2 in, 2 out]
            n855 = Number To Decimal String(number=w1508) -> (decimal integer string=w1507:string)  [unwired: 1 in]
            n856 = call "mDrive Send Command.vi"("error in (no error)"=w1502, "Extra"=w1507, "Command"=T1."Move to Absolute Position", "VISA resource name"=w1503) -> ("error out"=w1504:errorcluster, "VISA resource name out"=w1505:refnum<visa-resource-name>)  [unwired: 3 in, 1 out]
          }
          frame #4 {
            n857 = call "Time Delay29"("error in (no error)"=w1510, "Delay Time (s)"=0.1) -> ("error out"=w1511:errorcluster)  [unwired: 9 in]
          }
        }
      }
      event #15 {
        n858 = event-data() -> ()  [unwired: 1 in, 7 out]
        n859 = flat-sequence {
          tunnel: [w1526] -> w1518
          tunnel: [w1525] -> w1517
          tunnel: w1516 -> [w1526]
          tunnel: w1515 -> [w1525]
          tunnel: [w1531] -> w1520
          tunnel: [w1530] -> w1519
          tunnel: w1518 -> [w1533]
          tunnel: w1517 -> [w1532]
          tunnel: [w1551] -> w1522
          tunnel: [w1550] -> w1521
          tunnel: w1520 -> [w1549]
          tunnel: w1519 -> [w1548]
          tunnel: [w1558] -> w1524
          tunnel: [w1557] -> w1523
          tunnel: w1522 -> [w1556]
          tunnel: w1521 -> [w1555]
          tunnel: [w1564] -> w1513
          tunnel: [w1565] -> w1514
          tunnel: w1524 -> [w1565]
          tunnel: w1523 -> [w1563]
          frame #0 {
            n860 = property on="X Go" class="Bool"("DisabledEnum"=T2."Disabled and Grayed Out" ("Disabled")) -> ()  [unwired: 2 in, 2 out]
            n861 = property on="Scan Go" class="Bool"("DisabledEnum"=T2."Disabled and Grayed Out" ("Disabled")) -> ()  [unwired: 2 in, 2 out]
          }
          frame #1 {
            n862 = property on="X Step SP" class="DigNum (strict)"() -> ("Value"=w1541:i32)  [unwired: 2 in, 2 out]
            n863 = property on="X Step PV" class="DigNum (strict)"() -> ("Value"=w1540:i32)  [unwired: 2 in, 2 out]
            n864 = property on="X Backlash" class="DigNum (strict)"() -> ("Value"=w1529:i32)  [unwired: 2 in, 2 out]
            n865 = Subtract(x=w1541, y=w1540) -> (x-y=w1539:i32)
            n866 = Sign(1:w1529) -> (0:w1537:i32)
            n867 = Sign(1:w1539) -> (0:w1538:i32)
            n868 = Multiply(x=w1538, y=w1537) -> (x*y=w1536:i32)
            n869 = Equal?(x=w1536, y=1) -> (x = y?=w1534:bool)
            n870 = case shown="True" w1534 {
              tunnel: w1533 -> [w1544 w1546]
              tunnel: w1532 -> [w1543 w1545]
              tunnel: [w1543 w1545] -> w1531
              tunnel: [w1544 w1546] -> w1530
              frame #0 {
                n871 = property on="X Backlash corr" class="Bool (strict)"("Val(Sgnl)"=FALSE ("Value (Signaling)")) -> ()  [unwired: 2 in, 2 out]
              }
              frame #1 {
                n872 = property on="X Backlash corr" class="Bool (strict)"("Val(Sgnl)"=TRUE ("Value (Signaling)")) -> ()  [unwired: 2 in, 2 out]
              }
            }
          }
          frame #2 {
            # "Velocity Setting"
            n873 = property on="X Velocity SP step/sec" class="DigNum (strict)"() -> ("Value"=w1552:i32)  [unwired: 2 in, 2 out]
            n874 = Number To Decimal String(number=w1552) -> (decimal integer string=w1553:string)  [unwired: 1 in]
            n875 = call "mDrive Send Command.vi"("error in (no error)"=w1549, "Extra"=w1553, "Command"=T1."Max Velocity", "VISA resource name"=w1548) -> ("error out"=w1550:errorcluster, "VISA resource name out"=w1551:refnum<visa-resource-name>)  [unwired: 3 in, 1 out]
          }
          frame #3 {
            # "Move to Abs Position"
            n876 = property on="X Step SP" class="DigNum (strict)"() -> ("Value"=w1561:i32)  [unwired: 2 in, 2 out]
            n877 = Number To Decimal String(number=w1561) -> (decimal integer string=w1560:string)  [unwired: 1 in]
            n878 = call "mDrive Send Command.vi"("error in (no error)"=w1555, "Extra"=w1560, "Command"=T1."Move to Absolute Position", "VISA resource name"=w1556) -> ("error out"=w1557:errorcluster, "VISA resource name out"=w1558:refnum<visa-resource-name>)  [unwired: 3 in, 1 out]
          }
          frame #4 {
            n879 = call "Time Delay15"("error in (no error)"=w1563, "Delay Time (s)"=0.1) -> ("error out"=w1564:errorcluster)  [unwired: 9 in]
          }
        }
      }
      event #16 {
        n880 = event-data() -> ()  [unwired: 1 in, 7 out]
        n881 = flat-sequence {
          tunnel: [w1581] -> w1573
          tunnel: [w1579] -> w1572
          tunnel: w1571 -> [w1575]
          tunnel: w1570 -> [w1574]
          tunnel: w1573 -> [w1596]
          tunnel: w1572 -> [w1595]
          tunnel: [w1596] -> w1567
          tunnel: [w1595] -> w1566
          tunnel: [w1598] -> w1568
          tunnel: [w1599] -> w1569
          tunnel: w1567 -> [w1599]
          tunnel: w1566 -> [w1598]
          frame #0 {
            # "VELOCITY"
            n882 = property on="X Scan Velocity SP steps/sec" class="DigNum (strict)"() -> ("Value"=w1582:i32)  [unwired: 2 in, 2 out]
            n883 = Number To Decimal String(number=w1582) -> (decimal integer string=w1583:string)  [unwired: 1 in]
            n884 = call "mDrive Send Command.vi"("error in (no error)"=w1574, "Extra"=w1583, "Command"=T1."Max Velocity", "VISA resource name"=w1575) -> ("error out"=w1584:errorcluster, "VISA resource name out"=w1589:refnum<visa-resource-name>)  [unwired: 3 in, 1 out]
            n885 = call "Time Delay9"("error in (no error)"=w1584) -> ("error out"=w1587:errorcluster)  [unwired: 10 in]
            n886 = call "mDrive Send Command.vi"("error in (no error)"=w1587, "Extra"="VM", "Command"=T1."Print Parameter", "VISA resource name"=w1589) -> ("error out"=w1580:errorcluster, "read buffer"=w1585:string, "VISA resource name out"=w1581:refnum<visa-resource-name>)  [unwired: 3 in]
            n887 = call "Time Delay10"("error in (no error)"=w1580) -> ("error out"=w1579:errorcluster)  [unwired: 10 in]
            n888 = Decimal String To Number(string=w1585, offset=0) -> (number=w1588:i32)  [unwired: 1 in, 1 out]
            n889 = property on="X velocity PV step/sec" class="DigNum (strict)"("Val(Sgnl)"=w1588) -> ()  [unwired: 2 in, 2 out]
          }
          frame #1 {
            n890 = property on="X Scan" class="Bool (strict)"("Val(Sgnl)"=TRUE ("Slew Ready 2")) -> ()  [unwired: 2 in, 2 out]
            n891 = property on="Scan Cancel" class="Bool"("DisabledEnum"=T2."Enabled" ("Disabled")) -> ()  [unwired: 2 in, 2 out]
            n892 = property on="Scan Go" class="Bool"("DisabledEnum"=T2."Enabled" ("Disabled")) -> ()  [unwired: 2 in, 2 out]
            n893 = property on="X Scan Length SP steps" class="DigNum (strict)"("DisabledEnum"=T2."Disabled and Grayed Out" ("Disabled")) -> ()  [unwired: 2 in, 2 out]
            n894 = property on="X Scan Velocity SP steps/sec" class="DigNum (strict)"("DisabledEnum"=T2."Disabled and Grayed Out" ("Disabled")) -> ()  [unwired: 2 in, 2 out]
          }
          frame #2 {
            n895 = property on="X Go" class="Bool"("DisabledEnum"=T2."Disabled and Grayed Out" ("Disabled")) -> ()  [unwired: 2 in, 2 out]
          }
        }
      }
      event #17 {
        n896 = event-data() -> ()  [unwired: 1 in, 7 out]
        n897 = flat-sequence {
          tunnel: w1607 -> [w1617]
          tunnel: w1606 -> [w1616]
          tunnel: [w1613] -> w1604
          tunnel: [w1611] -> w1603
          tunnel: w1604 -> [w1630]
          tunnel: w1603 -> [w1629]
          tunnel: [w1630] -> w1601
          tunnel: [w1629] -> w1600
          tunnel: [w1632] -> w1605
          tunnel: [w1633] -> w1602
          tunnel: w1601 -> [w1633]
          tunnel: w1600 -> [w1632]
          frame #0 {
            # "VELOCITY"
            n898 = property on="Y Scan Velocity SP steps/sec" class="DigNum (strict)"() -> ("Value"=w1614:i32)  [unwired: 2 in, 2 out]
            n899 = Number To Decimal String(number=w1614) -> (decimal integer string=w1615:string)  [unwired: 1 in]
            n900 = call "mDrive Send Command.vi"("error in (no error)"=w1617, "Extra"=w1615, "Command"=T1."Max Velocity", "VISA resource name"=w1616) -> ("error out"=w1618:errorcluster, "VISA resource name out"=w1623:refnum<visa-resource-name>)  [unwired: 3 in, 1 out]
            n901 = call "Time Delay5"("error in (no error)"=w1618) -> ("error out"=w1621:errorcluster)  [unwired: 10 in]
            n902 = call "mDrive Send Command.vi"("error in (no error)"=w1621, "Extra"="VM", "Command"=T1."Print Parameter", "VISA resource name"=w1623) -> ("error out"=w1612:errorcluster, "read buffer"=w1619:string, "VISA resource name out"=w1613:refnum<visa-resource-name>)  [unwired: 3 in]
            n903 = Decimal String To Number(string=w1619, offset=0) -> (number=w1622:i32)  [unwired: 1 in, 1 out]
            n904 = property on="Y velocity PV step/sec" class="DigNum (strict)"("Val(Sgnl)"=w1622) -> ()  [unwired: 2 in, 2 out]
            n905 = call "Time Delay6"("error in (no error)"=w1612) -> ("error out"=w1611:errorcluster)  [unwired: 10 in]
          }
          frame #1 {
            n906 = property on="Y Scan" class="Bool (strict)"("Val(Sgnl)"=TRUE ("Slew Ready 2")) -> ()  [unwired: 2 in, 2 out]
            n907 = property on="Scan Cancel" class="Bool"("DisabledEnum"=T2."Enabled" ("Disabled")) -> ()  [unwired: 2 in, 2 out]
            n908 = property on="Scan Go" class="Bool"("DisabledEnum"=T2."Enabled" ("Disabled")) -> ()  [unwired: 2 in, 2 out]
            n909 = property on="Y Scan Length SP steps" class="DigNum (strict)"("DisabledEnum"=T2."Disabled and Grayed Out" ("Disabled")) -> ()  [unwired: 2 in, 2 out]
            n910 = property on="Y Scan Velocity SP steps/sec" class="DigNum (strict)"("DisabledEnum"=T2."Disabled and Grayed Out" ("Disabled")) -> ()  [unwired: 2 in, 2 out]
          }
          frame #2 {
            n911 = property on="Y Go" class="Bool"("DisabledEnum"=T2."Disabled and Grayed Out" ("Disabled")) -> ()  [unwired: 2 in, 2 out]
          }
        }
      }
      event #18 {
        n912 = event-data() -> ()  [unwired: 1 in, 7 out]
        n913 = flat-sequence {
          tunnel: [w1649] -> w1641
          tunnel: [w1647] -> w1640
          tunnel: w1637 -> [w1643]
          tunnel: w1636 -> [w1642]
          tunnel: w1641 -> [w1664]
          tunnel: w1640 -> [w1663]
          tunnel: [w1664] -> w1639
          tunnel: [w1663] -> w1638
          tunnel: [w1666] -> w1635
          tunnel: [w1667] -> w1634
          tunnel: w1639 -> [w1667]
          tunnel: w1638 -> [w1666]
          frame #0 {
            # "VELOCITY"
            n914 = property on="Z Scan Velocity SP steps/sec" class="DigNum (strict)"() -> ("Value"=w1650:i32)  [unwired: 2 in, 2 out]
            n915 = Number To Decimal String(number=w1650) -> (decimal integer string=w1651:string)  [unwired: 1 in]
            n916 = call "mDrive Send Command.vi"("error in (no error)"=w1642, "Extra"=w1651, "Command"=T1."Max Velocity", "VISA resource name"=w1643) -> ("error out"=w1652:errorcluster, "VISA resource name out"=w1657:refnum<visa-resource-name>)  [unwired: 3 in, 1 out]
            n917 = call "Time Delay24"("error in (no error)"=w1652) -> ("error out"=w1655:errorcluster)  [unwired: 10 in]
            n918 = call "mDrive Send Command.vi"("error in (no error)"=w1655, "Extra"="VM", "Command"=T1."Print Parameter", "VISA resource name"=w1657) -> ("error out"=w1648:errorcluster, "read buffer"=w1653:string, "VISA resource name out"=w1649:refnum<visa-resource-name>)  [unwired: 3 in]
            n919 = Decimal String To Number(string=w1653, offset=0) -> (number=w1656:i32)  [unwired: 1 in, 1 out]
            n920 = property on="Z  velocity PV step/sec" class="DigNum (strict)"("Val(Sgnl)"=w1656) -> ()  [unwired: 2 in, 2 out]
            n921 = call "Time Delay25"("error in (no error)"=w1648) -> ("error out"=w1647:errorcluster)  [unwired: 10 in]
          }
          frame #1 {
            n922 = property on="Z Scan" class="Bool (strict)"("Val(Sgnl)"=TRUE ("Slew Ready 2")) -> ()  [unwired: 2 in, 2 out]
            n923 = property on="Scan Cancel" class="Bool"("DisabledEnum"=T2."Enabled" ("Disabled")) -> ()  [unwired: 2 in, 2 out]
            n924 = property on="Scan Go" class="Bool"("DisabledEnum"=T2."Enabled" ("Disabled")) -> ()  [unwired: 2 in, 2 out]
            n925 = property on="Z Scan Length SP steps" class="DigNum (strict)"("DisabledEnum"=T2."Disabled and Grayed Out" ("Disabled")) -> ()  [unwired: 2 in, 2 out]
            n926 = property on="Z Scan Velocity SP steps/sec" class="DigNum (strict)"("DisabledEnum"=T2."Disabled and Grayed Out" ("Disabled")) -> ()  [unwired: 2 in, 2 out]
          }
          frame #2 {
            n927 = property on="Z Go" class="Bool"("DisabledEnum"=T2."Disabled and Grayed Out" ("Disabled")) -> ()  [unwired: 2 in, 2 out]
          }
        }
      }
      event #19 {
        n928 = event-data() -> ()  [unwired: 1 in, 7 out]
        n929 = flat-sequence {
          tunnel: [w1683] -> w1675
          tunnel: [w1681] -> w1674
          tunnel: w1671 -> [w1677]
          tunnel: w1670 -> [w1676]
          tunnel: w1675 -> [w1698]
          tunnel: w1674 -> [w1697]
          tunnel: [w1698] -> w1673
          tunnel: [w1697] -> w1672
          tunnel: [w1700] -> w1668
          tunnel: [w1701] -> w1669
          tunnel: w1673 -> [w1701]
          tunnel: w1672 -> [w1700]
          frame #0 {
            # "VELOCITY"
            n930 = property on="R Scan Velocity SP steps/sec" class="DigNum (strict)"() -> ("Value"=w1684:i32)  [unwired: 2 in, 2 out]
            n931 = Number To Decimal String(number=w1684) -> (decimal integer string=w1685:string)  [unwired: 1 in]
            n932 = call "mDrive Send Command.vi"("error in (no error)"=w1676, "Extra"=w1685, "Command"=T1."Max Velocity", "VISA resource name"=w1677) -> ("error out"=w1686:errorcluster, "VISA resource name out"=w1691:refnum<visa-resource-name>)  [unwired: 3 in, 1 out]
            n933 = call "Time Delay26"("error in (no error)"=w1686) -> ("error out"=w1689:errorcluster)  [unwired: 10 in]
            n934 = call "mDrive Send Command.vi"("error in (no error)"=w1689, "Extra"="VM", "Command"=T1."Print Parameter", "VISA resource name"=w1691) -> ("error out"=w1682:errorcluster, "read buffer"=w1687:string, "VISA resource name out"=w1683:refnum<visa-resource-name>)  [unwired: 3 in]
            n935 = Decimal String To Number(string=w1687, offset=0) -> (number=w1690:i32)  [unwired: 1 in, 1 out]
            n936 = property on="R velocity PV step/sec" class="DigNum (strict)"("Val(Sgnl)"=w1690) -> ()  [unwired: 2 in, 2 out]
            n937 = call "Time Delay27"("error in (no error)"=w1682) -> ("error out"=w1681:errorcluster)  [unwired: 10 in]
          }
          frame #1 {
            n938 = property on="R Scan" class="Bool (strict)"("Val(Sgnl)"=TRUE ("Slew Ready 2")) -> ()  [unwired: 2 in, 2 out]
            n939 = property on="Scan Cancel" class="Bool"("DisabledEnum"=T2."Enabled" ("Disabled")) -> ()  [unwired: 2 in, 2 out]
            n940 = property on="Scan Go" class="Bool"("DisabledEnum"=T2."Enabled" ("Disabled")) -> ()  [unwired: 2 in, 2 out]
            n941 = property on="R Scan Length SP steps" class="DigNum (strict)"("DisabledEnum"=T2."Disabled and Grayed Out" ("Disabled")) -> ()  [unwired: 2 in, 2 out]
            n942 = property on="R Scan Velocity SP steps/sec" class="DigNum (strict)"("DisabledEnum"=T2."Disabled and Grayed Out" ("Disabled")) -> ()  [unwired: 2 in, 2 out]
          }
          frame #2 {
            n943 = property on="R Go" class="Bool"("DisabledEnum"=T2."Disabled and Grayed Out" ("Disabled")) -> ()  [unwired: 2 in, 2 out]
          }
        }
      }
      event #20 {
        n944 = event-data() -> ()  [unwired: 1 in, 4 out]
        n945 = event-data() -> ()  [unwired: 3 in, 1 out]
      }
      event #21 {
        n946 = event-data() -> ()  [unwired: 1 in, 7 out]
        n947 = flat-sequence {
          tunnel: [w1734] -> w1716
          tunnel: [w1733] -> w1715
          tunnel: w1714 -> [w1732]
          tunnel: w1713 -> [w1731]
          frame #0 {
            n948 = call "mDrive Send Command.vi"("error in (no error)"=w1731, "Command"=T1."Stop", "VISA resource name"=w1732) -> ("error out"=w1733:errorcluster, "VISA resource name out"=w1734:refnum<visa-resource-name>)  [unwired: 4 in, 1 out]
          }
        }
        n949 = flat-sequence {
          tunnel: [w1729] -> w1710
          tunnel: [w1728] -> w1709
          tunnel: w1712 -> [w1727]
          tunnel: w1711 -> [w1726]
          frame #0 {
            n950 = call "mDrive Send Command.vi"("error in (no error)"=w1726, "Command"=T1."Stop", "VISA resource name"=w1727) -> ("error out"=w1728:errorcluster, "VISA resource name out"=w1729:refnum<visa-resource-name>)  [unwired: 4 in, 1 out]
          }
        }
        n951 = flat-sequence {
          tunnel: w1720 -> [w1740]
          tunnel: w1719 -> [w1739]
          tunnel: [w1738] -> w1718
          tunnel: [w1737] -> w1717
          frame #0 {
            n952 = call "mDrive Send Command.vi"("error in (no error)"=w1739, "Command"=T1."Stop", "VISA resource name"=w1740) -> ("error out"=w1737:errorcluster, "VISA resource name out"=w1738:refnum<visa-resource-name>)  [unwired: 4 in, 1 out]
          }
        }
        n953 = flat-sequence {
          tunnel: w1708 -> [w1725]
          tunnel: w1707 -> [w1724]
          tunnel: [w1723] -> w1706
          tunnel: [w1721] -> _
          tunnel: [w1721] -> w1705
          frame #0 {
            n954 = call "mDrive Send Command.vi"("error in (no error)"=w1724, "Command"=T1."Stop", "VISA resource name"=w1725) -> ("error out"=w1721:errorcluster, "VISA resource name out"=w1723:refnum<visa-resource-name>)  [unwired: 4 in, 1 out]
          }
        }
      }
      event #22 {
        n955 = event-data() -> ()  [unwired: 1 in, 7 out]
        n956 = flat-sequence {
          tunnel: w1756 -> [w1795]
          tunnel: w1755 -> [w1794]
          tunnel: [w1797] -> w1758
          tunnel: [w1796] -> w1757
          tunnel: [w1804] -> w1753
          tunnel: [w1805] -> w1754
          tunnel: w1758 -> [w1805]
          tunnel: w1757 -> [w1804]
          frame #0 {
            n957 = call "mDrive Send Command.vi"("error in (no error)"=w1794, "Command"=T1."Stop", "VISA resource name"=w1795) -> ("error out"=w1796:errorcluster, "VISA resource name out"=w1797:refnum<visa-resource-name>)  [unwired: 4 in, 1 out]
          }
          frame #1 {
            n958 = property on="X Scan" class="Bool (strict)"("Value"=FALSE ("Slew Ready")) -> ()  [unwired: 2 in, 2 out]
            n959 = property on="X Scan set" class="Bool"("DisabledEnum"=T2."Enabled" ("Disabled")) -> ()  [unwired: 2 in, 2 out]
            n960 = property on="X Scan Velocity SP steps/sec" class="DigNum (strict)"("DisabledEnum"=T2."Enabled" ("Disabled")) -> ()  [unwired: 2 in, 2 out]
            n961 = property on="X Scan Length SP steps" class="DigNum (strict)"("DisabledEnum"=T2."Enabled" ("Disabled")) -> ()  [unwired: 2 in, 2 out]
            n962 = property on="X Go" class="Bool"("DisabledEnum"=T2."Enabled" ("Disabled")) -> ()  [unwired: 2 in, 2 out]
            n963 = property on="X Scan OK" class="Bool"("DisabledEnum"=T2."Enabled" ("Disabled")) -> ()  [unwired: 2 in, 2 out]
          }
        }
        n964 = flat-sequence {
          tunnel: [w1784] -> w1752
          tunnel: [w1783] -> w1751
          tunnel: w1750 -> [w1781]
          tunnel: w1749 -> [w1780]
          tunnel: [w1791] -> w1747
          tunnel: [w1792] -> w1748
          tunnel: w1752 -> [w1792]
          tunnel: w1751 -> [w1791]
          frame #0 {
            n965 = call "mDrive Send Command.vi"("error in (no error)"=w1780, "Command"=T1."Stop", "VISA resource name"=w1781) -> ("error out"=w1783:errorcluster, "VISA resource name out"=w1784:refnum<visa-resource-name>)  [unwired: 4 in, 1 out]
          }
          frame #1 {
            n966 = property on="Z Scan" class="Bool (strict)"("Value"=FALSE ("Slew Ready")) -> ()  [unwired: 2 in, 2 out]
            n967 = property on="Z Scan set" class="Bool"("DisabledEnum"=T2."Enabled" ("Disabled")) -> ()  [unwired: 2 in, 2 out]
            n968 = property on="Z Scan Velocity SP steps/sec" class="DigNum (strict)"("DisabledEnum"=T2."Enabled" ("Disabled")) -> ()  [unwired: 2 in, 2 out]
            n969 = property on="Z Scan Length SP steps" class="DigNum (strict)"("DisabledEnum"=T2."Enabled" ("Disabled")) -> ()  [unwired: 2 in, 2 out]
            n970 = property on="Z Go" class="Bool"("DisabledEnum"=T2."Enabled" ("Disabled")) -> ()  [unwired: 2 in, 2 out]
            n971 = property on="Z Scan OK" class="Bool"("DisabledEnum"=T2."Enabled" ("Disabled")) -> ()  [unwired: 2 in, 2 out]
          }
        }
        n972 = flat-sequence {
          tunnel: w1764 -> [w1808]
          tunnel: w1763 -> [w1807]
          tunnel: [w1810] -> w1760
          tunnel: [w1809] -> w1759
          tunnel: [w1817] -> w1765
          tunnel: [w1818] -> w1766
          tunnel: w1760 -> [w1818]
          tunnel: w1759 -> [w1817]
          frame #0 {
            n973 = call "mDrive Send Command.vi"("error in (no error)"=w1807, "Command"=T1."Stop", "VISA resource name"=w1808) -> ("error out"=w1809:errorcluster, "VISA resource name out"=w1810:refnum<visa-resource-name>)  [unwired: 4 in, 1 out]
          }
          frame #1 {
            n974 = property on="Y Scan" class="Bool (strict)"("Value"=FALSE ("Slew Ready")) -> ()  [unwired: 2 in, 2 out]
            n975 = property on="Y Go" class="Bool"("DisabledEnum"=T2."Enabled" ("Disabled")) -> ()  [unwired: 2 in, 2 out]
            n976 = property on="Y Scan Velocity SP steps/sec" class="DigNum (strict)"("DisabledEnum"=T2."Enabled" ("Disabled")) -> ()  [unwired: 2 in, 2 out]
            n977 = property on="Y Scan set" class="Bool"("DisabledEnum"=T2."Enabled" ("Disabled")) -> ()  [unwired: 2 in, 2 out]
            n978 = property on="Y Scan OK" class="Bool"("DisabledEnum"=T2."Enabled" ("Disabled")) -> ()  [unwired: 2 in, 2 out]
            n979 = property on="Y Scan Length SP steps" class="DigNum (strict)"("DisabledEnum"=T2."Enabled" ("Disabled")) -> ()  [unwired: 2 in, 2 out]
          }
        }
        n980 = flat-sequence {
          tunnel: [w1771] -> w1746
          tunnel: [w1770] -> w1745
          tunnel: w1744 -> [w1768]
          tunnel: w1743 -> [w1767]
          tunnel: [w1778] -> w1741
          tunnel: [w1779] -> w1742
          tunnel: w1746 -> [w1779]
          tunnel: w1745 -> [w1778]
          frame #0 {
            n981 = call "mDrive Send Command.vi"("error in (no error)"=w1767, "Command"=T1."Stop", "VISA resource name"=w1768) -> ("error out"=w1770:errorcluster, "VISA resource name out"=w1771:refnum<visa-resource-name>)  [unwired: 4 in, 1 out]
          }
          frame #1 {
            n982 = property on="R Scan" class="Bool (strict)"("Value"=FALSE ("Slew Ready")) -> ()  [unwired: 2 in, 2 out]
            n983 = property on="R Scan Velocity SP steps/sec" class="DigNum (strict)"("DisabledEnum"=T2."Enabled" ("Disabled")) -> ()  [unwired: 2 in, 2 out]
            n984 = property on="R Go" class="Bool"("DisabledEnum"=T2."Enabled" ("Disabled")) -> ()  [unwired: 2 in, 2 out]
            n985 = property on="R Scan OK" class="Bool"("DisabledEnum"=T2."Enabled" ("Disabled")) -> ()  [unwired: 2 in, 2 out]
            n986 = property on="R Scan Length SP steps" class="DigNum (strict)"("DisabledEnum"=T2."Enabled" ("Disabled")) -> ()  [unwired: 2 in, 2 out]
            n987 = property on="R Scan set" class="Bool"("DisabledEnum"=T2."Enabled" ("Disabled")) -> ()  [unwired: 2 in, 2 out]
          }
        }
        n988 = property on="Scan Go" class="Bool"("DisabledEnum"=T2."Disabled and Grayed Out" ("Disabled")) -> ()  [unwired: 2 in, 2 out]
        n989 = property on="Scan Cancel" class="Bool"("DisabledEnum"=T2."Disabled and Grayed Out" ("Disabled")) -> ()  [unwired: 2 in, 2 out]
      }
      event #23 {
        n990 = event-data() -> ()  [unwired: 1 in, 7 out]
        n991 = flat-sequence {
          tunnel: [w1898] -> w1882
          tunnel: [w1896] -> w1875
          tunnel: [w1897] -> w1872
          tunnel: [w1891] -> w1871
          tunnel: [w1895] -> w1870
          tunnel: [w1894] -> w1869
          tunnel: [w1893] -> w1868
          tunnel: [w1892] -> w1867
          tunnel: w1846 -> [w1890]
          tunnel: [w1890] -> w1845
          tunnel: w1844 -> [w1889]
          tunnel: [w1889] -> w1843
          tunnel: w1842 -> [w1888]
          tunnel: [w1888] -> w1841
          tunnel: w1840 -> [w1887]
          tunnel: [w1887] -> w1839
          tunnel: w1838 -> [w1886]
          tunnel: [w1886] -> w1837
          tunnel: w1836 -> [w1885]
          tunnel: [w1885] -> w1835
          tunnel: [w1884] -> w1834
          tunnel: w1833 -> [w1884]
          tunnel: [w1883] -> w1832
          tunnel: w1831 -> [w1883]
          tunnel: [w1950] -> w1879
          tunnel: [w1949] -> w1877
          tunnel: w1882 -> [w1948]
          tunnel: w1875 -> [w1947]
          tunnel: [w1947] -> w1873
          tunnel: w1872 -> [w1946]
          tunnel: w1871 -> [w1935]
          tunnel: w1870 -> [w1945]
          tunnel: w1869 -> [w1941]
          tunnel: w1868 -> [w1938]
          tunnel: w1867 -> [w1944]
          tunnel: [w1943] -> w1865
          tunnel: [w1942] -> w1863
          tunnel: [w1941] -> w1860
          tunnel: [w1940] -> w1858
          tunnel: [w1939] -> w1856
          tunnel: [w1938] -> w1854
          tunnel: [w1937] -> w1852
          tunnel: [w1936] -> w1850
          tunnel: [w1935] -> w1849
          tunnel: w1845 -> [w1934]
          tunnel: w1843 -> [w1933]
          tunnel: w1841 -> [w1932]
          tunnel: w1839 -> [w1931]
          tunnel: w1837 -> [w1930]
          tunnel: w1835 -> [w1929]
          tunnel: w1834 -> [w1928]
          tunnel: w1832 -> [w1927]
          tunnel: w1879 -> [w1991]
          tunnel: [w1991] -> w1878
          tunnel: w1877 -> [w1990]
          tunnel: [w1990] -> w1876
          tunnel: [w1988] -> w1874
          tunnel: w1873 -> [w1988]
          tunnel: [w1987] -> w1866
          tunnel: w1865 -> [w1987]
          tunnel: [w1986] -> w1864
          tunnel: w1863 -> [w1986]
          tunnel: [w1985] -> w1862
          tunnel: [w1984] -> w1861
          tunnel: w1860 -> [w1984]
          tunnel: [w1983] -> w1859
          tunnel: w1858 -> [w1983]
          tunnel: [w1982] -> w1857
          tunnel: w1856 -> [w1982]
          tunnel: [w1981] -> w1855
          tunnel: w1854 -> [w1981]
          tunnel: [w1980] -> w1853
          tunnel: w1852 -> [w1980]
          tunnel: [w1979] -> w1851
          tunnel: w1850 -> [w1979]
          tunnel: w1849 -> [w1985]
          tunnel: w1878 -> [w2011]
          tunnel: [w2009] -> w1881
          tunnel: w1876 -> [w2010]
          tunnel: [w2008] -> w1880
          tunnel: w1874 -> [w2007]
          tunnel: w1866 -> [w2006]
          tunnel: w1864 -> [w2005]
          tunnel: w1862 -> [w2004]
          tunnel: w1861 -> [w2003]
          tunnel: w1859 -> [w2002]
          tunnel: w1857 -> [w2001]
          tunnel: w1855 -> [w2000]
          tunnel: w1853 -> [w1999]
          tunnel: w1851 -> [w1998]
          tunnel: [w1997] -> w1848
          tunnel: [w1996] -> w1847
          tunnel: [w1995] -> w1826
          tunnel: [w1994] -> w1823
          tunnel: [w1993] -> w1821
          tunnel: [w1992] -> w1819
          tunnel: w1881 -> [w2069]
          tunnel: w1880 -> [w2068]
          tunnel: [w2069] -> w1830
          tunnel: [w2068] -> w1829
          tunnel: [w2062] -> w1828
          tunnel: w1848 -> [w2062]
          tunnel: [w2061] -> w1827
          tunnel: w1847 -> [w2061]
          tunnel: w1826 -> [w2051]
          tunnel: [w2051] -> w1825
          tunnel: [w2050] -> w1824
          tunnel: w1823 -> [w2050]
          tunnel: [w2049] -> w1822
          tunnel: w1821 -> [w2049]
          tunnel: [w2048] -> w1820
          tunnel: w1819 -> [w2048]
          frame #0 {
            n992 = property on="X Scan" class="Bool (strict)"() -> ("Value"=w1891:bool)  [unwired: 2 in, 2 out]
            n993 = property on="Z Scan" class="Bool (strict)"() -> ("Value"=w1893:bool)  [unwired: 2 in, 2 out]
            n994 = property on="Y Scan" class="Bool (strict)"() -> ("Value"=w1896:bool)  [unwired: 2 in, 2 out]
            n995 = property on="R Scan" class="Bool (strict)"() -> ("Value"=w1894:bool)  [unwired: 2 in, 2 out]
            n996 = case shown="True" w1891 {
              tunnel: ["" w1914] -> w1897
              frame #0 {
              }
              frame #1 {
                n997 = property on="X Scan Length SP steps" class="DigNum (strict)"() -> ("Value"=w1919:i32)  [unwired: 2 in, 2 out]
                n998 = Number To Decimal String(number=w1919) -> (decimal integer string=w1916:string)  [unwired: 1 in]
                n999 = call <vilib>:"Space Constant.vi"() -> ("String"=w1917:string)
                n1000 = Concatenate Strings("MR", w1917, w1916, "\r") -> (w1914:string)
              }
            }
            n1001 = case shown="True" w1893 {
              tunnel: ["" w1907] -> w1895
              frame #0 {
              }
              frame #1 {
                n1002 = property on="Z Scan Length SP steps" class="DigNum (strict)"() -> ("Value"=w1912:i32)  [unwired: 2 in, 2 out]
                n1003 = Number To Decimal String(number=w1912) -> (decimal integer string=w1909:string)  [unwired: 1 in]
                n1004 = call <vilib>:"Space Constant.vi"() -> ("String"=w1910:string)
                n1005 = Concatenate Strings("MR", w1910, w1909, "\r") -> (w1907:string)
              }
            }
            n1006 = case shown="True" w1896 {
              tunnel: ["" w1921] -> w1898
              frame #0 {
              }
              frame #1 {
                n1007 = property on="Y Scan Length SP steps" class="DigNum (strict)"() -> ("Value"=w1926:i32)  [unwired: 2 in, 2 out]
                n1008 = Number To Decimal String(number=w1926) -> (decimal integer string=w1923:string)  [unwired: 1 in]
                n1009 = call <vilib>:"Space Constant.vi"() -> ("String"=w1924:string)
                n1010 = Concatenate Strings("MR", w1924, w1923, "\r") -> (w1921:string)
              }
            }
            n1011 = case shown="True" w1894 {
              tunnel: ["" w1900] -> w1892
              frame #0 {
              }
              frame #1 {
                n1012 = property on="R Scan Length SP steps" class="DigNum (strict)"() -> ("Value"=w1905:i32)  [unwired: 2 in, 2 out]
                n1013 = Number To Decimal String(number=w1905) -> (decimal integer string=w1902:string)  [unwired: 1 in]
                n1014 = call <vilib>:"Space Constant.vi"() -> ("String"=w1903:string)
                n1015 = Concatenate Strings("MR", w1903, w1902, "\r") -> (w1900:string)
              }
            }
          }
          frame #1 {
            n1016 = case shown="False" w1935 {
              tunnel: [w1966 w1971] -> w1943
              tunnel: [w1965 w1970] -> w1942
              tunnel: w1946 -> [_ w1969]
              tunnel: w1934 -> [w1966 w1968]
              tunnel: w1933 -> [w1965 w1967]
              frame #0 {
              }
              frame #1 {
                n1017 = VISA Write(VISA resource name=w1968, write buffer=w1969, error in (no error)=w1967) -> (VISA resource name out=w1971:refnum<visa-resource-name>, error out=w1970:errorcluster)  [unwired: 1 out]
              }
            }
            n1018 = case shown="False" w1938 {
              tunnel: [w1959 w1964] -> w1937
              tunnel: [w1958 w1963] -> w1936
              tunnel: w1945 -> [_ w1962]
              tunnel: w1930 -> [w1959 w1961]
              tunnel: w1929 -> [w1958 w1960]
              frame #0 {
              }
              frame #1 {
                n1019 = VISA Write(VISA resource name=w1961, write buffer=w1962, error in (no error)=w1960) -> (VISA resource name out=w1964:refnum<visa-resource-name>, error out=w1963:errorcluster)  [unwired: 1 out]
              }
            }
            n1020 = case shown="False" w1947 {
              tunnel: [w1973 w1978] -> w1950
              tunnel: [w1972 w1977] -> w1949
              tunnel: w1948 -> [_ w1976]
              tunnel: w1932 -> [w1973 w1975]
              tunnel: w1931 -> [w1972 w1974]
              frame #0 {
              }
              frame #1 {
                n1021 = VISA Write(VISA resource name=w1975, write buffer=w1976, error in (no error)=w1974) -> (VISA resource name out=w1978:refnum<visa-resource-name>, error out=w1977:errorcluster)  [unwired: 1 out]
              }
            }
            n1022 = case shown="False" w1941 {
              tunnel: [w1952 w1957] -> w1940
              tunnel: [w1951 w1956] -> w1939
              tunnel: w1944 -> [_ w1955]
              tunnel: w1928 -> [w1952 w1954]
              tunnel: w1927 -> [w1951 w1953]
              frame #0 {
              }
              frame #1 {
                n1023 = VISA Write(VISA resource name=w1954, write buffer=w1955, error in (no error)=w1953) -> (VISA resource name out=w1957:refnum<visa-resource-name>, error out=w1956:errorcluster)  [unwired: 1 out]
              }
            }
          }
          frame #2 {
            n1024 = call "Time Delay7"("Delay Time (s)"=0.1) -> ()  [unwired: 10 in, 1 out]
          }
          frame #3 {
            n1025 = case shown="True" w2004 {
              tunnel: w2006 -> [w2031 w2035]
              tunnel: w2005 -> [w2030 w2034]
              tunnel: [w2031 w2033] -> w1993
              tunnel: [w2030 w2032] -> w1992
              frame #0 {
              }
              frame #1 {
                n1026 = property class="Instr"(reference=w2035, error in=w2034) -> (reference out=w2037:refnum<visa-resource-name>, error out=w2036:errorcluster, "Serial Settings:Number of Bytes at Serial Port"=w2038:u32)
                n1027 = VISA Read(VISA resource name=w2037, byte count=w2038, error in (no error)=w2036) -> (VISA resource name out=w2033:refnum<visa-resource-name>, error out=w2032:errorcluster)  [unwired: 2 out]
              }
            }
            n1028 = case shown="True" w2000 {
              tunnel: w1999 -> [w2013 w2017]
              tunnel: w1998 -> [w2012 w2016]
              tunnel: [w2013 w2015] -> w1997
              tunnel: [w2012 w2014] -> w1996
              frame #0 {
              }
              frame #1 {
                n1029 = property class="Instr"(reference=w2017, error in=w2016) -> (reference out=w2019:refnum<visa-resource-name>, error out=w2018:errorcluster, "Serial Settings:Number of Bytes at Serial Port"=w2020:u32)
                n1030 = VISA Read(VISA resource name=w2019, byte count=w2020, error in (no error)=w2018) -> (VISA resource name out=w2015:refnum<visa-resource-name>, error out=w2014:errorcluster)  [unwired: 2 out]
              }
            }
            n1031 = case shown="True" w2007 {
              tunnel: w2011 -> [w2040 w2044]
              tunnel: w2010 -> [w2039 w2043]
              tunnel: [w2040 w2042] -> w2009
              tunnel: [w2039 w2041] -> w2008
              frame #0 {
              }
              frame #1 {
                n1032 = property class="Instr"(reference=w2044, error in=w2043) -> (reference out=w2046:refnum<visa-resource-name>, error out=w2045:errorcluster, "Serial Settings:Number of Bytes at Serial Port"=w2047:u32)
                n1033 = VISA Read(VISA resource name=w2046, byte count=w2047, error in (no error)=w2045) -> (VISA resource name out=w2042:refnum<visa-resource-name>, error out=w2041:errorcluster)  [unwired: 2 out]
              }
            }
            n1034 = case shown="True" w2003 {
              tunnel: w2002 -> [w2022 w2026]
              tunnel: w2001 -> [w2021 w2025]
              tunnel: [w2022 w2024] -> w1995
              tunnel: [w2021 w2023] -> w1994
              frame #0 {
              }
              frame #1 {
                n1035 = property class="Instr"(reference=w2026, error in=w2025) -> (reference out=w2028:refnum<visa-resource-name>, error out=w2027:errorcluster, "Serial Settings:Number of Bytes at Serial Port"=w2029:u32)
                n1036 = VISA Read(VISA resource name=w2028, byte count=w2029, error in (no error)=w2027) -> (VISA resource name out=w2024:refnum<visa-resource-name>, error out=w2023:errorcluster)  [unwired: 2 out]
              }
            }
          }
          frame #4 {
            n1037 = property on="R Scan" class="Bool (strict)"("Val(Sgnl)"=FALSE ("Slew Ready 2")) -> ()  [unwired: 2 in, 2 out]
            n1038 = property on="Z Scan" class="Bool (strict)"("Val(Sgnl)"=FALSE ("Slew Ready 2")) -> ()  [unwired: 2 in, 2 out]
            n1039 = property on="X Scan" class="Bool (strict)"("Val(Sgnl)"=FALSE ("Slew Ready 2")) -> ()  [unwired: 2 in, 2 out]
            n1040 = property on="Y Scan" class="Bool (strict)"("Val(Sgnl)"=FALSE ("Slew Ready 2")) -> ()  [unwired: 2 in, 2 out]
            n1041 = property on="Z Scan Velocity SP steps/sec" class="DigNum (strict)"("DisabledEnum"=T2."Enabled" ("Disabled")) -> ()  [unwired: 2 in, 2 out]
            n1042 = property on="X Scan Length SP steps" class="DigNum (strict)"("DisabledEnum"=T2."Enabled" ("Disabled")) -> ()  [unwired: 2 in, 2 out]
            n1043 = property on="Y Scan Selocity SP steps/sec" class="DigNum (strict)"("DisabledEnum"=T2."Enabled" ("Disabled")) -> ()  [unwired: 2 in, 2 out]
            n1044 = property on="Z Scan Length SP steps" class="DigNum (strict)"("DisabledEnum"=T2."Enabled" ("Disabled")) -> ()  [unwired: 2 in, 2 out]
            n1045 = property on="Y Scan Length SP steps" class="DigNum (strict)"("DisabledEnum"=T2."Enabled" ("Disabled")) -> ()  [unwired: 2 in, 2 out]
            n1046 = property on="X Scan Velocity SP steps/sec" class="DigNum (strict)"("DisabledEnum"=T2."Enabled" ("Disabled")) -> ()  [unwired: 2 in, 2 out]
            n1047 = property on="R Scan Length SP steps" class="DigNum (strict)"("DisabledEnum"=T2."Enabled" ("Disabled")) -> ()  [unwired: 2 in, 2 out]
            n1048 = property on="R Scan Velocity SP steps/sec" class="DigNum (strict)"("DisabledEnum"=T2."Enabled" ("Disabled")) -> ()  [unwired: 2 in, 2 out]
            n1049 = property on="Scan Cancel" class="Bool"("DisabledEnum"=T2."Disabled and Grayed Out" ("Disabled")) -> ()  [unwired: 2 in, 2 out]
            n1050 = property on="Scan Go" class="Bool"("DisabledEnum"=T2."Disabled and Grayed Out" ("Disabled")) -> ()  [unwired: 2 in, 2 out]
          }
        }
      }
      event #24 {
        n1051 = event-data() -> ()  [unwired: 1 in, 7 out]
        n1052 = flat-sequence {
          tunnel: [w2100] -> w2079
          tunnel: w2080 -> [w2103]
          tunnel: [w2102] -> w2078
          tunnel: w2081 -> [w2101]
          frame #0 {
            n1053 = property on="Reset X Motor Steps" class="DigNum (strict)"() -> ("Value"=w2104:i32)  [unwired: 2 in, 2 out]
            n1054 = Number To Decimal String(number=w2104) -> (decimal integer string=w2105:string)  [unwired: 1 in]
            n1055 = call "mDrive Send Command.vi"("error in (no error)"=w2103, "Extra"=w2105, "Command"=T1."Set Current Position", "VISA resource name"=w2101) -> ("error out"=w2102:errorcluster, "VISA resource name out"=w2100:refnum<visa-resource-name>)  [unwired: 3 in, 1 out]
          }
        }
        n1056 = flat-sequence {
          tunnel: [w2087] -> w2073
          tunnel: [w2089] -> w2072
          tunnel: w2075 -> [w2088]
          tunnel: w2074 -> [w2086]
          frame #0 {
            n1057 = property on="Reset R Motor Steps" class="DigNum (strict)"() -> ("Value"=w2090:i32)  [unwired: 2 in, 2 out]
            n1058 = Number To Decimal String(number=w2090) -> (decimal integer string=w2091:string)  [unwired: 1 in]
            n1059 = call "mDrive Send Command.vi"("error in (no error)"=w2086, "Extra"=w2091, "Command"=T1."Set Current Position", "VISA resource name"=w2088) -> ("error out"=w2089:errorcluster, "VISA resource name out"=w2087:refnum<visa-resource-name>)  [unwired: 3 in, 1 out]
          }
        }
        n1060 = flat-sequence {
          tunnel: w2085 -> [w2110]
          tunnel: w2084 -> [w2109]
          tunnel: [w2108] -> w2083
          tunnel: [w2107] -> w2082
          frame #0 {
            n1061 = property on="Reset Y Motor Steps" class="DigNum (strict)"() -> ("Value"=w2111:i32)  [unwired: 2 in, 2 out]
            n1062 = Number To Decimal String(number=w2111) -> (decimal integer string=w2112:string)  [unwired: 1 in]
            n1063 = call "mDrive Send Command.vi"("error in (no error)"=w2109, "Extra"=w2112, "Command"=T1."Set Current Position", "VISA resource name"=w2110) -> ("error out"=w2107:errorcluster, "VISA resource name out"=w2108:refnum<visa-resource-name>)  [unwired: 3 in, 1 out]
          }
        }
        n1064 = flat-sequence {
          tunnel: [w2096] -> w2071
          tunnel: [w2095] -> w2070
          tunnel: w2077 -> [w2094]
          tunnel: w2076 -> [w2093]
          frame #0 {
            n1065 = property on="Reset Z Motor Steps" class="DigNum (strict)"() -> ("Value"=w2097:i32)  [unwired: 2 in, 2 out]
            n1066 = Number To Decimal String(number=w2097) -> (decimal integer string=w2098:string)  [unwired: 1 in]
            n1067 = call "mDrive Send Command.vi"("error in (no error)"=w2093, "Extra"=w2098, "Command"=T1."Set Current Position", "VISA resource name"=w2094) -> ("error out"=w2095:errorcluster, "VISA resource name out"=w2096:refnum<visa-resource-name>)  [unwired: 3 in, 1 out]
          }
        }
      }
    }
  }
  n1068 = flat-sequence {
    tunnel: w62 -> [w2118]
    tunnel: w61 -> [w2115]
    frame #0 {
      n1069 = call "mDrive Send Command.vi"("error in (no error)"=w2115, "Command"=T1."Stop", "VISA resource name"=w2118) -> ("error out"=w2116:errorcluster, "VISA resource name out"=w2117:refnum<visa-resource-name>)  [unwired: 4 in, 1 out]
      n1070 = VISA Close(VISA resource name=w2117, error in (no error)=w2116) -> ()  [unwired: 1 out]
    }
  }
  n1071 = flat-sequence {
    tunnel: w34 -> [w2123]
    tunnel: w33 -> [w2120]
    frame #0 {
      n1072 = call "mDrive Send Command.vi"("error in (no error)"=w2120, "Command"=T1."Stop", "VISA resource name"=w2123) -> ("error out"=w2121:errorcluster, "VISA resource name out"=w2122:refnum<visa-resource-name>)  [unwired: 4 in, 1 out]
      n1073 = VISA Close(VISA resource name=w2122, error in (no error)=w2121) -> ()  [unwired: 1 out]
    }
  }
  n1074 = flat-sequence {
    tunnel: w78 -> [w2128]
    tunnel: w77 -> [w2125]
    frame #0 {
      n1075 = call "mDrive Send Command.vi"("error in (no error)"=w2125, "Command"=T1."Stop", "VISA resource name"=w2128) -> ("error out"=w2126:errorcluster, "VISA resource name out"=w2127:refnum<visa-resource-name>)  [unwired: 4 in, 1 out]
      n1076 = VISA Close(VISA resource name=w2127, error in (no error)=w2126) -> ()  [unwired: 1 out]
    }
  }
  n1077 = flat-sequence {
    tunnel: w30 -> [w2133]
    tunnel: w29 -> [w2130]
    frame #0 {
      n1078 = call "mDrive Send Command.vi"("error in (no error)"=w2130, "Command"=T1."Stop", "VISA resource name"=w2133) -> ("error out"=w2131:errorcluster, "VISA resource name out"=w2132:refnum<visa-resource-name>)  [unwired: 4 in, 1 out]
      n1079 = VISA Close(VISA resource name=w2132, error in (no error)=w2131) -> ()  [unwired: 1 out]
    }
  }
